vi "mainAuto.vi"() -> ()   [LabVIEW 2018]
uses:
  <vilib>/Analysis/baseanly.llb/Mean (DBL).vi
  #include/Global_usbComm.vi
  <userlib>/_OpenG.lib/array/array.llb/Filter 1D Array with Scalar (String)__ogtk.vi
  <userlib>/_OpenG.lib/array/array.llb/Filter 1D Array with Scalar (Boolean)__ogtk.vi
  <vilib>/Analysis/NI_AALBase.lvlib
panel:
  out "index 2":i32
  out "random 2":i32
  out "random":i32
  out "index":i32
  out "appended array":i16[](array[numeric])
  out "min(x,y)":i16
  out "max(x,y)":i16
  out "valueResistance":dbl
  out "resLower":dbl
  out "resUpper":dbl
  out "resistanceArray":dbl[](array[numeric])
  out "speedArray":dbl[](array[numeric])
  out "inclineArray":dbl[](array[numeric])
  out "negative incline":dbl
  out "FAN":string
  out "fanType":string
  out "refnum out":refnum<file>
  in  "Tab Control":T1(tab)
  out "Welcome to Console Test":picture
  out "Version":string[][](array[string])
  in  "Inspection Point":string(combo)
  in  "PO Line Number":string
  in  "PO Number":string
  in  "Inspector Name":string
  in  "Work Station":string
  in  "Vendor Name":string
  in  "Vendor Number":string
  out "Initialize Test":string
  out "Config and Fixture Setup":string
  out "Firmware Reference":string
  in  "EQF1259 com port":refnum<visa-resource-name>
  out "Console Number":string
  out "Console Name":string
  in  "scanSerial":string
  out "resultSerial":bool
  out "PartNumber":string
  in  "Cos0":bool
  in  "Cos1":bool
  out "COSMETIC-3, 4":string
  in  "Con1":bool
  out "FIXTURE_SETUP-1":string
  out "Connection":picture
  out "Voltage":string
  out "Power On":cluster{dbl, dbl}(graph)
  out "Current":string
  out "POWER_UP-5, 6":string
  in  "Pow0":bool
  in  "Pow1":bool
  out "PowerOn":bool
  out "CurrentOn":bool
  out "CurrentPeak":string
  out "limitON":bool
  out "CurrentMax":string
  out "PowerMode":string="Battery"
  out "BLE_SETUP-2":string
  out "BLE_CONNECT-7":string
  out "BLE PASS":bool
  out "Cal1":bool
  in  "Dis1":bool
  in  "Dis0":bool
  out "MAINTENANCE MODE-8, 9, 10, 11":string
  in  "Enter Firmware":string
  out "Firmware":bool
  in  "Key0":bool
  in  "Key1":bool
  out "SPM AEROBIC":dbl(knob) scale=0.0..200.0
  in  "stopP":bool
  out "SPEED":dbl(knob) scale=0.0..10.1
  out "MAX":string
  out "PWM_RPM":string
  out "SPEED AEROBIC":dbl(knob) scale=0.0..25.0
  out "RPM AEROBIC":dbl(knob) scale=0.0..200.0
  in  "Tac0":bool
  in  "Tac1":bool
  out "Quickspeed":bool
  out "Minus\nButton":bool
  out "Plus\nButton":bool
  out "ONE\nButton":bool
  out "PWM PASS":bool
  out "PWM hz":string
  out "PWM %":string
  out "Elapsed Time (s)":dbl
  out "Press Next":dbl format="%#_13g"
  out "Decrease":bool
  out "Increase":bool
  out "Least":bool
  out "RESISTANCE-15":string
  out "QuickResistance":bool
  out "RESISTANCE/CURRENT":cluster{dbl, dbl}(graph)
  out "IRun":string
  out "IPeak":string
  out "Press Next":dbl
  out "RESISTANCE PASS":bool
  out "overCurrent":bool
  in  "stopR":bool
  out "currentMaxResistance":string
  out "BLE PULSE":u32(graph)
  out "BLE_BPM":u32
  out "PULSE-17":string
  out "Hand/Thumb Pass":bool
  out "BLE_HRM Pass":bool
  in  "E-stopHRM":bool
  in  "PUL0":bool
  in  "PUL1":bool
  out "BLE Status":u32
  out "FanCurrent":dbl(graph)
  in  "FAN0":bool
  in  "FAN1":bool
  out "Ifan":string
  out "limitFan":bool
  out "currentMaxFan":string
  out "FAN-18":string
  out "fanIPeak":string
  in  "AUD0 2":bool
  in  "AUD1 2":bool
  out "Iaudio":string
  out "AudioCurrent":dbl(graph)
  in  "AUD0":bool
  out "currentMaxAudio":string
  out "AUDIO-19":string
  out "audioIPeak":string
  in  "AUD1":bool
  out "limitAudio":bool
  in  "TV1":bool
  in  "TV0":bool
  out "TVCurrent":dbl(graph)
  out "Itv":string
  out "limitTV":bool
  out "currentMaxTV":string
  out "TV-20":string
  out "tvIPeak":string
  out "limitUSB":bool
  out "Iusb":string
  in  "USB1":bool
  in  "USB0":bool
  out "currentMaxUSB":string
  out "USBCurrent":dbl(graph)
  out "USB-16":string
  out "usbIPeak":string
  in  "stopI":bool
  out "incline":dbl(graph)
  out "INCLINE PASS":bool
  out "INCLINE-14":string
  out "Quickincline":bool
  out "Down":bool
  out "Up":bool
  out "ZERO":bool
  out "MAX":dbl
  out "MIN":dbl
  out "Press Next":dbl
  out "limitCSafe":bool
  out "Icsafe":string
  in  "CSA1":bool
  in  "CSA0":bool
  out "currentMaxCSafe":string
  out "CSafeCurrent":dbl(graph)
  out "CSAFE-21":string
  out "csafeIPeak":string
  out "limitWahoo":bool
  out "Iwahoo":string
  in  "WAH1":bool
  in  "WAH0":bool
  out "currentMaxWahoo":string
  out "WahooCurrent":dbl(graph)
  out "WAHOO-22":string
  out "wahooIPeak":string
  in  "ANO0":bool
  in  "ANO1":bool
  out "Another":picture
  out "# of Samples":i32
  out "# of Failed Samples":i32
  out "# of Passed Samples":i32
  out "Failed":picture
  out "Test Log":string
  out "Goodbye!":picture
  out "standard notepad":string
  out "standard labviewdbupload":string
  in  "FIN0":bool
  out "FINISH-25":string
  # "Does Cosmetic Pass Inspection?"
  # "Scan Console Serial Number"
  # "Is The Harness Connected Correctly?"
  # "Did Console Power ON?"
  # "Calibrate?"
  # "Display?"
  # "Key Code?"
  # "Did The Hand/Thumb Pulse Pass?"
  # "Did The Fan Function Well?"
  # "BLE Audio"
  # "Aux Audio"
  # "NOT USED. SEE BLE CONNECT AND PULSE FOR DATA."
  # "Would You Like To Test Another Console?"
  # "Console Failed Test!"
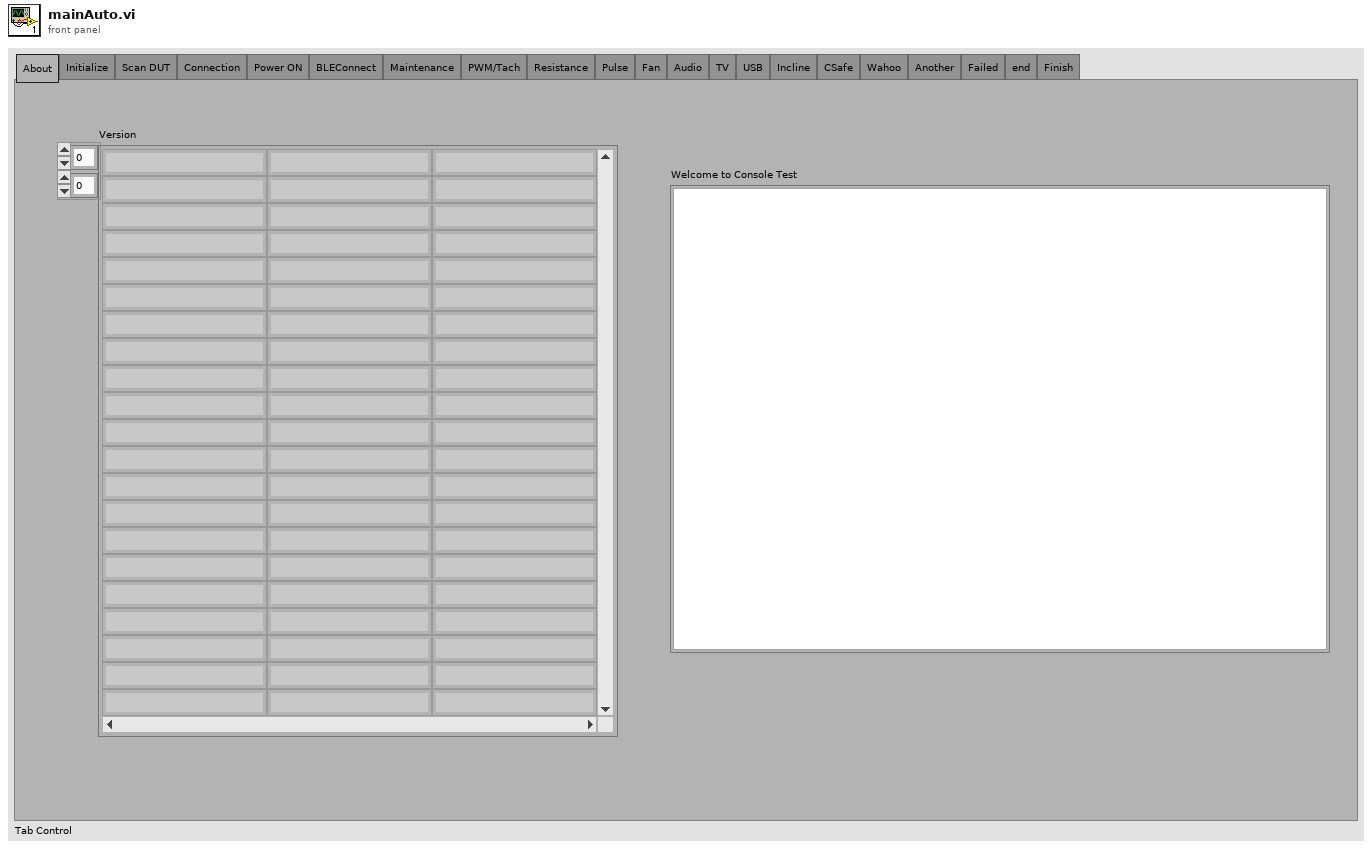
[diagram p1: front panel]
types:
  T1 = enum32{"About", "Initialize", "Scan DUT", "Connection", "Power ON", "BLEConnect", "Maintenance", "PWM/Tach", "Resistance", "Pulse", "Fan", "Audio", "TV", "USB", "Incline", "CSafe", "Wahoo", "Another", "Failed", "end", "Finish"}
  T2 = enum32{"Interactive applications", "Built-in command line utilities", "Executable command line utilities"}
  T3 = enum32{"About", "Initialize", "Scan DUT", "Connection", "Power ON", "BLEConnect", "Maintenance", "PWM/Tach", "Resistance", "Pulse", "Fan", "Audio", "TV", "USB", "Incline", "CSafe", "Wahoo", "Another", "Failed", "end"}
  T4 = enum16{"Flow", "User", "Station", "Vendor", "Number", "PO #", "PO Line#", "Record"}
  T5 = enum16{"name", "number", "device", "firmware", "mcu", "display", "grade", "resistance", "distance", "pulse"}
  T6 = enum16{"verifyHand_Thumb", "startBLE_HRM", "readBLE_HRM", "statusBLE_HRM"}
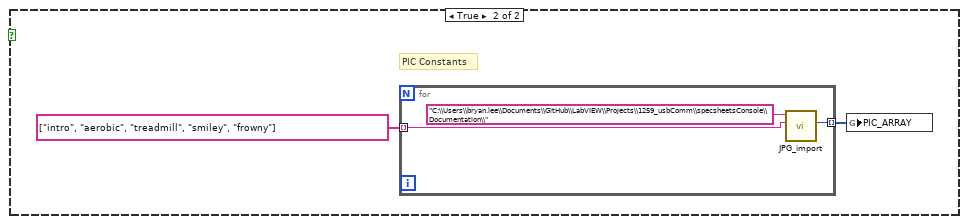
[diagram p3: hidden frame]
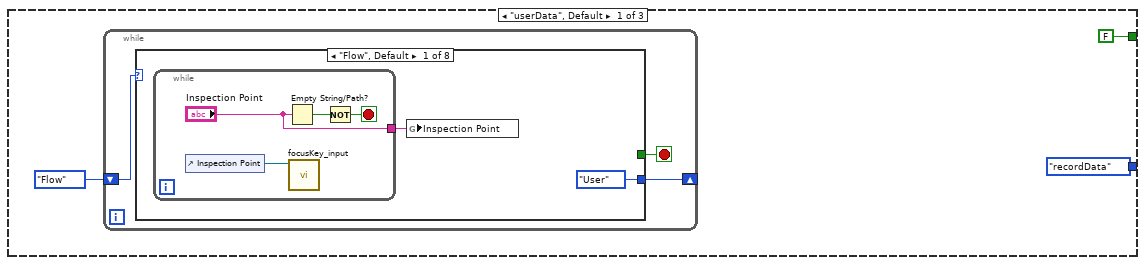
[diagram p5: hidden frame]
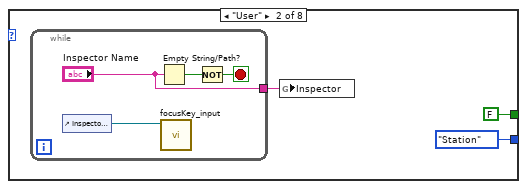
[diagram p6: hidden frame]
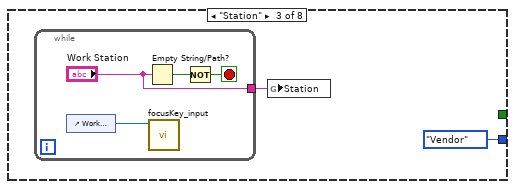
[diagram p7: hidden frame]
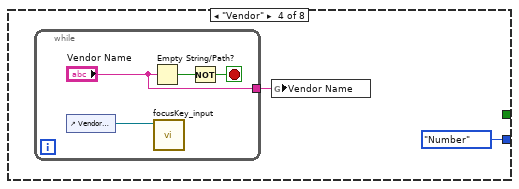
[diagram p8: hidden frame]
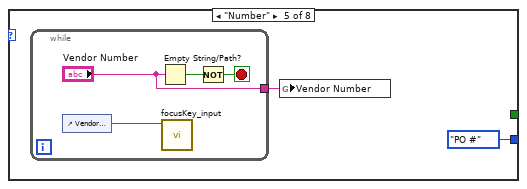
[diagram p9: hidden frame]
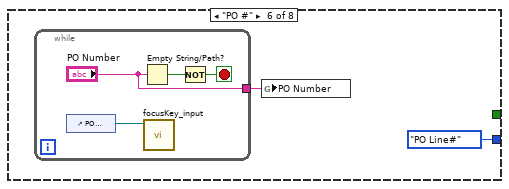
[diagram p10: hidden frame]
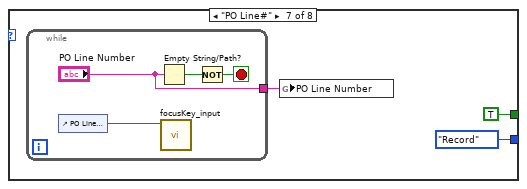
[diagram p11: hidden frame]
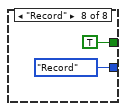
[diagram p12: hidden frame]
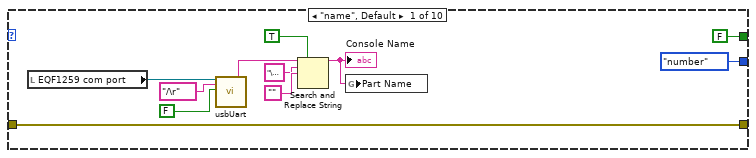
[diagram p13: hidden frame]
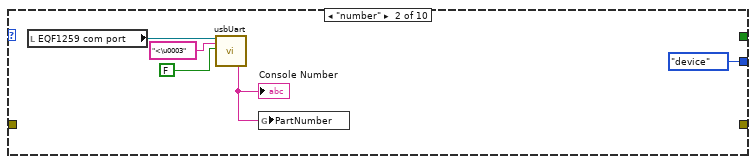
[diagram p14: hidden frame]
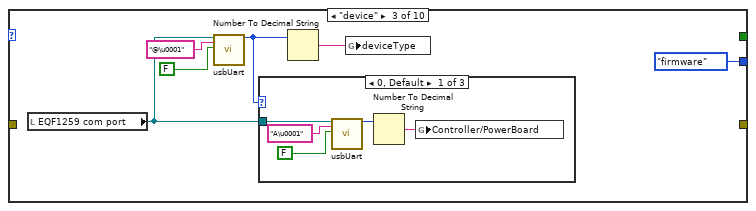
[diagram p15: hidden frame]
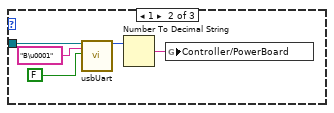
[diagram p16: hidden frame]
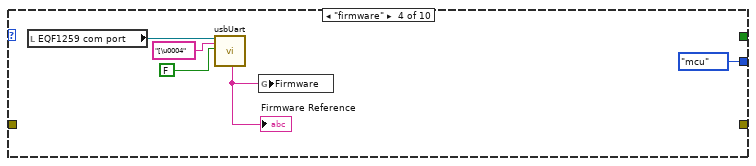
[diagram p18: hidden frame]
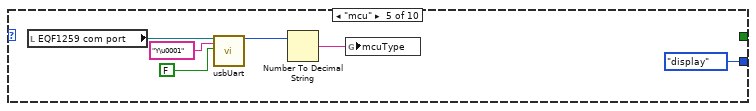
[diagram p19: hidden frame]
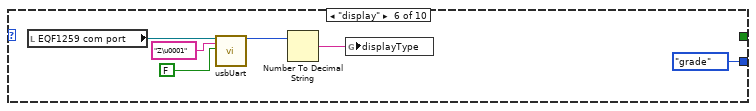
[diagram p20: hidden frame]
diagram:
  w1 = 0
  # "About\nInitialize\nScan DUT\nConnection\nPower On\nMaintenance\nSpeed/Distance\nIncline\nResistance\nFeatures\nExtra Features\nAnother\nFailed\nend"
  n1 = while {
    shift-right: [w3] -> _
    shift-left: "Tab Control" -> [w9]
    shift-right: [w5] -> _
    shift-left: w1 -> [w7]
    shift-right: [w4] -> _
    shift-left: w1 -> [w6]
    stop <- w10 stop-if-true
    n2 = property on="Tab Control" class="TabCtl (strict)"("Value"=w9) -> ("Value"=w8:T1)  [unwired: 2 in, 2 out]
    n3 = case shown="\"Audio\"" w8 {
      tunnel: [FALSE _ _ _ _ _ _ w524 w903 _ _ _ _ _ _ _ _ _ _ TRUE _] -> w10
      tunnel: [w13 T3."Connection" ("Tab Control") w217 w262 w298 w347 w413 w525 w905 w1347 w2236 w2355 w2467 w2608 w2670 w2715 w2756 w2793 T1."Finish" ("Tab Control") T3."end" ("Tab Control") w2854] -> w3
      tunnel: w7 -> [w12 w42 w210 w265 w292 w344 w410 w521 w900 w1343 w2230 w2342 w2462 w2601 w2664 w2704 w2749 w2784 w2805 w2814 w2856]
      tunnel: w6 -> [w11 w41 w215 w264 w291 w343 w409 w520 w894 w1342 w2229 w2341 w2461 w2600 w2663 w2711 w2748 w2783 w2807 w2813 w2855]
      tunnel: [w12 w42 w216 w265 w292 w344 w410 w521 w900 w1343 w2230 w2342 w2462 w2601 w2664 w2704 w2749 w2784 w2805 w2814 w2856] -> w5
      tunnel: [w11 w41 w215 w264 w291 w343 w409 w520 w894 w1342 w2229 w2341 w2461 w2600 w2663 w2711 w2748 w2783 w2806 w2813 w2855] -> w4
      frame "About", Default {
        n4 = for {
          N: 1 -> [_]
          w17 = FALSE ("Visible")
          w18 = 0
          n5 = global write "Global_usbComm.vi" "tempNumeric"(0.0 ("tempNumeric")) -> ()
          n6 = global write "Global_usbComm.vi" "tempBoolean"(FALSE) -> ()
          n7 = global write "Global_usbComm.vi" "tempString"("" ("tempString")) -> ()
          n8 = local write "# of Samples"(w18) -> ()
          n9 = local write "# of Failed Samples"(w18) -> ()
          n10 = case shown="False" FALSE {
            frame False {
              w28 = "\""
              # "Opens procedure"
              n11 = global read "Global_usbComm.vi" "PIC_ARRAY"() -> (w25:picture[])
              n12 = global read "Global_usbComm.vi" "Version"() -> (→"Version":string[][])
              n13 = Index Array(array=w25, index=0) -> (element=→"Welcome to Console Test":picture)
              n14 = call <vilib>:"Space Constant.vi"() -> ("String"=w30:string)
              n15 = Concatenate Strings("C:\\Windows\\System32\\notepad.exe" ("Command"), w30, w28, "C:\\specsheetsConsole\\Documentation\\Console(Chinese).txt" ("string"), w28) -> (w31:string)
              n16 = call "exeCLI.vi"("Tab Control"=T2."Interactive applications", "command line (interactive)"=w31) -> ()  [unwired: 11 in, 3 out]
            }
            frame True {
              # "PIC Constants"
              n17 = for {
                tunnel: [w35] -> w33 mode=indexing
                tunnel: string[] ["intro", "aerobic", "treadmill", "smiley", "frowny"] -> [w34] mode=indexing
                n18 = call "JPG_import.vi"("File name"=w34, "File path"="C:\\Users\\bryan.lee\\Documents\\GitHub\\LabVIEW\\Projects\\1259_usbComm\\specsheetsConsole\\Documentation\\") -> ("new picture"=w35:picture)  [unwired: 7 in, 2 out]
              }
              n19 = global write "Global_usbComm.vi" "PIC_ARRAY"(w33) -> ()
            }
          }
          n20 = property on="speedArray" class="Arr (strict)"("Visible"=w17) -> ()  [unwired: 2 in, 2 out]
          n21 = property on="resistanceArray" class="Arr (strict)"("Visible"=w17) -> ()  [unwired: 2 in, 2 out]
          n22 = property on="inclineArray" class="Arr (strict)"("Visible"=w17) -> ()  [unwired: 2 in, 2 out]
        }
        n23 = while {
          tunnel: [T3."Initialize" ("Tab Control")] -> w13
          stop <- TRUE stop-if-true
          n24 = Wait (ms)(milliseconds to wait=u32 1500) -> ()  [unwired: 1 out]
        }
      }
      frame "Initialize" {
        # "used for debugging"
        n25 = for {
          N: 2 -> [_]
          tunnel: [w48] -> w44
          w46 = ""
          n26 = local write "Work Station"(w46) -> ()
          n27 = global write "Global_usbComm.vi" "mcuType"(w46) -> ()
          n28 = global write "Global_usbComm.vi" "Controller/PowerBoard"(w46) -> ()
          n29 = global write "Global_usbComm.vi" "Firmware"(w46) -> ()
          n30 = global write "Global_usbComm.vi" "PartNumber"(w46) -> ()
          n31 = local write "Vendor Name"(w46) -> ()
          n32 = local write "Vendor Number"(w46) -> ()
          n33 = local write "PO Number"(w46) -> ()
          n34 = local write "PO Line Number"(w46) -> ()
          n35 = local write "Console Name"(w46) -> ()
          n36 = local write "Console Number"(w46) -> ()
          n37 = local write "Firmware Reference"(w46) -> ()
          n38 = global write "Global_usbComm.vi" "Part Name"(w46) -> ()
          n39 = global write "Global_usbComm.vi" "deviceType"(w46) -> ()
          n40 = local write "Inspector Name"(w46) -> ()
          n41 = local write "Inspection Point"(w46) -> ()
          n42 = local write "EQF1259 com port"(refnum<visa-resource-name> refnum ("VISA resource name")) -> ()
          n43 = call <vilib>:"Simple Error Handler.vi"() -> ("error out"=w48:errorcluster)  [unwired: 5 in, 4 out]
          "Initialize Test" <- "\u0006\\&^\tgMneöNvm\u0000i\u0000c\u0000r\u0000o\u0000S\u0000D\u0000ÒceQE\u0000Q\u0000F\u00001\u00002\u00005\u00009\u0000\u00020\n\u0000\u0000_/TE\u0000Q\u0000F\u00001\u00002\u00005\u00009\u0000\u00020\n\u0000(WE\u0000Q\u0000F\u00001\u00002\u00005\u00009\u0000\nN\fÿ\tébv^ R}cknxvMneöN\u00020\n\u0000(W\u000bNbvh<h\nNkXQáOo`\u00020\n\u0000\tébE\u0000Q\u0000F\u00001\u00002\u00005\u00009\u0000\u001a¯ïzãS\u00020\n\u0000I\u0000n\u0000s\u0000e\u0000r\u0000t\u0000 \u0000m\u0000i\u0000c\u0000r\u0000o\u0000S\u0000D\u0000 \u0000w\u0000i\u0000t\u0000h\u0000 \u0000p\u0000r\u0000o\u0000f\u0000i\u0000l\u0000e\u0000 \u0000i\u0000n\u0000t\u0000o\u0000 \u0000E\u0000Q\u0000F\u00001\u00002\u00005\u00009\u0000.\u0000\n\u0000T\u0000u\u0000r\u0000n\u0000 \u0000o\u0000n\u0000 \u0000E\u0000Q\u0000F\u00001\u00002\u00005\u00009\u0000.\u0000\n\u0000O\u0000n\u0000 \u0000t\u0000h\u0000e\u0000 \u0000E\u0000Q\u0000F\u00001\u00002\u00005\u00009\u0000,\u0000 \u0000s\u0000e\u0000l\u0000e\u0000c\u0000t\u0000 \u0000a\u0000n\u0000d\u0000 \u0000l\u0000o\u0000a\u0000d\u0000 \u0000t\u0000h\u0000e\u0000 \u0000c\u0000o\u0000r\u0000r\u0000e\u0000c\u0000t\u0000 \u0000c\u0000o\u0000n\u0000f\u0000i\u0000g\u0000u\u0000r\u0000a\u0000t\u0000i\u0000o\u0000n\u0000 \u0000f\u0000i\u0000l\u0000e\u0000.\u0000\n\u0000F\u0000i\u0000l\u0000l\u0000 \u0000o\u0000u\u0000t\u0000 \u0000t\u0000h\u0000e\u0000 \u0000i\u0000n\u0000f\u0000o\u0000r\u0000m\u0000a\u0000t\u0000i\u0000o\u0000n\u0000 \u0000o\u0000n\u0000 \u0000t\u0000h\u0000e\u0000 \u0000f\u0000o\u0000r\u0000m\u0000 \u0000b\u0000e\u0000l\u0000o\u0000w\u0000.\u0000\n\u0000S\u0000e\u0000l\u0000e\u0000c\u0000t\u0000 \u0000t\u0000h\u0000e\u0000 \u0000E\u0000Q\u0000F\u00001\u00002\u00005\u00009\u0000 \u0000c\u0000o\u0000m\u0000m\u0000u\u0000n\u0000i\u0000c\u0000a\u0000t\u0000i\u0000o\u0000n\u0000 \u0000p\u0000o\u0000r\u0000t\u0000.\u0000"
          "Config and Fixture Setup" <- "\u0006\\5un¿~Þ¥c0RE\u0000Q\u0000F\u00001\u00002\u00005\u00009\u0000\u00020\n\u0000¾nopwQMn\u001aÿ\n\u0000O(uP\u0000C\u0000\u0006\\.\u0000x\u0000m\u0000l\u0000MneöN R}0Rm\u0000i\u0000c\u0000r\u0000o\u0000S\u0000D\u0000aS-N\fÿåeöN(WR\u0000N\u0000D\u0000f\u0000t\u0000p\u0000-Nv§c6RðS\rTðy\u000bN~b0R\bÿOY\u001aÿ& R\u0000N\u0000D\u0000F\u0000t\u0000p\u0000 \u0000\\\u0000 \u0000E\u0000B\u0000N\u0000T\u00000\u00002\u00001\u00001\u00007\u0000 \u0000\\\u0000 \u0000P\u0000r\u0000o\u0000c\u0000e\u0000d\u0000u\u0000r\u0000e\u0000\tÿ\u00020\n\u0000\u0006\\m\u0000i\u0000c\u0000r\u0000o\u0000S\u0000D\u0000aSb\u001dg\nNÒceQm\u0000i\u0000c\u0000r\u0000o\u0000S\u0000D\u0000aSÒcýi-N\u00020\n\u0000Sb\u0000_opwQÌbvR\u0000E\u0000S\u0000E\u0000T\u0000\tc®\u00020\n\u0000O(u\u0011T\nNT\u0011T\u000bN\tc®~b0RcknxvMneöN\u00020\n\u0000\tcE\u0000N\u0000T\u0000E\u0000R\u0000\tébMneöN\bÿO\\U^1\u0000\tÿ\u00020\n\u0000S_O\\U^3z[öe\fÿ÷I{_5\u0000Òy\fÿY\u000bN@b:y\u00020\n\u0000¾n9YwQ\t²Q\u001aÿ\n\u0000\tcE\u0000Q\u0000F\u00001\u00002\u00005\u00009\u0000 \u00002\u0000x\u0000\nNvD\u0000i\u0000s\u0000p\u0000l\u0000a\u0000y\u0000\u00020\n\u0000(WdkopwQ\nN\tc\u0000_ËY\n\u0000O(u\u0011T\nNT\u0011T\u000bN\tc®¾n:g\t²Q\u00020\n\u0000(WopwQ\nN\tc\u0000_ËY\u00020\n\u0000\tc\u0000N!k>f:y\u00020\n\u0000C\u0000o\u0000n\u0000n\u0000e\u0000c\u0000t\u0000 \u0000t\u0000h\u0000e\u0000 \u0000p\u0000o\u0000w\u0000e\u0000r\u0000 \u0000..."
        }
        n44 = while {
          shift-right: [w52] -> _
          shift-left: enum16{"getData", "userData", "recordData"}."getData" -> [w54]
          tunnel: w44 -> [w51]
          stop <- w53 stop-if-true
          n45 = case shown="\"getData\"" w54 {
            tunnel: [FALSE FALSE TRUE] -> w53
            tunnel: [enum16{"getData", "userData", "recordData"}."recordData" enum16{"getData", "userData", "recordData"}."userData" enum16{"getData", "userData", "recordData"}."recordData"] -> w52
            tunnel: w51 -> [_ w109 _]
            frame "userData", Default {
              n46 = while {
                shift-right: [w58] -> _
                shift-left: T4."Flow" -> [w59]
                stop <- w60 stop-if-true
                n47 = case shown="\"Flow\", Default" w59 {
                  tunnel: [_ FALSE _ _ _ _ TRUE TRUE] -> w60
                  tunnel: [T4."User" T4."Station" T4."Vendor" T4."Number" T4."PO #" T4."PO Line#" T4."Record" T4."Record"] -> w58
                  frame "Flow", Default {
                    n48 = while {
                      tunnel: ["Inspection Point"] -> w62
                      stop <- w64 stop-if-true
                      n49 = control-ref of="Inspection Point"() -> (w66:refnum<vi>)
                      n50 = Empty String/Path?(string/path="Inspection Point") -> (empty?=w65:bool)
                      n51 = call "focusKey_input.vi"("reference"=w66) -> ()  [unwired: 10 in, 1 out]
                      n52 = Not(x=w65) -> (.not. x?=w64:bool)
                    }
                    n53 = global write "Global_usbComm.vi" "Inspection Point"(w62) -> ()
                  }
                  frame "User" {
                    n54 = while {
                      tunnel: ["Inspector Name"] -> w68
                      stop <- w72 stop-if-true
                      n55 = control-ref of="Inspector Name"() -> (w71:refnum<vi>)
                      n56 = Empty String/Path?(string/path="Inspector Name") -> (empty?=w73:bool)
                      n57 = call "focusKey_input.vi"("reference"=w71) -> ()  [unwired: 10 in, 1 out]
                      n58 = Not(x=w73) -> (.not. x?=w72:bool)
                    }
                    n59 = global write "Global_usbComm.vi" "Inspector"(w68) -> ()
                  }
                  frame "Station" {
                    n60 = while {
                      tunnel: ["Work Station"] -> w75
                      stop <- w78 stop-if-true
                      n61 = control-ref of="Work Station"() -> (w77:refnum<vi>)
                      n62 = Empty String/Path?(string/path="Work Station") -> (empty?=w79:bool)
                      n63 = call "focusKey_input.vi"("reference"=w77) -> ()  [unwired: 10 in, 1 out]
                      n64 = Not(x=w79) -> (.not. x?=w78:bool)
                    }
                    n65 = global write "Global_usbComm.vi" "Station"(w75) -> ()
                  }
                  frame "Vendor" {
                    n66 = while {
                      tunnel: ["Vendor Name"] -> w81
                      stop <- w84 stop-if-true
                      n67 = control-ref of="Vendor Name"() -> (w83:refnum<vi>)
                      n68 = Empty String/Path?(string/path="Vendor Name") -> (empty?=w85:bool)
                      n69 = call "focusKey_input.vi"("reference"=w83) -> ()  [unwired: 10 in, 1 out]
                      n70 = Not(x=w85) -> (.not. x?=w84:bool)
                    }
                    n71 = global write "Global_usbComm.vi" "Vendor Name"(w81) -> ()
                  }
                  frame "Number" {
                    n72 = while {
                      tunnel: ["Vendor Number"] -> w87
                      stop <- w90 stop-if-true
                      n73 = control-ref of="Vendor Number"() -> (w89:refnum<vi>)
                      n74 = Empty String/Path?(string/path="Vendor Number") -> (empty?=w91:bool)
                      n75 = call "focusKey_input.vi"("reference"=w89) -> ()  [unwired: 10 in, 1 out]
                      n76 = Not(x=w91) -> (.not. x?=w90:bool)
                    }
                    n77 = global write "Global_usbComm.vi" "Vendor Number"(w87) -> ()
                  }
                  frame "PO #" {
                    n78 = while {
                      tunnel: ["PO Number"] -> w93
                      stop <- w96 stop-if-true
                      n79 = control-ref of="PO Number"() -> (w95:refnum<vi>)
                      n80 = Empty String/Path?(string/path="PO Number") -> (empty?=w97:bool)
                      n81 = call "focusKey_input.vi"("reference"=w95) -> ()  [unwired: 10 in, 1 out]
                      n82 = Not(x=w97) -> (.not. x?=w96:bool)
                    }
                    n83 = global write "Global_usbComm.vi" "PO Number"(w93) -> ()
                  }
                  frame "PO Line#" {
                    n84 = while {
                      tunnel: ["PO Line Number"] -> w99
                      stop <- w102 stop-if-true
                      n85 = control-ref of="PO Line Number"() -> (w104:refnum<vi>)
                      n86 = Empty String/Path?(string/path="PO Line Number") -> (empty?=w103:bool)
                      n87 = call "focusKey_input.vi"("reference"=w104) -> ()  [unwired: 10 in, 1 out]
                      n88 = Not(x=w103) -> (.not. x?=w102:bool)
                    }
                    n89 = global write "Global_usbComm.vi" "PO Line Number"(w99) -> ()
                  }
                  frame "Record" {
                  }
                }
              }
            }
            frame "getData" {
              n90 = while {
                tunnel: [w113] -> w110
                tunnel: w109 -> [w112]
                stop <- w114 stop-if-true
                n91 = control-ref of="EQF1259 com port"() -> (w117:refnum<vi>)
                n92 = Empty String/Path?(string/path="EQF1259 com port") -> (empty?=w115:bool)
                n93 = call "focusKey_input.vi"("error in (no error)"=w112, "reference"=w117) -> ("error out"=w113:errorcluster)  [unwired: 9 in]
                n94 = Not(x=w115) -> (.not. x?=w114:bool)
              }
              n95 = while {
                shift-right: [w118] -> _
                shift-left: T5."name" -> [w119]
                shift-right: [w120] -> _
                shift-left: w110 -> [w121]
                stop <- w122 stop-if-true
                n96 = case shown="\"pulse\"" w119 {
                  tunnel: [FALSE _ _ _ _ _ _ _ _ TRUE] -> w122
                  tunnel: w121 -> [w130 _ _ _ _ _ _ _ _ _]
                  tunnel: [T5."number" T5."device" T5."firmware" T5."mcu" T5."display" T5."grade" T5."resistance" T5."distance" T5."pulse" T5."name"] -> w118
                  tunnel: [w130 _ _ _ _ _ _ _ _ _] -> w120
                  frame "name", Default {
                    n97 = local read "EQF1259 com port"() -> (w131:refnum<visa-resource-name>)
                    n98 = call "usbUart.vi"("VISA resource name"=w131, "write buffer"="/\r" ("write buffer buffer"), "sdFeature"=FALSE) -> ("valid byte"=w129:string)  [unwired: 1 in, 15 out]
                    n99 = Search and Replace String(replace all?=TRUE ("replace all? (F)"), input string=w129, search string="\u0000", replace string="") -> (result string=w126:string)  [unwired: 4 in, 3 out]
                    "Console Name" <- w126
                    n100 = global write "Global_usbComm.vi" "Part Name"(w126) -> ()
                  }
                  frame "number" {
                    n101 = local read "EQF1259 com port"() -> (w137:refnum<visa-resource-name>)
                    n102 = call "usbUart.vi"("VISA resource name"=w137, "write buffer"="<\u0003" ("write buffer buffer"), "sdFeature"=FALSE) -> ("PartNumber"=w136:string)  [unwired: 1 in, 15 out]
                    "Console Number" <- w136
                    n103 = global write "Global_usbComm.vi" "PartNumber"(w136) -> ()
                  }
                  frame "device" {
                    n104 = local read "EQF1259 com port"() -> (w140:refnum<visa-resource-name>)
                    n105 = call "usbUart.vi"("VISA resource name"=w140, "write buffer"="@\u0001" ("write buffer buffer"), "sdFeature"=FALSE) -> ("number[0]"=w141:u32)  [unwired: 1 in, 15 out]
                    n106 = case shown="0, Default" w141 {
                      tunnel: w140 -> [w146 w153 _]
                      frame 0, Default {
                        n107 = call "usbUart.vi"("VISA resource name"=w146, "write buffer"="A\u0001" ("write buffer buffer"), "sdFeature"=FALSE) -> ("number[0]"=w149:u32)  [unwired: 1 in, 15 out]
                        n108 = Number To Decimal String(number=w149) -> (decimal integer string=w148:string)  [unwired: 1 in]
                        n109 = global write "Global_usbComm.vi" "Controller/PowerBoard"(w148) -> ()
                      }
                      frame 1 {
                        n110 = call "usbUart.vi"("VISA resource name"=w153, "write buffer"="B\u0001", "sdFeature"=FALSE) -> ("number[0]"=w151:u32)  [unwired: 1 in, 15 out]
                        n111 = Number To Decimal String(number=w151) -> (decimal integer string=w152:string)  [unwired: 1 in]
                        n112 = global write "Global_usbComm.vi" "Controller/PowerBoard"(w152) -> ()
                      }
                      frame 3 {
                        # "Rower_Basic"
                      }
                    }
                    n113 = Number To Decimal String(number=w141) -> (decimal integer string=w144:string)  [unwired: 1 in]
                    n114 = global write "Global_usbComm.vi" "deviceType"(w144) -> ()
                  }
                  frame "firmware" {
                    n115 = local read "EQF1259 com port"() -> (w159:refnum<visa-resource-name>)
                    n116 = call "usbUart.vi"("VISA resource name"=w159, "write buffer"="[\u0004", "sdFeature"=FALSE) -> ("BB FW"=w155:string)  [unwired: 1 in, 15 out]
                    "Firmware Reference" <- w155
                    n117 = global write "Global_usbComm.vi" "Firmware"(w155) -> ()
                  }
                  frame "mcu" {
                    n118 = local read "EQF1259 com port"() -> (w163:refnum<visa-resource-name>)
                    n119 = call "usbUart.vi"("VISA resource name"=w163, "write buffer"="Y\u0001", "sdFeature"=FALSE) -> ("number[0]"=w165:u32)  [unwired: 1 in, 15 out]
                    n120 = Number To Decimal String(number=w165) -> (decimal integer string=w162:string)  [unwired: 1 in]
                    n121 = global write "Global_usbComm.vi" "mcuType"(w162) -> ()
                  }
                  frame "display" {
                    n122 = local read "EQF1259 com port"() -> (w168:refnum<visa-resource-name>)
                    n123 = call "usbUart.vi"("VISA resource name"=w168, "write buffer"="Z\u0001", "sdFeature"=FALSE) -> ("number[0]"=w171:u32)  [unwired: 1 in, 15 out]
                    n124 = Number To Decimal String(number=w171) -> (decimal integer string=w169:string)  [unwired: 1 in]
                    n125 = global write "Global_usbComm.vi" "displayType"(w169) -> ()
                  }
                  frame "grade" {
                    n126 = local read "EQF1259 com port"() -> (w173:refnum<visa-resource-name>)
                    n127 = call "usbUart.vi"("VISA resource name"=w173, "write buffer"=" \u0001", "sdFeature"=FALSE) -> ("number[0]"=w177:u32)  [unwired: 1 in, 15 out]
                    n128 = Number To Decimal String(number=w177) -> (decimal integer string=w175:string)  [unwired: 1 in]
                    n129 = global write "Global_usbComm.vi" "gradeType"(w175) -> ()
                  }
                  frame "resistance" {
                    n130 = local read "EQF1259 com port"() -> (w179:refnum<visa-resource-name>)
                    n131 = call "usbUart.vi"("VISA resource name"=w179, "write buffer"="¡\u0001", "sdFeature"=FALSE) -> ("number[0]"=w182:u32)  [unwired: 1 in, 15 out]
                    n132 = Number To Decimal String(number=w182) -> (decimal integer string=w183:string)  [unwired: 1 in]
                    n133 = global write "Global_usbComm.vi" "resistanceType"(w183) -> ()
                  }
                  frame "distance" {
                    n134 = local read "EQF1259 com port"() -> (w185:refnum<visa-resource-name>)
                    n135 = call "usbUart.vi"("VISA resource name"=w185, "write buffer"="›\u0001", "sdFeature"=FALSE) -> ("number[0]"=w189:u32)  [unwired: 1 in, 15 out]
                    n136 = Number To Decimal String(number=w189) -> (decimal integer string=w187:string)  [unwired: 1 in]
                    n137 = global write "Global_usbComm.vi" "distanceType"(w187) -> ()
                  }
                  frame "pulse" {
                    n138 = local read "EQF1259 com port"() -> (w192:refnum<visa-resource-name>)
                    n139 = call "usbUart.vi"("VISA resource name"=w192, "write buffer"="h\u0001", "sdFeature"=FALSE) -> ("number[0]"=w196:u32)  [unwired: 1 in, 15 out]
                    n140 = Number To Decimal String(number=w196) -> (decimal integer string=w194:string)  [unwired: 1 in]
                    n141 = global write "Global_usbComm.vi" "pulseType"(w194) -> ()
                  }
                }
              }
            }
            frame "recordData" {
              # "loads the feature array"
              n142 = local read "EQF1259 com port"() -> (w204:refnum<visa-resource-name>)
              n143 = call "usbUart.vi"("VISA resource name"=w204, "write buffer"="P\u0002", "sdFeature"=TRUE) -> ("error out"=w198:errorcluster)  [unwired: 1 in, 15 out]
              n144 = global read "Global_usbComm.vi" "Part Name"() -> (w200:string)
              n145 = call "Header data_Cnsl.vi"("base path"=path "C:/", "prompt (Create Folder)"="logsConsole", "file name"=w200, "Error In"=w198) -> ("refnum out"=→"refnum out":refnum<file>)  [unwired: 10 in, 1 out]
            }
          }
        }
      }
      frame "Scan DUT" {
        w213 = FALSE
        w220 = ""
        n146 = Increment(x=w210) -> (x+1=w216:i32)
        "# of Samples" <- w216
        n147 = local write "scanSerial"(w220) -> ()
        n148 = local write "PartNumber"(w220) -> ()
        n149 = local write "Cos0"(w213) -> ()
        n150 = local write "Cos1"(w213) -> ()
        n151 = local write "resultSerial"(w213) -> ()
        n152 = local read "refnum out"() -> (w211:refnum<file>)
        n153 = call "User data_Cnsl.vi"("refnum in"=w211) -> ("error out"=w212:errorcluster)  [unwired: 7 in, 1 out]
        n154 = call "cosmeticPIP.vi"("error in (no error)"=w212) -> ("error out"=w208:errorcluster)  [unwired: 10 in]
        n155 = flat-sequence {
          tunnel: w208 -> [w225]
          tunnel: [w225] -> w207
          frame #0 {
            n156 = global read "Global_usbComm.vi" "COSMETIC-3, 4"() -> (w222:string)
            n157 = Concatenate Strings(w222, "kbÏcïSeRagb_\u0001x\u0007h~{\u00020\n\u0000S\u0000c\u0000a\u0000n\u0000 \u0000t\u0000h\u0000e\u0000 \u0000p\u0000e\u0000e\u0000l\u0000a\u0000b\u0000l\u0000e\u0000 \u0000b\u0000a\u0000r\u0000c\u0000o\u0000d\u0000e\u0000 \u0000l\u0000a\u0000b\u0000e\u0000l\u0000.\u0000\n\u0000") -> (→"COSMETIC-3, 4":string)
          }
        }
        n158 = while {
          tunnel: [w259] -> w221
          tunnel: [w253] -> w214
          tunnel: w207 -> [w252]
          stop <- w260 stop-if-true
          n159 = control-ref of="scanSerial"() -> (w258:refnum<vi>)
          n160 = Empty String/Path?(string/path="scanSerial") -> (empty?=w261:bool)
          n161 = Search/Split String(string="scanSerial", offset (0)=6) -> (substring before match=w257:string)  [unwired: 1 in, 2 out]
          n162 = call "focusKey_input.vi"("error in (no error)"=w252, "reference"=w258) -> ("error out"=w259:errorcluster)  [unwired: 9 in]
          n163 = global read "Global_usbComm.vi" "PartNumber"() -> (w256:string)
          "PartNumber" <- w256
          n164 = Not(x=w261) -> (.not. x?=w260:bool)
          n165 = Equal?(x=w257, y=w256) -> (x = y?=w253:bool)
          "resultSerial" <- w253
        }
        n166 = case shown="True" w214 {
          tunnel: w221 -> [_ w232]
          tunnel: [FALSE w229] -> w209
          frame False {
          }
          frame True {
            n167 = flat-sequence {
              tunnel: w232 -> [w235]
              tunnel: [w234] -> w231
              tunnel: [w233] -> w230
              tunnel: w231 -> [_]
              tunnel: w230 -> [w243]
              tunnel: [w241] -> w227
              frame #0 {
                n168 = local read "scanSerial"() -> (w237:string)
                n169 = Reverse String(1:w237) -> (0:w239:string)
                n170 = Search/Split String(string=w239, offset (0)=11) -> (substring before match=w240:string)  [unwired: 1 in, 2 out]
                n171 = local read "refnum out"() -> (w233:refnum<file>)
                n172 = Reverse String(1:w240) -> (0:w236:string)
                n173 = call "Serial data.vi"("error in"=w235, "Serial Number"=w236, "refnum in"=w233) -> ("error out"=w234:errorcluster)  [unwired: 7 in, 1 out]
              }
              frame #1 {
                n174 = while {
                  tunnel: [w247] -> w242
                  stop <- w250 stop-if-true
                  n175 = Not(x="Cos0") -> (.not. x?=w251:bool)
                  n176 = Or(x="Cos1", y="Cos0") -> (x .or. y?=w250:bool)
                  n177 = And(x="Cos1", y=w251) -> (x .and. y?=w247:bool)
                }
                n178 = case shown="True" w242 {
                  selector: w242 -> [w244 w245]
                  tunnel: w243 -> [_ w246]
                  tunnel: [w244 w245] -> w241
                  frame False {
                  }
                  frame True {
                    n179 = call "Pass_Fail.vi"("OK"=w245, "Byte Stream File in"=w246) -> ()  [unwired: 8 in, 2 out]
                  }
                }
              }
            }
            n180 = And(x=TRUE, y=w227) -> (x .and. y?=w229:bool)
          }
        }
        n181 = Select(t=T3."Power ON" ("Tab Control"), s=w209, f=T3."Failed" ("Tab Control")) -> (s? t:f=w217:T3)
      }
      frame "Connection" {
        n182 = call "controllerVoltage.vi"() -> ("error out"=w263:errorcluster)  [unwired: 11 in]
        n183 = local write "Con1"(FALSE) -> ()
        n184 = call "controllerPIP.vi"("error in (no error)"=w263) -> ("error out"=w266:errorcluster)  [unwired: 10 in]
        n185 = global read "Global_usbComm.vi" "deviceType"() -> (w267:string)
        n186 = case shown="\"1\"" w267 {
          tunnel: w266 -> [_ _ _]
          frame "0", Default {
            n187 = global read "Global_usbComm.vi" "PIC_ARRAY"() -> (w269:picture[])
            n188 = global read "Global_usbComm.vi" "FIXTURE_SETUP-1"() -> (→"FIXTURE_SETUP-1":string)
            n189 = Index Array(array=w269, index=2) -> (element=→"Connection":picture)
          }
          frame "1" {
            n190 = global read "Global_usbComm.vi" "PIC_ARRAY"() -> (w275:picture[])
            n191 = global read "Global_usbComm.vi" "FIXTURE_SETUP-1"() -> (w276:string)
            n192 = Index Array(array=w275, index=1) -> (element=w273:picture)
            n193 = local write "FIXTURE_SETUP-1"(w276) -> ()
            n194 = local write "Connection"(w273) -> ()
          }
          frame "2" {
            n195 = global read "Global_usbComm.vi" "PIC_ARRAY"() -> (w279:picture[])
            n196 = global read "Global_usbComm.vi" "FIXTURE_SETUP-1"() -> (w280:string)
            n197 = Index Array(array=w279, index=1) -> (element=w277:picture)
            n198 = local write "FIXTURE_SETUP-1"(w280) -> ()
            n199 = local write "Connection"(w277) -> ()
          }
        }
        n200 = while {
          tunnel: [T3."Scan DUT" ("Tab Control")] -> w262
          stop <- "Con1" stop-if-true
        }
      }
      frame "Power ON" {
        w287 = "0.00" ("Voltage")
        w288 = FALSE
        # "current cannot be used as a stop due to battery option"
        n201 = local write "Voltage"(w287) -> ()
        n202 = local write "Current"(w287) -> ()
        n203 = local write "CurrentPeak"(w287) -> ()
        n204 = global write "Global_usbComm.vi" "runCurrent"(w287) -> ()
        n205 = local write "CurrentMax"(w287) -> ()
        n206 = local write "Pow1"(w288) -> ()
        n207 = local write "Pow0"(w288) -> ()
        n208 = property on="Power On" class="WFChart (strict)"("History Data"=cluster{dbl, dbl}[] []) -> ()  [unwired: 2 in, 2 out]
        n209 = local write "PowerMode"("Off" ("runCurrent")) -> ()
        n210 = global read "Global_usbComm.vi" "POWER_UP-5, 6"() -> (→"POWER_UP-5, 6":string)
        n211 = local write "CurrentOn"(w288) -> ()
        n212 = local write "limitON"(w288) -> ()
        n213 = local write "PowerOn"(w288) -> ()
        n214 = local read "EQF1259 com port"() -> (w283:refnum<visa-resource-name>)
        n215 = call "currentMax.vi"("VISA Refnum in"=w283) -> ("error out"=w289:errorcluster, "stringCurrentMax"=w284:string)  [unwired: 8 in, 1 out]
        n216 = global write "Global_usbComm.vi" "maxCurrent"(w284) -> ()
        n217 = while {
          tunnel: [w327] -> w297
          tunnel: w289 -> [w309]
          tunnel: [w323] -> w290
          tunnel: [w316] -> w286
          tunnel: w284 -> [w304]
          stop <- w328 stop-if-true
          n218 = local read "EQF1259 com port"() -> (w305:refnum<visa-resource-name>)
          n219 = call "usbUart.vi"("VISA resource name"=w305, "write buffer"="j\u0001", "sdFeature"=FALSE) -> ("number[0]"=w308:u32)  [unwired: 1 in, 15 out]
          n220 = case shown="0, Default" w308 {
            frame 0, Default {
              w329 = "Off" ("USB")
              n221 = local write "PowerMode"(w329) -> ()
              n222 = global write "Global_usbComm.vi" "PowerMode"(w329) -> ()
            }
            frame 1 {
              w330 = "On" ("USB")
              # "On"
              n223 = local read "limitON"() -> (w335:bool)
              n224 = local read "CurrentOn"() -> (w334:bool)
              n225 = local read "PowerOn"() -> (w333:bool)
              n226 = Not(x=w335) -> (.not. x?=w336:bool)
              n227 = Compound Arithmetic op=OR(TRUE, w333, w334, w336) -> (w331:bool)
              n228 = local write "PowerMode"(w330) -> ()
              n229 = global write "Global_usbComm.vi" "PowerMode"(w330) -> ()
              n230 = local write "Pow1"(w331) -> ()
            }
            frame 2 {
              w337 = "Battery" ("USB")
              # "Battery"
              n231 = global write "Global_usbComm.vi" "PowerMode"(w337) -> ()
              "PowerMode" <- w337
            }
          }
          n232 = global read "Global_usbComm.vi" "ConsoleVoltage"() -> (w302:string)
          n233 = call "voltageScan.vi"("error in (no error)"=w309, "VISA Refnum in"=w305) -> ("error out"=w321:errorcluster, "stringVoltage"=w316:string, "numberVoltage"=w315:dbl)  [unwired: 7 in]
          "Voltage" <- w316
          n234 = Fract/Exp String To Number(string=w302) -> (number=w301:dbl)  [unwired: 3 in, 1 out]
          n235 = call "currentScan.vi"("error in (no error)"=w321, "Imax"=w304, "VISA resource name"=w305) -> ("error out"=w320:errorcluster, "max"=w317:bool, "Istring"=w310:string, "Ichart"=w313:dbl)  [unwired: 5 in]
          "limitON" <- w317
          n236 = Greater?(x=w315, y=w301) -> (0:→"PowerOn":bool)
          n237 = Compound Arithmetic op=OR("Pow1", "Pow0", w317) -> (w328:bool)
          n238 = Not(x=w317) -> (.not. x?=w318:bool)
          n239 = Not(x="Pow0") -> (.not. x?=w325:bool)
          n240 = call "currentPeak.vi"("error in (no error)"=w320, "Istring# change"=w310, "Istring# scan"=w310) -> ("Ipeak"=w323:string, "Irun"=→"Current":string)  [unwired: 6 in, 1 out]
          "CurrentPeak" <- w323
          n241 = Bundle("numberVoltage"=w315, "Ichart"=w313) -> (→"Power On":cluster{"\nnumberVoltage":dbl, "Ichart":dbl})  [unwired: 1 in]
          n242 = Greater?(x=w313, y=0.0) -> (0:→"CurrentOn":bool)
          n243 = Compound Arithmetic op=AND(TRUE ("value"), w318, "Pow1", w325) -> (w327:bool)
          "CurrentMax" <- w304
        }
        n244 = local read "refnum out"() -> (w300:refnum<file>)
        n245 = call "dataSampled.vi"("Data"=w286, "refnum in"=w300) -> ("refnum out"=w299:refnum<file>)  [unwired: 8 in, 1 out]
        n246 = call "dataSampled.vi"("Data"=w290, "refnum in"=w299) -> ()  [unwired: 8 in, 2 out]
        n247 = Select(t=T3."Maintenance" ("Tab Control"), s=w297, f=T3."Failed" ("Tab Control")) -> (s? t:f=w298:T3)
      }
      frame "BLEConnect" {
        n248 = local write "BLE PASS"(FALSE ("BLE PASS")) -> ()
        n249 = global read "Global_usbComm.vi" "Inspection Point"() -> (w340:string)
        n250 = Equal?(x=w340, y="SubAssembly") -> (x = y?=w338:bool)
        n251 = case shown="False" w338 {
          tunnel: [TRUE w353] -> w342
          frame True {
            n252 = local read "refnum out"() -> (w348:refnum<file>)
            n253 = call "dataSampled.vi"("refnum in"=w348) -> ()  [unwired: 9 in, 2 out]
          }
          frame False {
            n254 = global read "Global_usbComm.vi" "WAHOO"() -> (w352:string)
            n255 = Not Equal?(x=w352, y="1") -> (x != y?=w350:bool)
            n256 = case shown="True" w350 {
              tunnel: [w354 w379] -> w353
              frame False {
                w358 = 2 ("index (row)")
                # "ANT+ SamplerApp"
                n257 = global read "Global_usbComm.vi" "PIP_Instruction"() -> (w361:string[][])
                n258 = global write "Global_usbComm.vi" "pulseType"("16" ("pulseType")) -> ()
                n259 = Index Array(array=w361, index (row) #1=w358, index (col) #1=w358, index (row) #2=w358, index (col) #2=7 ("disabled index (col)")) -> (element #1=w356:string, element #2=w357:string)
                n260 = global write "Global_usbComm.vi" "BLE_SETUP-2"(w356) -> ()
                n261 = local write "BLE_SETUP-2"(w356) -> ()
                n262 = global write "Global_usbComm.vi" "BLE_CONNECT-7"(w357) -> ()
                n263 = local write "BLE_CONNECT-7"(w357) -> ()
                n264 = while {
                  tunnel: [w373] -> w355
                  stop <- w371 stop-if-true
                  n265 = local read "EQF1259 com port"() -> (w366:refnum<visa-resource-name>)
                  n266 = call "usbUart.vi"("VISA resource name"=w366, "write buffer"="†\u0001") -> ("number[0]"=w368:u32)  [unwired: 2 in, 15 out]
                  n267 = Number To Decimal String(number=w368, width (-)=i16 0) -> (decimal integer string=w365:string)
                  n268 = Not Equal?(x=w365, y="0") -> (x != y?=w373:bool)
                  n269 = feedback #1() -> (w370:bool)  [unwired: 1 in]
                  n270 = call "Elapsed Time3"("Reset"=w370) -> ("Time has Elapsed"=w372:bool)  [unwired: 11 in, 7 out]
                  n271 = Or(x=w373, y=w372) -> (x .or. y?=w371:bool)
                  n272 = feedback-in #1(w371) -> ()
                }
                n273 = local write "BLE PASS"(w355) -> ()
                n274 = case shown="True" w355 {
                  selector: w355 -> [w362 w363]
                  tunnel: [w362 w363] -> w354
                  frame False {
                  }
                  frame True {
                    n275 = local read "refnum out"() -> (w364:refnum<file>)
                    n276 = call "Pass_Fail.vi"("OK"=w363, "Byte Stream File in"=w364) -> ()  [unwired: 8 in, 2 out]
                  }
                }
              }
              frame True {
                n277 = global read "Global_usbComm.vi" "TABLET"() -> (w377:string)
                n278 = Equal?(x=w377, y="0") -> (x = y?=w375:bool)
                n279 = case shown="True" w375 {
                  tunnel: [FALSE w381] -> w378
                  frame False {
                  }
                  frame True {
                    n280 = global read "Global_usbComm.vi" "BLE"() -> (w383:string)
                    n281 = Equal?(x=w383, y="1") -> (x = y?=w381:bool)
                  }
                }
                n282 = case shown="True" w378 {
                  tunnel: [TRUE w386] -> w379
                  frame False {
                    n283 = local read "refnum out"() -> (w385:refnum<file>)
                    n284 = call "dataSampled.vi"("refnum in"=w385) -> ()  [unwired: 9 in, 2 out]
                  }
                  frame True {
                    w388 = 1 ("index (row)")
                    # "BLE_CardioApp"
                    n285 = global read "Global_usbComm.vi" "PIP_Instruction"() -> (w393:string[][])
                    n286 = while {
                      tunnel: [w402] -> w387
                      stop <- w403 stop-if-true
                      n287 = local read "EQF1259 com port"() -> (w399:refnum<visa-resource-name>)
                      n288 = call "usbUart.vi"("VISA resource name"=w399, "write buffer"="†\u0001") -> ("binary[0] String"=w397:string)  [unwired: 2 in, 15 out]
                      n289 = Not Equal?(x="0" ("y"), y=w397) -> (x != y?=w402:bool)
                      n290 = feedback #2() -> (w401:bool)  [unwired: 1 in]
                      n291 = call "Elapsed Time2"("Reset"=w401) -> ("Time has Elapsed"=w404:bool)  [unwired: 11 in, 7 out]
                      n292 = Or(x=w402, y=w404) -> (x .or. y?=w403:bool)
                      n293 = feedback-in #2(w403) -> ()
                    }
                    "BLE PASS" <- w387
                    n294 = Index Array(array=w393, index (row) #1=w388, index (col) #1=2 ("disabled index (col)"), index (row) #2=w388, index (col) #2=7 ("disabled index (col)")) -> (element #1=w392:string, element #2=w391:string)
                    "BLE_SETUP-2" <- w392
                    "BLE_CONNECT-7" <- w391
                    n295 = global write "Global_usbComm.vi" "BLE_SETUP-2"(w392) -> ()
                    n296 = global write "Global_usbComm.vi" "BLE_CONNECT-7"(w391) -> ()
                    n297 = case shown="True" w387 {
                      selector: w387 -> [w394 w395]
                      tunnel: [w394 w395] -> w386
                      frame False {
                      }
                      frame True {
                        n298 = local read "refnum out"() -> (w396:refnum<file>)
                        n299 = call "Pass_Fail.vi"("OK"=w395, "Byte Stream File in"=w396) -> ()  [unwired: 8 in, 2 out]
                      }
                    }
                  }
                }
              }
            }
          }
        }
        n300 = Select(t=T3."PWM/Tach" ("Tab Control"), s=w342, f=T3."Failed" ("Tab Control")) -> (s? t:f=w347:T3)
      }
      frame "Maintenance" {
        w405 = ""
        w408 = FALSE
        (unwired) FALSE
        n301 = local write "Enter Firmware"(w405) -> ()
        n302 = global write "Global_usbComm.vi" "BaseCurrent"(w405) -> ()
        n303 = local write "Cal1"(w408) -> ()
        n304 = local write "Dis1"(w408) -> ()
        n305 = local write "Key0"(w408) -> ()
        n306 = local write "Key1"(w408) -> ()
        n307 = local write "Dis0"(w408) -> ()
        n308 = local write "Firmware"(w408) -> ()
        n309 = while {
          shift-right: [w416] -> _
          shift-left: 0 -> [w417]
          tunnel: [w414] -> w411
          stop <- w415 stop-if-true
          n310 = case shown="3" w417 {
            tunnel: [1 2 3 4 5 6 _] -> w416
            tunnel: [FALSE FALSE FALSE w446 w475 w489 w503] -> w415
            tunnel: [FALSE FALSE FALSE w447 w476 w490 w504] -> w414
            frame 0, Default {
              n311 = local read "EQF1259 com port"() -> (w419:refnum<visa-resource-name>)
              n312 = call "usbUart.vi"("VISA resource name"=w419, "write buffer"="\u0001", "sdFeature"=FALSE) -> ("PartNumber"=w428:string, "error out"=w418:errorcluster)  [unwired: 1 in, 14 out]
              n313 = global write "Global_usbComm.vi" "buttonType"(w428) -> ()
              n314 = call "usbUart.vi"("VISA resource name"=w419, "write buffer"="š\u0001", "sdFeature"=FALSE, "error in (no error)"=w418) -> ("PartNumber"=w422:string)  [unwired: 15 out]
              n315 = global write "Global_usbComm.vi" "tabletType"(w422) -> ()
            }
            frame 1 {
              n316 = global read "Global_usbComm.vi" "GRADE"() -> (w432:string)
              n317 = case shown="\"0\"" w432 {
                frame "1", Default {
                  n318 = property on="Cal1" class="Bool (strict)"("Visible"=TRUE) -> ()  [unwired: 2 in, 2 out]
                }
                frame "0" {
                  n319 = local write "Cal1"(TRUE) -> ()
                  n320 = property on="Cal1" class="Bool (strict)"("Visible"=FALSE) -> ()  [unwired: 2 in, 2 out]
                }
              }
              n321 = call "maintenancePIP.vi"() -> ("MAINTENANCE MODE-8, 9, 10, 11"=→"MAINTENANCE MODE-8, 9, 10, 11":string)  [unwired: 10 in, 1 out]
            }
            frame 2 {
              n322 = while {
                tunnel: ["Enter Firmware"] -> w439
                stop <- w444 stop-if-true
                n323 = control-ref of="Enter Firmware"() -> (w443:refnum<vi>)
                n324 = Empty String/Path?(string/path="Enter Firmware") -> (empty?=w445:bool)
                n325 = call "focusKey_input.vi"("reference"=w443) -> ()  [unwired: 10 in, 1 out]
                n326 = Not(x=w445) -> (.not. x?=w444:bool)
                "Firmware" <- w444
              }
              n327 = local read "refnum out"() -> (w440:refnum<file>)
              n328 = call "dataSampled.vi"("Data"=w439, "refnum in"=w440) -> ()  [unwired: 8 in, 2 out]
            }
            frame 3 {
              n329 = local read "Cal1"() -> (w448:bool)
              n330 = case shown="False" w448 {
                tunnel: [FALSE w463] -> w447
                tunnel: [FALSE w462] -> w446
                frame True {
                  # "This is 1 second / per 10 samples"
                  n331 = while {
                    tunnel: [w461] -> w453 mode=indexing
                    i -> [w459]
                    stop <- w460 stop-if-true
                    n332 = local read "EQF1259 com port"() -> (w457:refnum<visa-resource-name>)
                    n333 = Equal?(x=25, y=w459) -> (x = y?=w460:bool)
                    n334 = call "currentScan.vi"("VISA resource name"=w457) -> ("Ichart"=w461:dbl)  [unwired: 7 in, 3 out]
                  }
                  n335 = local read "refnum out"() -> (w456:refnum<file>)
                  n336 = call-poly <vilib>:"Mean.vi"("X"=w453) -> ("mean"=w452:dbl)  [unwired: 1 out]
                  n337 = call "dataSampled.vi"("refnum in"=w456) -> ()  [unwired: 9 in, 2 out]
                  n338 = Number To Fractional String(number=w452, precision (6)=i16 2) -> (F-format string=w451:string)  [unwired: 2 in]
                  n339 = global write "Global_usbComm.vi" "BaseCurrent"(w451) -> ()
                }
                frame False {
                  n340 = flat-sequence {
                    tunnel: [w465] -> w464
                    tunnel: w464 -> [w469]
                    tunnel: [w468] -> w463
                    tunnel: [w467] -> w462
                    frame #0 {
                      # "engineer mode on fixture"
                      n341 = local read "EQF1259 com port"() -> (w466:refnum<visa-resource-name>)
                      n342 = call "inclineCalibrate.vi"("VISA Refnum in"=w466) -> ("Complete"=w465:bool)  [unwired: 8 in, 2 out]
                    }
                    frame #1 {
                      n343 = case shown="False" w469 {
                        selector: w469 -> [w471 w473]
                        tunnel: [w471 w473] -> w468
                        tunnel: [w470 w472] -> w467
                        frame False {
                          n344 = Not(x=w471) -> (.not. x?=w470:bool)
                        }
                        frame True {
                          n345 = Not(x=w473) -> (.not. x?=w472:bool)
                          n346 = local read "refnum out"() -> (w474:refnum<file>)
                          n347 = call "Pass_Fail.vi"("OK"=w473, "Byte Stream File in"=w474) -> ()  [unwired: 8 in, 2 out]
                        }
                      }
                      "Cal1" <- w469
                    }
                  }
                }
              }
            }
            frame 4 {
              n348 = while {
                tunnel: [w487] -> w477
                stop <- w486 stop-if-true
                n349 = Not(x="Dis0") -> (.not. x?=w488:bool)
                n350 = Or(x="Dis1", y="Dis0") -> (x .or. y?=w486:bool)
                n351 = And(x="Dis1", y=w488) -> (x .and. y?=w487:bool)
              }
              n352 = case shown="True" w477 {
                selector: w477 -> [w479 w482]
                tunnel: [w479 w482] -> w476
                tunnel: [w480 w481] -> w475
                frame False {
                  n353 = Not(x=w479) -> (.not. x?=w480:bool)
                }
                frame True {
                  n354 = Not(x=w482) -> (.not. x?=w481:bool)
                  n355 = local read "refnum out"() -> (w483:refnum<file>)
                  n356 = call "Pass_Fail.vi"("OK"=w482, "Byte Stream File in"=w483) -> ()  [unwired: 8 in, 2 out]
                }
              }
            }
            frame 5 {
              n357 = while {
                tunnel: [w501] -> w491
                stop <- w500 stop-if-true
                n358 = Not(x="Key0") -> (.not. x?=w502:bool)
                n359 = Or(x="Key1", y="Key0") -> (x .or. y?=w500:bool)
                n360 = And(x="Key1", y=w502) -> (x .and. y?=w501:bool)
              }
              n361 = case shown="True" w491 {
                selector: w491 -> [w494 w496]
                tunnel: [w494 w496] -> w490
                tunnel: [w493 w495] -> w489
                frame False {
                  n362 = Not(x=w494) -> (.not. x?=w493:bool)
                }
                frame True {
                  n363 = Not(x=w496) -> (.not. x?=w495:bool)
                  n364 = local read "refnum out"() -> (w497:refnum<file>)
                  n365 = call "Pass_Fail.vi"("OK"=w496, "Byte Stream File in"=w497) -> ()  [unwired: 8 in, 2 out]
                }
              }
            }
            frame 6 {
              n366 = while {
                tunnel: [w509] -> w504
                tunnel: [w508] -> w503
                stop <- w508 stop-if-true
                n367 = local read "Key1"() -> (w507:bool)
                n368 = local read "Cal1"() -> (w506:bool)
                n369 = local read "Dis1"() -> (w511:bool)
                n370 = Compound Arithmetic op=AND(TRUE ("value"), w506, w511, w507) -> (w509:bool)
                n371 = Not(x=w509) -> (.not. x?=w510:bool)
                n372 = Or(x=w509, y=w510) -> (x .or. y?=w508:bool)
              }
            }
          }
        }
        n373 = Select(t=T3."BLEConnect" ("Tab Control"), s=w411, f=T3."Failed" ("Tab Control")) -> (s? t:f=w413:T3)
      }
      frame "PWM/Tach" {
        w516 = 0.0 ("Press Next")
        w518 = FALSE ("stop")
        n374 = local write "SPEED"(w516) -> ()
        n375 = local write "Plus\nButton"(w518) -> ()
        n376 = local write "Minus\nButton"(w518) -> ()
        n377 = local write "Quickspeed"(w518) -> ()
        n378 = local write "ONE\nButton"(w518) -> ()
        n379 = local write "PWM PASS"(w518) -> ()
        n380 = local write "speedArray"(dbl[] [0.0] ("Array")) -> ()
        n381 = local write "Press Next"(w516) -> ()
        n382 = global read "Global_usbComm.vi" "deviceType"() -> (w514:string)
        n383 = Decimal String To Number(string=w514) -> (number=w515:i32)  [unwired: 2 in, 1 out]
        n384 = Not Equal To 0?(x=w515) -> (x != 0?=w513:bool)
        n385 = case shown="True" w513 {
          tunnel: ["0" "1"] -> w512
          frame False {
            # "Treadmill"
          }
          frame True {
            # "Aerobic"
          }
        }
        n386 = case shown="\"0\", Default" w512 {
          tunnel: [w543 w601] -> w519
          tunnel: [w542 FALSE ("E-Stop")] -> w524
          frame "1" {
            w537 = 0.0 ("SPEED AEROBIC")
            w538 = FALSE ("Visible")
            w536 = TRUE
            w544 = FALSE ("Visible")
            # "Aerobic"
            # "Quick_Keys"
            n387 = property on="MAX" class="Str"("Visible"=w538) -> ()  [unwired: 2 in, 2 out]
            n388 = property on="speedArray" class="Arr (strict)"("Visible"=w538) -> ()  [unwired: 2 in, 2 out]
            n389 = property on="Quickspeed" class="Bool (strict)"("Visible"=w538) -> ()  [unwired: 2 in, 2 out]
            n390 = property on="ONE\nButton" class="Bool (strict)"("Visible"=w538) -> ()  [unwired: 2 in, 2 out]
            n391 = property on="PWM PASS" class="Bool (strict)"("Visible"=w538) -> ()  [unwired: 2 in, 2 out]
            n392 = property on="Plus\nButton" class="Bool (strict)"("Visible"=w538) -> ()  [unwired: 2 in, 2 out]
            n393 = property on="Press Next" class="DigNum (strict)"("Visible"=w538) -> ()  [unwired: 2 in, 2 out]
            n394 = property on="Minus\nButton" class="Bool (strict)"("Visible"=w538) -> ()  [unwired: 2 in, 2 out]
            n395 = property on="PWM hz" class="Str"("Visible"=w538) -> ()  [unwired: 2 in, 2 out]
            n396 = property on="PWM %" class="Str"("Visible"=w538) -> ()  [unwired: 2 in, 2 out]
            n397 = property on="SPEED" class="Knob (strict)"("Visible"=FALSE) -> ()  [unwired: 2 in, 2 out]
            n398 = property on="RPM AEROBIC" class="Knob (strict)"("Visible"=w536) -> ()  [unwired: 2 in, 2 out]
            n399 = property on="SPEED AEROBIC" class="Knob (strict)"("Visible"=w536) -> ()  [unwired: 2 in, 2 out]
            n400 = property on="Tac1" class="Bool (strict)"("Visible"=w536) -> ()  [unwired: 2 in, 2 out]
            n401 = property on="Tac0" class="Bool (strict)"("Visible"=w536) -> ()  [unwired: 2 in, 2 out]
            n402 = local write "Tac1"(w544) -> ()
            n403 = local write "Tac0"(w544) -> ()
            n404 = for {
              N: 1 -> [_]
              tunnel: [w553] -> w530
              tunnel: [w550] -> w529
              n405 = call "pwm_rpmPIP.vi"() -> ("error out"=w551:errorcluster, "PWM_RPM"=w554:string)  [unwired: 10 in]
              n406 = local read "EQF1259 com port"() -> (w552:refnum<visa-resource-name>)
              n407 = local write "PWM_RPM"(w554) -> ()
              n408 = Wait (ms)(milliseconds to wait=u32 250) -> ()  [unwired: 1 out]
              n409 = call "speedSet.vi"("error in (no error)"=w551, "VISA resource name"=w552) -> ("error out (no error)"=w550:errorcluster, "Running"=w553:bool)  [unwired: 2 in, 6 out]
            }
            n410 = property on="SPM AEROBIC" class="Knob (strict)"("Visible"=w536) -> ()  [unwired: 2 in, 2 out]
            n411 = local write "RPM AEROBIC"(w537) -> ()
            n412 = local write "SPEED AEROBIC"(w537) -> ()
            n413 = local write "SPM AEROBIC"(w537) -> ()
            n414 = while {
              tunnel: [w563] -> w540
              tunnel: [w562] -> w541
              tunnel: [w559] -> w543
              tunnel: [w558] -> w542
              shift-right: [w556] -> _
              shift-left: w530 -> [w557]
              tunnel: w529 -> [_]
              tunnel: [w555] -> w531
              stop <- w561 stop-if-true
              n415 = feedback #3() -> (w560:bool)  [unwired: 1 in]
              n416 = case shown="True" w557 {
                tunnel: [w566 w581] -> w561
                tunnel: [w564 w584] -> w563
                tunnel: [w564 w583] -> w562
                tunnel: w560 -> [_ w582]
                tunnel: [w566 w576] -> w559
                tunnel: [w566 FALSE ("E-Stop")] -> w558
                tunnel: [TRUE TRUE] -> w556
                tunnel: [w564 w570] -> w555
                frame False {
                  w564 = ""
                  w566 = FALSE
                  n417 = local read "EQF1259 com port"() -> (w569:refnum<visa-resource-name>)
                  n418 = call "usbCommand.vi"("write buffer"="\u0005\u0004", "VISA resource name in"=w569) -> ()  [unwired: 8 in, 2 out]
                  n419 = Wait (ms)(milliseconds to wait=u32 250) -> ()  [unwired: 1 out]
                }
                frame True {
                  n420 = call "Elapsed Time"("Reset"=w582) -> ("Elapsed Time (s)"=→"Elapsed Time (s)":dbl, "Time has Elapsed"=w575:bool)  [unwired: 11 in, 6 out]
                  n421 = local read "EQF1259 com port"() -> (w587:refnum<visa-resource-name>)
                  n422 = call "speedSet.vi"("VISA resource name"=w587) -> ("spm"=w570:string, "rpm"=w583:string, "speed"=w584:string, "RPM"=→"RPM AEROBIC":dbl, "SPEED"=→"SPEED AEROBIC":dbl, "SPM"=→"SPM AEROBIC":dbl)  [unwired: 3 in, 2 out]
                  n423 = Or(x="Tac1", y="Tac0") -> (x .or. y?=w577:bool)
                  n424 = Not(x="Tac0") -> (.not. x?=w580:bool)
                  n425 = And(x="Tac1", y=w580) -> (x .and. y?=w576:bool)
                  n426 = Compound Arithmetic op=OR(w577, w575) -> (w581:bool)
                }
              }
              n427 = feedback-in #3(w561) -> ()
            }
            n428 = local read "refnum out"() -> (w547:refnum<file>)
            n429 = call "dataSampled.vi"("Data"=w540, "refnum in"=w547) -> ("error out"=w546:errorcluster, "refnum out"=w548:refnum<file>)  [unwired: 8 in]
            n430 = call "dataSampled.vi"("Error In"=w546, "Data"=w541, "refnum in"=w548) -> ("error out"=w533:errorcluster, "refnum out"=w532:refnum<file>)  [unwired: 7 in]
            n431 = call "dataSampled.vi"("Error In"=w533, "Data"=w531, "refnum in"=w532) -> ("error out"=w534:errorcluster, "refnum out"=w535:refnum<file>)  [unwired: 7 in]
            n432 = for {
              N: 7 -> [_]
              tunnel: w535 -> [w589]
              tunnel: w534 -> [w588]
              n433 = call "dataSampled.vi"("Error In"=w588, "refnum in"=w589) -> ()  [unwired: 8 in, 2 out]
            }
          }
          frame "0", Default {
            w591 = FALSE
            w597 = TRUE ("Visible")
            # "Treadmill"
            # "No E-STOP"
            n434 = property on="RPM AEROBIC" class="Knob (strict)"("Visible"=w591) -> ()  [unwired: 2 in, 2 out]
            n435 = property on="Tac1" class="Bool (strict)"("Visible"=w591) -> ()  [unwired: 2 in, 2 out]
            n436 = property on="Tac0" class="Bool (strict)"("Visible"=w591) -> ()  [unwired: 2 in, 2 out]
            n437 = property on="Elapsed Time (s)" class="DigNum (strict)"("Visible"=w591) -> ()  [unwired: 2 in, 2 out]
            n438 = property on="SPEED AEROBIC" class="Knob (strict)"("Visible"=w591) -> ()  [unwired: 2 in, 2 out]
            n439 = property on="MAX" class="Str"("Visible"=w597) -> ()  [unwired: 2 in, 2 out]
            n440 = property on="PWM PASS" class="Bool (strict)"("Visible"=w597) -> ()  [unwired: 2 in, 2 out]
            n441 = property on="Press Next" class="DigNum (strict)"("Visible"=w597) -> ()  [unwired: 2 in, 2 out]
            n442 = property on="Plus\nButton" class="Bool (strict)"("Visible"=w597) -> ()  [unwired: 2 in, 2 out]
            n443 = property on="Quickspeed" class="Bool (strict)"("Visible"=w597) -> ()  [unwired: 2 in, 2 out]
            n444 = property on="ONE\nButton" class="Bool (strict)"("Visible"=w597) -> ()  [unwired: 2 in, 2 out]
            n445 = property on="SPEED" class="Knob (strict)"("Visible"=w597) -> ()  [unwired: 2 in, 2 out]
            n446 = property on="Minus\nButton" class="Bool (strict)"("Visible"=w597) -> ()  [unwired: 2 in, 2 out]
            n447 = property on="PWM hz" class="Str"("Visible"=w597) -> ()  [unwired: 2 in, 2 out]
            n448 = property on="PWM %" class="Str"("Visible"=w597) -> ()  [unwired: 2 in, 2 out]
            n449 = property on="SPM AEROBIC" class="Knob (strict)"("Visible"=w591) -> ()  [unwired: 2 in, 2 out]
            n450 = for {
              N: 2 -> [_]
              tunnel: [w845] -> w599
              tunnel: [w844] -> w600
              tunnel: [w841] -> w592
              n451 = flat-sequence {
                tunnel: [w848] -> w839
                tunnel: [w847] -> w838
                tunnel: [w855] -> w840
                tunnel: w839 -> [w856]
                tunnel: w838 -> [w855]
                tunnel: [w852] -> w837
                tunnel: [w851] -> w836
                tunnel: [w863] -> w843
                tunnel: [w862] -> w842
                tunnel: w840 -> [w861]
                tunnel: w837 -> [w860]
                tunnel: w836 -> [w859]
                tunnel: [w887] -> w845
                tunnel: [w883] -> w844
                tunnel: w843 -> [w883]
                tunnel: w842 -> [w882]
                tunnel: [w882] -> w841
                frame #0 {
                  n452 = local read "EQF1259 com port"() -> (w848:refnum<visa-resource-name>)
                  n453 = call "usbUart.vi"("VISA resource name"=w848, "write buffer"="E\u0001", "sdFeature"=FALSE) -> ("PartNumber"=w847:string)  [unwired: 1 in, 15 out]
                  n454 = global write "Global_usbComm.vi" "unitType"(w847) -> ()
                  n455 = Wait (ms)(milliseconds to wait=u32 250) -> ()  [unwired: 1 out]
                }
                frame #1 {
                  n456 = call "usbUart.vi"("VISA resource name"=w856, "write buffer"="v\u0002", "sdFeature"=FALSE) -> ("maxSpeed"=w851:string)  [unwired: 1 in, 15 out]
                  n457 = Fract/Exp String To Number(string=w851) -> (number=w852:dbl)  [unwired: 3 in, 1 out]
                  n458 = Wait (ms)(milliseconds to wait=u32 250) -> ()  [unwired: 1 out]
                }
                frame #2 {
                  n459 = case shown="\"1\", Default" w861 {
                    tunnel: w860 -> [w873 _]
                    tunnel: w859 -> [_ w881]
                    tunnel: [w867 w878] -> w863
                    tunnel: [w866 w877] -> w862
                    frame "1", Default {
                      # "euro"
                      n460 = local read "EQF1259 com port"() -> (w869:refnum<visa-resource-name>)
                      n461 = Multiply(x=w873, y=1.60934) -> (x*y=w871:dbl)
                      n462 = Number To Fractional String(number=w871, precision (6)=i16 1) -> (F-format string=w870:string)  [unwired: 2 in]
                      "MAX" <- w870
                      n463 = global write "Global_usbComm.vi" "MaxSpeed"(w870) -> ()
                      n464 = call "parseQuickKey.vi"("VISA resource name"=w869, "write buffer"="«\u0003", "y"=1, "x"=0) -> ("lengthString"=w867:i32, "KeyCodeName"=w866:string[])  [unwired: 11 in, 3 out]
                    }
                    frame "2" {
                      # "dom"
                      n465 = global write "Global_usbComm.vi" "MaxSpeed"(w881) -> ()
                      n466 = local write "MAX"(w881) -> ()
                      n467 = local read "EQF1259 com port"() -> (w880:refnum<visa-resource-name>)
                      n468 = call "parseQuickKey.vi"("VISA resource name"=w880, "write buffer"="©\u0002", "y"=0, "x"=0) -> ("lengthString"=w878:i32, "KeyCodeName"=w877:string[])  [unwired: 11 in, 3 out]
                    }
                  }
                  n469 = Wait (ms)(milliseconds to wait=u32 250) -> ()  [unwired: 1 out]
                }
                frame #3 {
                  n470 = global read "Global_usbComm.vi" "MaxSpeed"() -> (w885:string)
                  n471 = Fract/Exp String To Number(string=w885) -> (number=w884:dbl)  [unwired: 3 in, 1 out]
                  n472 = property on="SPEED" class="Knob (strict)"("Scale.Maximum"=w884) -> ()  [unwired: 2 in, 2 out]
                  n473 = call "pwm_rpmPIP.vi"() -> ("error out"=w887:errorcluster, "PWM_RPM"=→"PWM_RPM":string)  [unwired: 10 in]
                }
              }
            }
            n474 = for {
              N: 3 -> [_]
              tunnel: w599 -> [w835]
              tunnel: [w834] -> w590
              # "Speed, RPM, and SPM"
              n475 = local read "refnum out"() -> (w833:refnum<file>)
              n476 = call "dataSampled.vi"("Error In"=w835, "refnum in"=w833) -> ("error out"=w834:errorcluster)  [unwired: 8 in, 1 out]
            }
            n477 = global read "Global_usbComm.vi" "Inspection Point"() -> (w596:string)
            n478 = Equal?(x=w596, y="SubAssembly") -> (x = y?=w593:bool)
            n479 = case shown="True" w593 {
              tunnel: w590 -> [_ w730]
              tunnel: [w607 w729] -> w601
              tunnel: w600 -> [_ w728]
              tunnel: w592 -> [w605 w727]
              frame True {
                # "sub assembly"
                n480 = local write "PWM_RPM"("(W§c6RðS\nN\fÿYg*gÐL\fÿ÷\tcS\u0000T\u0000A\u0000R\u0000T\u0000\n\u0000(W§c6RðS\nN\fÿ\tc\tN\u000bN\u0000N*NvQ\u0000u\u0000i\u0000c\u0000k\u0000 \u0000s\u0000p\u0000e\u0000e\u0000d\u0000\bÿë_\u001f\u001f¦^\tÿ\tc®\fÿ6q\u000eTI{_Ó~gôv0R\u0007c:yopÝO\u0001c¹p®N\u00020\n\u0000(W§c6RðS\nN\fÿ\tc\u0000gNOv\u001c ë_\u001f\u001f¦^\u001d \tc®\u00020\n\u0000\n\u0000O\u0000n\u0000 \u0000t\u0000h\u0000e\u0000 \u0000c\u0000o\u0000n\u0000s\u0000o\u0000l\u0000e\u0000,\u0000 \u0000p\u0000r\u0000e\u0000s\u0000s\u0000 \u0000S\u0000T\u0000A\u0000R\u0000T\u0000 \u0000i\u0000f\u0000 \u0000n\u0000o\u0000t\u0000 \u0000r\u0000u\u0000n\u0000n\u0000i\u0000n\u0000g\u0000\n\u0000O\u0000n\u0000 \u0000t\u0000h\u0000e\u0000 \u0000c\u0000o\u0000n\u0000s\u0000o\u0000l\u0000e\u0000,\u0000 \u0000p\u0000r\u0000e\u0000s\u0000s\u0000 \u0000n\u0000e\u0000x\u0000t\u0000 \u0000Q\u0000u\u0000i\u0000c\u0000k\u0000 \u0000s\u0000p\u0000e\u0000e\u0000d\u0000 \u0000b\u0000u\u0000t\u0000t\u0000o\u0000n\u0000 \u0000o\u0000f\u0000 \u0000t\u0000h\u0000r\u0000e\u0000e\u0000 \u0000a\u0000n\u0000d\u0000 \u0000w\u0000a\u0000i\u0000t\u0000 \u0000f\u0000o\u0000r\u0000 \u0000r\u0000e\u0000s\u0000u\u0000l\u0000t\u0000s\u0000 \u0000t\u0000i\u0000l\u0000l\u0000 \u0000i\u0000n\u0000d\u0000i\u0000c\u0000a\u0000t\u0000o\u0000r\u0000 \u0000r\u0000e\u0000m\u0000a\u0000i\u0000n\u0000s\u0000 \u0000l\u0000i\u0000t\u0000.\u0000\n\u0000O\u0000n\u0000 \u0000t\u0000h\u0000e\u0000 \u0000c\u0000o\u0000n\u0000s\u0000o\u0000l\u0000e\u0000,\u0000 \u0000p\u0000r\u0000e\u0000s\u0000s\u0000 \u0000t\u0000h\u0000e\u0000 \u0000l\u0000o\u0000w\u0000e\u0000s\u0000t\u0000 \u0000Q\u0000u\u0000i\u0000c\u0000k\u0000 \u0000s\u0000p\u0000e\u0000e\u0000d\u0000 \u0000b\u0000u\u0000t\u0000t\u0000o\u0000n\u0000.\u0000") -> ()
                n481 = call-poly <userlib>:"Filter 1D Array__ogtk.vi"("items to filter"="", "array"=w605) -> ("filtered array"=w603:string[])  [unwired: 4 in, 1 out]
                n482 = flat-sequence {
                  tunnel: w603 -> [w608]
                  tunnel: [w723] -> w607
                  frame #0 {
                    n483 = while {
                      shift-right: [w612] -> _
                      shift-left: 0 -> [w613]
                      tunnel: w608 -> [w610]
                      stop <- w611 stop-if-true
                      n484 = case shown="1" w613 {
                        tunnel: [1 _] -> w612
                        tunnel: [FALSE TRUE] -> w611
                        tunnel: w610 -> [w614 _]
                        frame 0, Default {
                          n485 = while {
                            shift-right: [w619] -> _
                            shift-left: 0 -> [w620]
                            tunnel: w614 -> [w618]
                            stop <- w621 stop-if-true
                            n486 = case shown="0, Default" w620 {
                              tunnel: [FALSE FALSE TRUE] -> w621
                              tunnel: [w622 w646 2 ("f")] -> w619
                              tunnel: w618 -> [_ w645 _]
                              frame 0, Default {
                                n487 = for {
                                N: 2 -> [_]
                                tunnel: [w641] -> w640 mode=indexing
                                n488 = Random Number (0-1)() -> (number: 0 to 1=w644:dbl)
                                n489 = Multiply(x=w644, y=10.0) -> (x*y=w642:dbl)
                                n490 = To Word Integer(number=w642) -> (16bit integer=w641:i16)
                                }
                                n491 = Index Array(array=w640, index #1=0 ("index"), index #2=1 ("index")) -> (element #1=w638:i16, element #2=w639:i16)
                                n492 = Max & Min(x=w638, y=w639) -> (max(x,y)=w628:i16, min(x,y)=w634:i16)
                                "max(x,y)" <- w628
                                "min(x,y)" <- w634
                                n493 = Not Equal?(x=w628, y=w634) -> (x != y?=w632:bool)
                                n494 = Greater Or Equal?(x=i16 8 ("y"), y=w628) -> (x >= y?=w630:bool)
                                n495 = Greater Or Equal?(x=w634, y=i16 3) -> (x >= y?=w631:bool)
                                n496 = Compound Arithmetic op=AND(TRUE ("value"), w630, w632, w631) -> (w623:bool)
                                n497 = Select(t=1, s=w623, f=0) -> (s? t:f=w622:i32)
                              }
                              frame 1 {
                                n498 = for {
                                tunnel: w645 -> [w671] mode=indexing
                                tunnel: [w668] -> w658 mode=indexing
                                n499 = local read "max(x,y)"() -> (w667:i16)
                                n500 = Number To Decimal String(number=w667, width (-)=i16 0) -> (decimal integer string=w669:string)
                                n501 = Equal?(x=w671, y=w669) -> (x = y?=w668:bool)
                                }
                                n502 = for {
                                tunnel: w645 -> [w666] mode=indexing
                                tunnel: [w663] -> w655 mode=indexing
                                n503 = local read "min(x,y)"() -> (w662:i16)
                                n504 = Number To Decimal String(number=w662, width (-)=i16 0) -> (decimal integer string=w664:string)
                                n505 = Equal?(x=w666, y=w664) -> (x = y?=w663:bool)
                                }
                                n506 = call-poly <userlib>:"Filter 1D Array__ogtk.vi"("items to filter"=FALSE, "array"=w658) -> ("filtered array"=w657:bool[])  [unwired: 4 in, 1 out]
                                n507 = call-poly <userlib>:"Filter 1D Array__ogtk.vi"("items to filter"=FALSE, "array"=w655) -> ("filtered array"=w656:bool[])  [unwired: 4 in, 1 out]
                                n508 = Index Array(array=w657, index=0) -> (element=w659:bool)
                                n509 = Index Array(array=w656, index=0) -> (element=w660:bool)
                                n510 = Compound Arithmetic op=AND(TRUE ("value"), w659, w660) -> (w661:bool)
                                n511 = Select(t=2, s=w661, f=0) -> (s? t:f=w646:i32)
                              }
                              frame 2 {
                                n512 = local read "max(x,y)"() -> (w676:i16)
                                n513 = local read "min(x,y)"() -> (w675:i16)
                                n514 = Build Array(w676, w675, i16 1) -> (→"appended array":i16[])
                              }
                            }
                          }
                        }
                        frame 1 {
                          n515 = local read "appended array"() -> (w678:i16[])
                          n516 = for {
                            N: 3 -> [_]
                            tunnel: w678 -> [w683]
                            i -> [w682]
                            n517 = while {
                              tunnel: w683 -> [w699]
                              tunnel: w682 -> [w698]
                              tunnel: [w693] -> w681
                              i -> [w694]
                              stop <- w693 stop-if-true
                              n518 = Index Array(array=w699, index=w698) -> (element=w697:i16)
                              n519 = To Double Precision Float(number=w697) -> (double precision float=w696:dbl)
                              n520 = local write "Press Next"(w696) -> ()
                              n521 = Equal?(x=w694, y=1) -> (x = y?=w693:bool)
                            }
                            n522 = case shown="True" w681 {
                              frame False {
                              }
                              frame True {
                                n523 = while {
                                stop <- w689 stop-if-true
                                w692 = 0.5
                                n524 = local read "EQF1259 com port"() -> (w684:refnum<visa-resource-name>)
                                n525 = local read "Press Next"() -> (w686:dbl)
                                n526 = Add(x=w686, y=w692) -> (x+y=w691:dbl)
                                n527 = Subtract(x=w686, y=w692) -> (x-y=w690:dbl)
                                n528 = call "speedAquire.vi"("VISA resource name"=w684) -> ("SPEED"=w685:dbl)  [unwired: 6 in, 4 out]
                                n529 = local write "SPEED"(w685) -> ()
                                n530 = local read "stopP"() -> (w688:bool)
                                n531 = In Range and Coerce(upper limit=w691, x=w685, lower limit=w690) -> (In Range?=w687:bool)  [unwired: 1 out]
                                n532 = Or(x=w687, y=w688) -> (x .or. y?=w689:bool)
                                n533 = local write "Quickspeed"(w687) -> ()
                                }
                              }
                            }
                          }
                        }
                      }
                      n534 = local write "ONE\nButton"(w611) -> ()
                    }
                  }
                  frame #1 {
                    n535 = local read "refnum out"() -> (w717:refnum<file>)
                    n536 = global read "Global_usbComm.vi" "MaxSpeed"() -> (w716:string)
                    n537 = local read "EQF1259 com port"() -> (w712:refnum<visa-resource-name>)
                    n538 = call "dataSampled.vi"("Data"=w716, "refnum in"=w717) -> ("error out"=w713:errorcluster, "refnum out"=w718:refnum<file>)  [unwired: 8 in]
                    n539 = call "usbUart.vi"("VISA resource name"=w712, "write buffer"="t\u0002", "sdFeature"=FALSE, "error in (no error)"=w713) -> ("BB FW"=w708:string, "error out"=w710:errorcluster)  [unwired: 14 out]
                    n540 = local read "Quickspeed"() -> (w715:bool)
                    n541 = call "decimalAdd.vi"("Error In"=w710, "Frequency/PWM%"=w708, "refnum in"=w718) -> ("error out"=w709:errorcluster, "concatenated string"=w714:string, "refnum out"=w711:refnum<file>)  [unwired: 6 in]
                    n542 = local write "PWM hz"(w714) -> ()
                    n543 = call "Pass_Fail.vi"("error in (no error)"=w709, "OK"=w715, "Byte Stream File in"=w711) -> ("error out"=w707:errorcluster, "Byte Stream File out"=w702:refnum<file>)  [unwired: 7 in]
                    n544 = local read "ONE\nButton"() -> (w700:bool)
                    n545 = for {
                      N: 3 -> [_]
                      tunnel: w707 -> [w722]
                      tunnel: [w721] -> w703
                      tunnel: w702 -> [w720]
                      tunnel: [w719] -> w701
                      n546 = call "dataSampled.vi"("Error In"=w722, "refnum in"=w720) -> ("error out"=w719:errorcluster, "refnum out"=w721:refnum<file>)  [unwired: 8 in]
                    }
                    n547 = call "Pass_Fail.vi"("error in (no error)"=w701, "OK"=w700, "Byte Stream File in"=w703) -> ()  [unwired: 7 in, 2 out]
                  }
                  frame #2 {
                    n548 = local read "Quickspeed"() -> (w724:bool)
                    n549 = local read "ONE\nButton"() -> (w725:bool)
                    n550 = Compound Arithmetic op=AND(w724, w725, TRUE) -> (w723:bool)
                    n551 = local write "PWM PASS"(w723) -> ()
                  }
                }
              }
              frame False {
                # "vendor assembly"
                n552 = flat-sequence {
                  tunnel: w728 -> [w732]
                  tunnel: w730 -> [_]
                  tunnel: w727 -> [w733]
                  tunnel: [w830] -> w729
                  frame #0 {
                    n553 = for {
                      N: w732 -> [_]
                      tunnel: w733 -> [w740]
                      tunnel: [w736] -> w731 mode=indexing
                      i -> [w739]
                      n554 = Index Array(array=w740, index=w739) -> (element=w734:string)
                      n555 = Empty String/Path?(string/path=w734) -> (empty?=w738:bool)
                      n556 = Not(x=w738) -> (.not. x?=w737:bool)
                      n557 = case shown="True" w737 {
                        tunnel: [FALSE TRUE] -> w735
                        tunnel: w734 -> [_ w744]
                        frame False {
                        }
                        frame True {
                          n558 = Fract/Exp String To Number(string=w744) -> (number=→"Press Next":dbl)  [unwired: 3 in, 1 out]
                          n559 = Wait (ms)(milliseconds to wait=u32 1250) -> ()  [unwired: 1 out]
                        }
                      }
                      n560 = case shown="True" w735 {
                        tunnel: [_ w746] -> w736
                        frame False {
                        }
                        frame True {
                          n561 = while {
                            tunnel: [w751] -> w746
                            stop <- w749 stop-if-true
                            w752 = 0.5 ("x")
                            n562 = local read "EQF1259 com port"() -> (w753:refnum<visa-resource-name>)
                            n563 = local read "Press Next"() -> (w750:dbl)
                            n564 = Add(x=w752, y=w750) -> (x+y=w755:dbl)
                            n565 = Subtract(x=w750, y=w752) -> (x-y=w754:dbl)
                            n566 = call "speedAquire.vi"("VISA resource name"=w753) -> ("SPEED"=w751:dbl)  [unwired: 6 in, 4 out]
                            "SPEED" <- w751
                            n567 = In Range and Coerce(upper limit=w755, x=w751, lower limit=w754) -> (In Range?=w747:bool)  [unwired: 1 out]
                            "Quickspeed" <- w747
                            n568 = Or(x=w747, y="stopP") -> (x .or. y?=w749:bool)
                          }
                        }
                      }
                    }
                    "speedArray" <- w731
                  }
                  frame #1 {
                    n569 = flat-sequence {
                      tunnel: [w765] -> w760
                      tunnel: [w766] -> w759
                      tunnel: [w764] -> w756
                      tunnel: [w778] -> w761
                      tunnel: w760 -> [w778]
                      tunnel: w759 -> [w777]
                      tunnel: [w777] -> w758
                      tunnel: [w776] -> w757
                      tunnel: w756 -> [w776]
                      tunnel: w761 -> [w783]
                      tunnel: w758 -> [w782]
                      tunnel: w757 -> [w781]
                      frame #0 {
                        n570 = local read "EQF1259 com port"() -> (w764:refnum<visa-resource-name>)
                        n571 = local read "refnum out"() -> (w771:refnum<file>)
                        n572 = global read "Global_usbComm.vi" "MaxSpeed"() -> (w770:string)
                        n573 = call "dataSampled.vi"("Data"=w770, "refnum in"=w771) -> ("error out"=w769:errorcluster)  [unwired: 8 in, 1 out]
                        n574 = call "usbUart.vi"("VISA resource name"=w764, "write buffer"="t\u0002", "sdFeature"=FALSE, "error in (no error)"=w769) -> ("BB FW"=w774:string, "error out"=w768:errorcluster)  [unwired: 14 out]
                        n575 = call "decimalAdd.vi"("Error In"=w768, "Frequency/PWM%"=w774, "refnum in"=w771) -> ("error out"=w773:errorcluster, "concatenated string"=→"PWM hz":string, "refnum out"=w767:refnum<file>)  [unwired: 6 in]
                        n576 = local read "Quickspeed"() -> (w763:bool)
                        n577 = call "Pass_Fail.vi"("error in (no error)"=w773, "OK"=w763, "Byte Stream File in"=w767) -> ("error out"=w766:errorcluster, "Byte Stream File out"=w765:refnum<file>)  [unwired: 7 in]
                      }
                      frame #1 {
                        n578 = Wait (ms)(milliseconds to wait=u32 1000) -> ()  [unwired: 1 out]
                      }
                      frame #2 {
                        n579 = call "usbUart.vi"("VISA resource name"=w781, "write buffer"="r\u0002", "sdFeature"=FALSE, "error in (no error)"=w782) -> ("BB FW"=w785:string, "error out"=w787:errorcluster)  [unwired: 14 out]
                        n580 = call "decimalAdd.vi"("Error In"=w787, "Frequency/PWM%"=w785, "refnum in"=w783) -> ("concatenated string"=→"PWM %":string)  [unwired: 6 in, 2 out]
                      }
                    }
                  }
                  frame #2 {
                    n581 = while {
                      tunnel: [w793] -> w788
                      stop <- w794 stop-if-true
                      n582 = local read "EQF1259 com port"() -> (w795:refnum<visa-resource-name>)
                      n583 = global read "Global_usbComm.vi" "MaxSpeed"() -> (w799:string)
                      n584 = call "speedAquire.vi"("VISA resource name"=w795) -> ("KPH/MPH"=w801:string)  [unwired: 6 in, 4 out]
                      n585 = Fract/Exp String To Number(string=w799) -> (number=w798:dbl)  [unwired: 3 in, 1 out]
                      n586 = Fract/Exp String To Number(string=w801) -> (number=w800:dbl)  [unwired: 3 in, 1 out]
                      n587 = Subtract(x=w798, y=1.0) -> (x-y=w796:dbl)
                      n588 = local write "SPEED"(w800) -> ()
                      n589 = local read "stopP"() -> (w790:bool)
                      n590 = Equal?(x=w800, y=w796) -> (x = y?=w792:bool)
                      n591 = Or(x=w790, y=w792) -> (x .or. y?=w794:bool)
                      n592 = Not(x=w790) -> (.not. x?=w791:bool)
                      n593 = And(x=w792, y=w791) -> (x .and. y?=w793:bool)
                    }
                    "Minus\nButton" <- w788
                    n594 = local read "refnum out"() -> (w789:refnum<file>)
                    n595 = call "Pass_Fail.vi"("OK"=w788, "Byte Stream File in"=w789) -> ()  [unwired: 8 in, 2 out]
                  }
                  frame #3 {
                    n596 = while {
                      tunnel: [w806] -> w802
                      stop <- w807 stop-if-true
                      n597 = local read "EQF1259 com port"() -> (w809:refnum<visa-resource-name>)
                      n598 = global read "Global_usbComm.vi" "MaxSpeed"() -> (w813:string)
                      n599 = call "speedAquire.vi"("VISA resource name"=w809) -> ("KPH/MPH"=w815:string)  [unwired: 6 in, 4 out]
                      n600 = Fract/Exp String To Number(string=w813) -> (number=w811:dbl)  [unwired: 3 in, 1 out]
                      n601 = Fract/Exp String To Number(string=w815) -> (number=w814:dbl)  [unwired: 3 in, 1 out]
                      n602 = Subtract(x=w811, y=0.5) -> (x-y=w812:dbl)
                      n603 = local write "SPEED"(w814) -> ()
                      n604 = local read "stopP"() -> (w805:bool)
                      n605 = Equal?(x=w814, y=w812) -> (x = y?=w804:bool)
                      n606 = Or(x=w804, y=w805) -> (x .or. y?=w807:bool)
                      n607 = Not(x=w805) -> (.not. x?=w808:bool)
                      n608 = And(x=w804, y=w808) -> (x .and. y?=w806:bool)
                    }
                    "Plus\nButton" <- w802
                    n609 = local read "refnum out"() -> (w803:refnum<file>)
                    n610 = call "Pass_Fail.vi"("OK"=w802, "Byte Stream File in"=w803) -> ()  [unwired: 8 in, 2 out]
                  }
                  frame #4 {
                    n611 = local read "EQF1259 com port"() -> (w816:refnum<visa-resource-name>)
                    n612 = while {
                      tunnel: [w820] -> w817
                      tunnel: w816 -> [w826]
                      stop <- w821 stop-if-true
                      n613 = call "speedAquire.vi"("VISA resource name"=w826) -> ("KPH/MPH"=w827:string)  [unwired: 6 in, 4 out]
                      n614 = Fract/Exp String To Number(string=w827) -> (number=w824:dbl)  [unwired: 3 in, 1 out]
                      n615 = local write "SPEED"(w824) -> ()
                      n616 = local read "stopP"() -> (w823:bool)
                      n617 = Less?(x=w824, y=2.0) -> (x < y?=w819:bool)
                      n618 = Not(x=w823) -> (.not. x?=w822:bool)
                      n619 = Or(x=w823, y=w819) -> (x .or. y?=w821:bool)
                      n620 = And(x=w819, y=w822) -> (x .and. y?=w820:bool)
                    }
                    "ONE\nButton" <- w817
                    n621 = local read "refnum out"() -> (w818:refnum<file>)
                    n622 = call "Pass_Fail.vi"("OK"=w817, "Byte Stream File in"=w818) -> ()  [unwired: 8 in, 2 out]
                  }
                  frame #5 {
                    n623 = local read "Minus\nButton"() -> (w831:bool)
                    n624 = local read "ONE\nButton"() -> (w828:bool)
                    n625 = local read "Plus\nButton"() -> (w832:bool)
                    n626 = Compound Arithmetic op=AND(w831, w832, w828, TRUE ("value")) -> (w830:bool)
                    "PWM PASS" <- w830
                  }
                }
              }
            }
          }
        }
        n627 = Select(t=T3."Pulse" ("Tab Control"), s=w519, f=T3."Failed" ("Tab Control")) -> (s? t:f=w525:T3)
      }
      frame "Incline" {
        w893 = FALSE ("Visible")
        n628 = local write "negative incline"(0.0 ("negative incline")) -> ()
        n629 = local write "Up"(w893) -> ()
        n630 = local write "Down"(w893) -> ()
        n631 = local write "ZERO"(w893) -> ()
        n632 = local write "stopI"(w893) -> ()
        n633 = local write "inclineArray"(dbl[] []) -> ()
        n634 = property on="incline" class="WFChart (strict)"("History Data"=dbl[] []) -> ()  [unwired: 2 in, 2 out]
        n635 = local write "INCLINE PASS"(w893) -> ()
        n636 = local write "Quickincline"(w893) -> ()
        n637 = global read "Global_usbComm.vi" "gradeType"() -> (w899:string)
        n638 = Equal?(x=w899, y="0") -> (x = y?=w891:bool)
        n639 = case shown="False" w891 {
          tunnel: [FALSE w1328] -> w892
          frame True {
          }
          frame False {
            n640 = global read "Global_usbComm.vi" "gradeType"() -> (w1331:string)
            n641 = Decimal String To Number(string=w1331) -> (number=w1330:i32)  [unwired: 2 in, 1 out]
            n642 = Greater Or Equal?(x=w1330, y=2) -> (x >= y?=w1328:bool)
          }
        }
        n643 = global read "Global_usbComm.vi" "Inspection Point"() -> (w889:string)
        n644 = Equal?(x=w889, y="SubAssembly") -> (x = y?=w888:bool)
        n645 = case shown="False" w888 {
          tunnel: [w907 w1055] -> w904
          tunnel: [FALSE w1054] -> w903
          tunnel: w892 -> [w906 w1053]
          frame True {
            # "Quick"
            n646 = case shown="True" w906 {
              tunnel: [TRUE w928] -> w907
              frame False {
                n647 = local read "refnum out"() -> (w920:refnum<file>)
                n648 = call "dataSampled.vi"("refnum in"=w920) -> ("error out"=w914:errorcluster, "refnum out"=w919:refnum<file>)  [unwired: 9 in]
                n649 = call "dataSampled.vi"("Error In"=w914, "refnum in"=w919) -> ("error out"=w913:errorcluster, "refnum out"=w918:refnum<file>)  [unwired: 8 in]
                n650 = call "dataSampled.vi"("Error In"=w913, "refnum in"=w918) -> ("error out"=w912:errorcluster, "refnum out"=w917:refnum<file>)  [unwired: 8 in]
                n651 = call "dataSampled.vi"("Error In"=w912, "refnum in"=w917) -> ("error out"=w911:errorcluster, "refnum out"=w916:refnum<file>)  [unwired: 8 in]
                n652 = call "dataSampled.vi"("Error In"=w911, "refnum in"=w916) -> ("error out"=w910:errorcluster, "refnum out"=w915:refnum<file>)  [unwired: 8 in]
                n653 = call "dataSampled.vi"("Error In"=w910, "refnum in"=w915) -> ()  [unwired: 8 in, 2 out]
              }
              frame True {
                n654 = local write "INCLINE-14"("(W§c6RðS\nN\fÿ\tc\u000bN\u0000N*N\u001c ë_\u001f>Pe\u001d \tc®\fÿ6q\u000eTI{_Ó~gôv0R\u0007c:yopÝO\u0001c¹p®N\u00020\n\u0000(W§c6RðS\nN\fÿ\tc\u0000gNOv\u001c ë_\u001f>Pe\u001d \tc®\u00020\n\u0000\n\u0000O\u0000n\u0000 \u0000t\u0000h\u0000e\u0000 \u0000c\u0000o\u0000n\u0000s\u0000o\u0000l\u0000e\u0000,\u0000 \u0000p\u0000r\u0000e\u0000s\u0000s\u0000 \u0000n\u0000e\u0000x\u0000t\u0000 \u0000Q\u0000u\u0000i\u0000c\u0000k\u0000 \u0000i\u0000n\u0000c\u0000l\u0000i\u0000n\u0000e\u0000 \u0000b\u0000u\u0000t\u0000t\u0000o\u0000n\u0000 \u0000a\u0000n\u0000d\u0000 \u0000w\u0000a\u0000i\u0000t\u0000 \u0000f\u0000o\u0000r\u0000 \u0000r\u0000e\u0000s\u0000u\u0000l\u0000t\u0000s\u0000 \u0000t\u0000i\u0000l\u0000l\u0000 \u0000i\u0000n\u0000d\u0000i\u0000c\u0000a\u0000t\u0000o\u0000r\u0000 \u0000r\u0000e\u0000m\u0000a\u0000i\u0000n\u0000s\u0000 \u0000l\u0000i\u0000t\u0000.\u0000\n\u0000O\u0000n\u0000 \u0000t\u0000h\u0000e\u0000 \u0000c\u0000o\u0000n\u0000s\u0000o\u0000l\u0000e\u0000,\u0000 \u0000p\u0000r\u0000e\u0000s\u0000s\u0000 \u0000t\u0000h\u0000e\u0000 \u0000l\u0000o\u0000w\u0000e\u0000s\u0000t\u0000 \u0000Q\u0000u\u0000i\u0000c\u0000k\u0000 \u0000i\u0000n\u0000c\u0000l\u0000i\u0000n\u0000e\u0000 \u0000b\u0000u\u0000t\u0000t\u0000o\u0000n\u0000.\u0000\u0000\u0000o\u0000n\u0000.\u0000") -> ()
                n655 = local read "EQF1259 com port"() -> (w927:refnum<visa-resource-name>)
                n656 = call "parseQuickKey.vi"("VISA resource name"=w927, "write buffer"="®\b", "y"=2, "x"=0) -> ("KeyCodeName"=w923:string[])  [unwired: 11 in, 4 out]
                n657 = call-poly <userlib>:"Filter 1D Array__ogtk.vi"("items to filter"="", "array"=w923) -> ("filtered array"=w921:string[])  [unwired: 4 in, 1 out]
                n658 = flat-sequence {
                  tunnel: w921 -> [w930]
                  tunnel: [w1049] -> w928
                  frame #0 {
                    n659 = while {
                      shift-right: [w934] -> _
                      shift-left: 0 -> [w935]
                      tunnel: w930 -> [w933]
                      stop <- w932 stop-if-true
                      n660 = case shown="1" w935 {
                        tunnel: [1 _] -> w934
                        tunnel: [FALSE TRUE] -> w932
                        tunnel: w933 -> [w936 _]
                        frame 0, Default {
                          n661 = while {
                            shift-right: [w942] -> _
                            shift-left: 0 -> [w943]
                            tunnel: w936 -> [w940]
                            stop <- w941 stop-if-true
                            n662 = case shown="0, Default" w943 {
                              tunnel: [w948 w969 2] -> w942
                              tunnel: [FALSE FALSE TRUE] -> w941
                              tunnel: w940 -> [_ w967 _]
                              frame 0, Default {
                                n663 = for {
                                N: 2 -> [_]
                                tunnel: [w963] -> w962 mode=indexing
                                n664 = Random Number (0-1)() -> (number: 0 to 1=w966:dbl)
                                n665 = Multiply(x=w966, y=10.0) -> (x*y=w964:dbl)
                                n666 = To Word Integer(number=w964) -> (16bit integer=w963:i16)
                                }
                                n667 = Index Array(array=w962, index #1=0 ("index"), index #2=1 ("index")) -> (element #1=w960:i16, element #2=w961:i16)
                                n668 = Max & Min(x=w960, y=w961) -> (max(x,y)=w949:i16, min(x,y)=w950:i16)
                                n669 = local write "max(x,y)"(w949) -> ()
                                n670 = local write "min(x,y)"(w950) -> ()
                                n671 = Not Equal?(x=w949, y=w950) -> (x != y?=w955:bool)
                                n672 = Greater Or Equal?(x=i16 8 ("y"), y=w949) -> (x >= y?=w953:bool)
                                n673 = Greater Or Equal?(x=w950, y=i16 3) -> (x >= y?=w954:bool)
                                n674 = Compound Arithmetic op=AND(TRUE ("value"), w953, w955, w954) -> (w945:bool)
                                n675 = Select(t=1, s=w945, f=0) -> (s? t:f=w948:i32)
                              }
                              frame 1 {
                                n676 = for {
                                tunnel: w967 -> [w993] mode=indexing
                                tunnel: [w990] -> w980 mode=indexing
                                n677 = local read "max(x,y)"() -> (w989:i16)
                                n678 = Number To Decimal String(number=w989, width (-)=i16 0) -> (decimal integer string=w991:string)
                                n679 = Equal?(x=w993, y=w991) -> (x = y?=w990:bool)
                                }
                                n680 = for {
                                tunnel: w967 -> [w988] mode=indexing
                                tunnel: [w985] -> w977 mode=indexing
                                n681 = local read "min(x,y)"() -> (w984:i16)
                                n682 = Number To Decimal String(number=w984, width (-)=i16 0) -> (decimal integer string=w986:string)
                                n683 = Equal?(x=w988, y=w986) -> (x = y?=w985:bool)
                                }
                                n684 = call-poly <userlib>:"Filter 1D Array__ogtk.vi"("items to filter"=FALSE, "array"=w980) -> ("filtered array"=w979:bool[])  [unwired: 4 in, 1 out]
                                n685 = call-poly <userlib>:"Filter 1D Array__ogtk.vi"("items to filter"=FALSE, "array"=w977) -> ("filtered array"=w978:bool[])  [unwired: 4 in, 1 out]
                                n686 = Index Array(array=w979, index=0) -> (element=w981:bool)
                                n687 = Index Array(array=w978, index=0) -> (element=w982:bool)
                                n688 = Compound Arithmetic op=AND(TRUE ("value"), w981, w982) -> (w983:bool)
                                n689 = Select(t=2, s=w983, f=0) -> (s? t:f=w969:i32)
                              }
                              frame 2 {
                                n690 = local read "max(x,y)"() -> (w999:i16)
                                n691 = local read "min(x,y)"() -> (w998:i16)
                                n692 = Build Array(w999, w998, i16 0) -> (w997:i16[])
                                n693 = local write "appended array"(w997) -> ()
                              }
                            }
                          }
                        }
                        frame 1 {
                          n694 = local read "appended array"() -> (w1002:i16[])
                          n695 = for {
                            N: 3 -> [_]
                            tunnel: w1002 -> [w1005]
                            i -> [w1004]
                            n696 = while {
                              tunnel: w1005 -> [w1022]
                              tunnel: w1004 -> [w1020]
                              tunnel: [w1017] -> w1003
                              i -> [w1019]
                              stop <- w1017 stop-if-true
                              n697 = Index Array(array=w1022, index=w1020) -> (element=w1021:i16)
                              n698 = To Double Precision Float(number=w1021) -> (double precision float=w1016:dbl)
                              n699 = local write "Press Next"(w1016) -> ()
                              n700 = Equal?(x=w1019, y=1) -> (x = y?=w1017:bool)
                            }
                            n701 = case shown="True" w1003 {
                              frame False {
                              }
                              frame True {
                                n702 = while {
                                stop <- w1011 stop-if-true
                                w1015 = 0.3
                                n703 = local read "EQF1259 com port"() -> (w1008:refnum<visa-resource-name>)
                                n704 = local read "Press Next"() -> (w1010:dbl)
                                n705 = Add(x=w1010, y=w1015) -> (x+y=w1014:dbl)
                                n706 = Subtract(x=w1010, y=w1015) -> (x-y=w1013:dbl)
                                n707 = call "inclineAquire.vi"("Negative Incline"=0.0, "VISA Refnum in"=w1008) -> ("Incline Out"=w1009:dbl)  [unwired: 8 in, 1 out]
                                n708 = local write "incline"(w1009) -> ()
                                n709 = local read "stopI"() -> (w1012:bool)
                                n710 = In Range and Coerce(upper limit=w1014, x=w1009, lower limit=w1013) -> (In Range?=w1006:bool)  [unwired: 1 out]
                                n711 = Or(x=w1006, y=w1012) -> (x .or. y?=w1011:bool)
                                n712 = local write "Quickincline"(w1006) -> ()
                                }
                              }
                            }
                          }
                        }
                      }
                      n713 = local write "ZERO"(w932) -> ()
                    }
                  }
                  frame #1 {
                    n714 = for {
                      N: 2 -> [_]
                      tunnel: [w1047] -> w1030
                      tunnel: [w1046] -> w1027
                      n715 = local read "refnum out"() -> (w1048:refnum<file>)
                      n716 = call "dataSampled.vi"("refnum in"=w1048) -> ("error out"=w1047:errorcluster, "refnum out"=w1046:refnum<file>)  [unwired: 9 in]
                    }
                    n717 = case shown="True" TRUE {
                      tunnel: w1030 -> [w1040 w1044]
                      tunnel: [w1039 w1043] -> w1029
                      tunnel: [w1038 w1042] -> w1026
                      tunnel: w1027 -> [w1037 w1041]
                      frame False {
                        n718 = call "dataSampled.vi"("Error In"=w1040, "refnum in"=w1037) -> ("error out"=w1039:errorcluster, "refnum out"=w1038:refnum<file>)  [unwired: 8 in]
                      }
                      frame True {
                        n719 = local read "Quickincline"() -> (w1045:bool)
                        n720 = call "Pass_Fail.vi"("error in (no error)"=w1044, "OK"=w1045, "Byte Stream File in"=w1041) -> ("error out"=w1043:errorcluster, "Byte Stream File out"=w1042:refnum<file>)  [unwired: 7 in]
                      }
                    }
                    n721 = for {
                      N: 2 -> [_]
                      tunnel: [w1036] -> w1023
                      tunnel: w1029 -> [w1035]
                      tunnel: w1026 -> [w1034]
                      tunnel: [w1033] -> w1025
                      n722 = call "dataSampled.vi"("Error In"=w1035, "refnum in"=w1034) -> ("error out"=w1036:errorcluster, "refnum out"=w1033:refnum<file>)  [unwired: 8 in]
                    }
                    n723 = local read "ZERO"() -> (w1024:bool)
                    n724 = call "Pass_Fail.vi"("error in (no error)"=w1023, "OK"=w1024, "Byte Stream File in"=w1025) -> ()  [unwired: 7 in, 2 out]
                  }
                  frame #2 {
                    n725 = local read "Quickincline"() -> (w1051:bool)
                    n726 = local read "ZERO"() -> (w1050:bool)
                    n727 = Compound Arithmetic op=AND(TRUE, w1051, w1050) -> (w1049:bool)
                    n728 = local write "INCLINE PASS"(w1049) -> ()
                  }
                }
              }
            }
          }
          frame False {
            # "Standard"
            n729 = case shown="True" w1053 {
              tunnel: [TRUE w1083] -> w1055
              tunnel: [FALSE ("E-Stop/Incline") FALSE ("E-Stop/Incline")] -> w1054
              frame False {
                n730 = local read "refnum out"() -> (w1067:refnum<file>)
                n731 = call "dataSampled.vi"("refnum in"=w1067) -> ("error out"=w1063:errorcluster, "refnum out"=w1066:refnum<file>)  [unwired: 9 in]
                n732 = call "dataSampled.vi"("Error In"=w1063, "refnum in"=w1066) -> ("error out"=w1062:errorcluster, "refnum out"=w1065:refnum<file>)  [unwired: 8 in]
                n733 = call "dataSampled.vi"("Error In"=w1062, "refnum in"=w1065) -> ("error out"=w1061:errorcluster, "refnum out"=w1056:refnum<file>)  [unwired: 8 in]
                n734 = call "dataSampled.vi"("Error In"=w1061, "refnum in"=w1056) -> ("error out"=w1060:errorcluster, "refnum out"=w1057:refnum<file>)  [unwired: 8 in]
                n735 = call "dataSampled.vi"("Error In"=w1060, "refnum in"=w1057) -> ("error out"=w1059:errorcluster, "refnum out"=w1058:refnum<file>)  [unwired: 8 in]
                n736 = call "dataSampled.vi"("Error In"=w1059, "refnum in"=w1058) -> ()  [unwired: 8 in, 2 out]
              }
              frame True {
                n737 = flat-sequence {
                  tunnel: [w1091] -> w1072
                  tunnel: [w1087] -> w1071
                  tunnel: [w1090] -> w1070
                  tunnel: [w1089] -> w1069
                  tunnel: [w1093] -> w1081
                  tunnel: [w1103] -> w1076
                  tunnel: w1072 -> [w1096]
                  tunnel: w1071 -> [w1093]
                  tunnel: w1070 -> [w1095]
                  tunnel: w1069 -> [w1094]
                  tunnel: [w1118] -> w1086
                  tunnel: [w1119] -> w1085
                  tunnel: [w1117] -> w1082
                  tunnel: w1081 -> [w1116]
                  tunnel: w1076 -> [w1114]
                  tunnel: [w1111] -> w1075
                  tunnel: [w1110] -> w1074
                  tunnel: w1086 -> [w1136]
                  tunnel: w1085 -> [w1138]
                  tunnel: w1082 -> [w1137]
                  tunnel: [w1122] -> w1080
                  tunnel: w1075 -> [w1135]
                  tunnel: w1074 -> [w1132]
                  tunnel: w1080 -> [w1234]
                  tunnel: [w1234] -> w1079
                  tunnel: w1079 -> [w1249]
                  tunnel: [w1249] -> w1078
                  tunnel: w1078 -> [w1274]
                  tunnel: [w1274] -> w1077
                  tunnel: w1077 -> [w1299]
                  tunnel: [w1299] -> w1073
                  tunnel: [w1316] -> w1083
                  tunnel: w1073 -> [w1315]
                  frame #0 {
                    w1091 = FALSE ("sdFeature")
                    n738 = Wait (ms)(milliseconds to wait=u32 250) -> ()  [unwired: 1 out]
                    n739 = local read "EQF1259 com port"() -> (w1089:refnum<visa-resource-name>)
                    n740 = call "usbUart.vi"("VISA resource name"=w1089, "write buffer"="€\u0002", "sdFeature"=w1091) -> ("double precision float"=w1087:dbl, "error out"=w1090:errorcluster)  [unwired: 1 in, 14 out]
                  }
                  frame #1 {
                    n741 = Wait (ms)(milliseconds to wait=u32 250) -> ()  [unwired: 1 out]
                    n742 = call "usbUart.vi"("VISA resource name"=w1094, "write buffer"="‚\u0002", "sdFeature"=w1096, "error in (no error)"=w1095) -> ("number[0]"=w1098:u32, "negative incline"=w1097:dbl, "error out"=w1103:errorcluster)  [unwired: 13 out]
                    n743 = Equal?(x=w1098, y=u32 0) -> (x = y?=w1099:bool)
                    n744 = case shown="False" w1099 {
                      tunnel: w1098 -> [_ w1106]
                      tunnel: w1097 -> [w1104 _]
                      frame False {
                        "negative incline" <- w1104
                      }
                      frame True {
                        n745 = To Double Precision Float(number=w1106) -> (double precision float=w1105:dbl)
                        n746 = local write "negative incline"(w1105) -> ()
                      }
                    }
                  }
                  frame #2 {
                    n747 = Wait (ms)(milliseconds to wait=u32 250) -> ()  [unwired: 1 out]
                    n748 = local read "EQF1259 com port"() -> (w1113:refnum<visa-resource-name>)
                    n749 = local read "negative incline"() -> (w1108:dbl)
                    n750 = local write "Press Next"(w1108) -> ()
                    n751 = call "usbUart.vi"("VISA resource name"=w1113, "write buffer"="Å\u0002", "sdFeature"=FALSE, "error in (no error)"=w1114) -> ("double precision float"=w1111:dbl, "error out"=w1115:errorcluster)  [unwired: 14 out]
                    n752 = call "inclineCount.vi"("error in (no error)"=w1115, "negative incline"=w1108, "max incline"=w1116) -> ("error out"=w1110:errorcluster, "press start"=w1118:dbl, "max incline"=w1117:dbl)  [unwired: 5 in, 1 out]
                    n753 = Not Equal?(x=w1108, y=0.0) -> (x != y?=w1119:bool)
                  }
                  frame #3 {
                    # "Note: changed incline compare from .6 to .1 on negative and from .5 to .1 on positive to eliminate false presses at the low end. need more data. 06-04-20"
                    n754 = local read "EQF1259 com port"() -> (w1139:refnum<visa-resource-name>)
                    n755 = Increment(x=w1137) -> (x+1=w1126:dbl)
                    n756 = Decrement(x=w1136) -> (x-1=w1125:dbl)
                    n757 = call "parseQuickKey.vi"("VISA resource name"=w1139, "write buffer"="®\b", "y"=2, "x"=0, "error in (no error)"=w1132) -> ("lengthString"=w1127:i32, "KeyCodeName"=w1140:string[], "No Keys"=w1122:bool, "error out"=w1133:errorcluster)  [unwired: 10 in, 1 out]
                    n758 = property on="incline" class="WFChart (strict)"("YScale.Maximum"=w1126) -> ()  [unwired: 2 in, 2 out]
                    n759 = property on="incline" class="WFChart (strict)"("YScale.Minimum"=w1125) -> ()  [unwired: 2 in, 2 out]
                    n760 = Decrement(x=w1127) -> (x-1=w1131:i32)
                    n761 = call "delayTransmax.vi"("error in (no error)"=w1133, "Tmax"=w1135, "Bcount"=w1131) -> ("error out"=w1123:errorcluster, "Tdelay"=w1134:dbl)  [unwired: 7 in]
                    n762 = case shown="True" w1138 {
                      tunnel: w1131 -> [w1144 w1187]
                      tunnel: w1139 -> [w1146 w1189]
                      tunnel: w1140 -> [w1145 w1188]
                      tunnel: w1134 -> [w1143 w1186]
                      tunnel: w1122 -> [w1141 w1184]
                      frame False {
                        n763 = for {
                          N: w1144 -> [_]
                          tunnel: w1146 -> [w1159]
                          tunnel: w1145 -> [w1157]
                          tunnel: w1143 -> [w1148]
                          tunnel: [w1149] -> w1142 mode=indexing
                          tunnel: w1141 -> [w1147]
                          i -> [w1158]
                          n764 = Index Array(array=w1157, index=w1158) -> (element=w1151:string)
                          n765 = Empty String/Path?(string/path=w1151) -> (empty?=w1153:bool)
                          n766 = Equal?(x=w1151, y="0") -> (x = y?=w1152:bool)
                          n767 = Or(x=w1152, y=w1153) -> (x .or. y?=w1154:bool)
                          n768 = Not(x=w1154) -> (.not. x?=w1156:bool)
                          n769 = case shown="True" w1156 {
                            tunnel: [w1162 TRUE] -> w1150
                            tunnel: w1151 -> [_ w1170]
                            tunnel: w1148 -> [_ w1166]
                            frame False {
                              n770 = local read "Press Next"() -> (w1161:dbl)
                              n771 = local read "MAX"() -> (w1160:dbl)
                              n772 = Equal?(x=w1161, y=w1160) -> (x = y?=w1165:bool)
                              n773 = Select(t=TRUE, s=w1165, f=FALSE) -> (s? t:f=w1162:bool)
                            }
                            frame True {
                              n774 = To Unsigned Long Integer(number=w1166) -> (unsigned 32bit integer=w1167:u32)
                              n775 = Fract/Exp String To Number(string=w1170) -> (number=w1169:dbl)  [unwired: 3 in, 1 out]
                              n776 = Wait (ms)(milliseconds to wait=w1167) -> ()  [unwired: 1 out]
                              n777 = local write "Press Next"(w1169) -> ()
                            }
                          }
                          n778 = case shown="True" w1150 {
                            tunnel: w1159 -> [_ w1173]
                            tunnel: [_ w1172] -> w1149
                            tunnel: w1147 -> [w1171 _]
                            frame False {
                              n779 = local write "Quickincline"(w1171) -> ()
                            }
                            frame True {
                              n780 = while {
                                tunnel: w1173 -> [w1182]
                                tunnel: [w1177] -> w1172
                                stop <- w1176 stop-if-true
                                w1179 = 0.5 ("y")
                                n781 = local read "negative incline"() -> (w1183:dbl)
                                n782 = local read "Press Next"() -> (w1178:dbl)
                                n783 = Add(x=w1178, y=w1179) -> (x+y=w1180:dbl)
                                n784 = Subtract(x=w1178, y=w1179) -> (x-y=w1181:dbl)
                                n785 = call "inclineAquire.vi"("Negative Incline"=w1183, "VISA Refnum in"=w1182) -> ("Incline Out"=w1177:dbl)  [unwired: 8 in, 1 out]
                                n786 = local write "incline"(w1177) -> ()
                                n787 = In Range and Coerce(upper limit=w1180, x=w1177, lower limit=w1181) -> (In Range?=w1174:bool)  [unwired: 1 out]
                                n788 = Or(x=w1174, y="stopI") -> (x .or. y?=w1176:bool)
                                n789 = local write "Quickincline"(w1174) -> ()
                              }
                            }
                          }
                        }
                        n790 = local write "inclineArray"(w1142) -> ()
                      }
                      frame True {
                        n791 = for {
                          N: w1187 -> [_]
                          tunnel: w1189 -> [_]
                          tunnel: w1188 -> [w1200]
                          tunnel: w1186 -> [w1191]
                          tunnel: [w1199] -> w1185 mode=indexing
                          tunnel: w1184 -> [w1190]
                          i -> [w1201]
                          n792 = Index Array(array=w1200, index=w1201) -> (element=w1195:string)
                          n793 = Empty String/Path?(string/path=w1195) -> (empty?=w1197:bool)
                          n794 = Equal?(x=w1195, y="0") -> (x = y?=w1196:bool)
                          n795 = Or(x=w1196, y=w1197) -> (x .or. y?=w1198:bool)
                          n796 = Not(x=w1198) -> (.not. x?=w1192:bool)
                          n797 = case shown="True" w1192 {
                            tunnel: w1195 -> [_ w1212]
                            tunnel: [w1202 TRUE] -> w1193
                            tunnel: w1191 -> [_ w1208]
                            frame False {
                              n798 = local read "Press Next"() -> (w1207:dbl)
                              n799 = local read "MAX"() -> (w1206:dbl)
                              n800 = Equal?(x=w1207, y=w1206) -> (x = y?=w1205:bool)
                              n801 = Select(t=TRUE, s=w1205, f=FALSE) -> (s? t:f=w1202:bool)
                            }
                            frame True {
                              n802 = To Unsigned Long Integer(number=w1208) -> (unsigned 32bit integer=w1209:u32)
                              n803 = Fract/Exp String To Number(string=w1212) -> (number=→"Press Next":dbl)  [unwired: 3 in, 1 out]
                              n804 = Wait (ms)(milliseconds to wait=w1209) -> ()  [unwired: 1 out]
                            }
                          }
                          n805 = case shown="True" w1193 {
                            tunnel: [_ w1214] -> w1199
                            tunnel: w1190 -> [w1213 _]
                            frame False {
                              n806 = local write "Quickincline"(w1213) -> ()
                            }
                            frame True {
                              n807 = while {
                                tunnel: [w1215] -> w1214
                                stop <- w1220 stop-if-true
                                n808 = local read "EQF1259 com port"() -> (w1221:refnum<visa-resource-name>)
                                n809 = local read "negative incline"() -> (w1223:dbl)
                                n810 = call "inclineAquire.vi"("Negative Incline"=w1223, "VISA Refnum in"=w1221) -> ("Incline Out"=w1215:dbl)  [unwired: 8 in, 1 out]
                                "incline" <- w1215
                                n811 = local read "Press Next"() -> (w1222:dbl)
                                n812 = Greater Or Equal?(x=w1215, y=0.0) -> (x >= y?=w1225:bool)
                                n813 = case shown="False" w1225 {
                                tunnel: w1222 -> [w1228 w1233]
                                tunnel: [w1227 w1231] -> w1217
                                tunnel: [w1226 w1230] -> w1216
                                frame False {
                                w1229 = 0.5 ("x")
                                # "Positive"
                                n814 = Subtract(x=w1228, y=w1229) -> (x-y=w1227:dbl)
                                n815 = Add(x=w1229, y=w1228) -> (x+y=w1226:dbl)
                                }
                                frame True {
                                w1232 = 0.6
                                # "negative"
                                n816 = Subtract(x=w1233, y=w1232) -> (x-y=w1231:dbl)
                                n817 = Add(x=w1232, y=w1233) -> (x+y=w1230:dbl)
                                }
                                }
                                n818 = local read "stopI"() -> (w1219:bool)
                                n819 = In Range and Coerce(upper limit=w1216, x=w1215, lower limit=w1217) -> (In Range?=w1218:bool)  [unwired: 1 out]
                                "Quickincline" <- w1218
                                n820 = Or(x=w1218, y=w1219) -> (x .or. y?=w1220:bool)
                              }
                            }
                          }
                        }
                        "inclineArray" <- w1185
                      }
                    }
                    n821 = call "inclinePIP.vi"("error in (no error)"=w1123, "QUICK_KEYS"=w1122, "INCLINE"=TRUE) -> ("INCLINE-14"=→"INCLINE-14":string)  [unwired: 7 in, 1 out]
                    "MAX" <- w1137
                    "MIN" <- w1136
                  }
                  frame #4 {
                    n822 = local read "MIN"() -> (w1242:dbl)
                    n823 = Number To Fractional String(number=w1242) -> (F-format string=w1241:string)  [unwired: 3 in]
                    n824 = local read "refnum out"() -> (w1239:refnum<file>)
                    n825 = local read "MAX"() -> (w1243:dbl)
                    n826 = call "dataSampled.vi"("Data"=w1241, "refnum in"=w1239) -> ("error out"=w1237:errorcluster, "refnum out"=w1238:refnum<file>)  [unwired: 8 in]
                    n827 = Number To Fractional String(number=w1243) -> (F-format string=w1240:string)  [unwired: 3 in]
                    n828 = call "dataSampled.vi"("Error In"=w1237, "Data"=w1240, "refnum in"=w1238) -> ("error out"=w1235:errorcluster, "refnum out"=w1236:refnum<file>)  [unwired: 7 in]
                    n829 = case shown="False" w1234 {
                      tunnel: w1236 -> [w1245 w1248]
                      tunnel: w1235 -> [w1244 w1247]
                      frame False {
                        n830 = local read "Quickincline"() -> (w1246:bool)
                        n831 = call "Pass_Fail.vi"("error in (no error)"=w1244, "OK"=w1246, "Byte Stream File in"=w1245) -> ()  [unwired: 7 in, 2 out]
                      }
                      frame True {
                        n832 = call "dataSampled.vi"("Error In"=w1247, "refnum in"=w1248) -> ()  [unwired: 8 in, 2 out]
                      }
                    }
                  }
                  frame #5 {
                    n833 = case shown="True" w1249 {
                      tunnel: [w1252 w1264] -> w1250
                      frame False {
                        n834 = while {
                          tunnel: [w1255] -> w1252
                          stop <- w1254 stop-if-true
                          n835 = local read "EQF1259 com port"() -> (w1263:refnum<visa-resource-name>)
                          n836 = local read "negative incline"() -> (w1262:dbl)
                          n837 = local read "MAX"() -> (w1261:dbl)
                          n838 = call "inclineAquire.vi"("Negative Incline"=w1262, "VISA Refnum in"=w1263) -> ("Incline Out"=w1258:dbl)  [unwired: 8 in, 1 out]
                          n839 = Subtract(x=w1261, y=2.0) -> (x-y=w1259:dbl)
                          n840 = local write "incline"(w1258) -> ()
                          n841 = local read "stopI"() -> (w1256:bool)
                          n842 = Equal?(x=w1258, y=w1259) -> (x = y?=w1253:bool)
                          n843 = Or(x=w1256, y=w1253) -> (x .or. y?=w1254:bool)
                          n844 = Not(x=w1256) -> (.not. x?=w1257:bool)
                          n845 = And(x=w1253, y=w1257) -> (x .and. y?=w1255:bool)
                        }
                        "Down" <- w1252
                      }
                      frame True {
                        n846 = while {
                          tunnel: [w1270] -> w1264
                          stop <- w1268 stop-if-true
                          n847 = local read "EQF1259 com port"() -> (w1273:refnum<visa-resource-name>)
                          n848 = local read "negative incline"() -> (w1272:dbl)
                          n849 = call "inclineAquire.vi"("Negative Incline"=w1272, "VISA Refnum in"=w1273) -> ("Incline Out"=w1265:dbl)  [unwired: 8 in, 1 out]
                          n850 = local write "incline"(w1265) -> ()
                          n851 = local read "stopI"() -> (w1267:bool)
                          n852 = Equal?(x=w1265, y=2.0) -> (x = y?=w1266:bool)
                          n853 = Or(x=w1266, y=w1267) -> (x .or. y?=w1268:bool)
                          n854 = Not(x=w1267) -> (.not. x?=w1269:bool)
                          n855 = And(x=w1266, y=w1269) -> (x .and. y?=w1270:bool)
                        }
                        n856 = local write "Up"(w1264) -> ()
                      }
                    }
                    n857 = local read "refnum out"() -> (w1251:refnum<file>)
                    n858 = call "Pass_Fail.vi"("OK"=w1250, "Byte Stream File in"=w1251) -> ()  [unwired: 8 in, 2 out]
                  }
                  frame #6 {
                    n859 = case shown="True" w1274 {
                      tunnel: [w1277 w1289] -> w1275
                      frame False {
                        n860 = while {
                          tunnel: [w1281] -> w1277
                          stop <- w1282 stop-if-true
                          n861 = local read "EQF1259 com port"() -> (w1288:refnum<visa-resource-name>)
                          n862 = local read "negative incline"() -> (w1287:dbl)
                          n863 = local read "MAX"() -> (w1286:dbl)
                          n864 = call "inclineAquire.vi"("Negative Incline"=w1287, "VISA Refnum in"=w1288) -> ("Incline Out"=w1283:dbl)  [unwired: 8 in, 1 out]
                          n865 = Subtract(x=w1286, y=1.0) -> (x-y=w1284:dbl)
                          n866 = local write "incline"(w1283) -> ()
                          n867 = local read "stopI"() -> (w1279:bool)
                          n868 = Equal?(x=w1283, y=w1284) -> (x = y?=w1278:bool)
                          n869 = Or(x=w1279, y=w1278) -> (x .or. y?=w1282:bool)
                          n870 = Not(x=w1279) -> (.not. x?=w1280:bool)
                          n871 = And(x=w1278, y=w1280) -> (x .and. y?=w1281:bool)
                        }
                        "Up" <- w1277
                      }
                      frame True {
                        n872 = while {
                          tunnel: [w1295] -> w1289
                          stop <- w1292 stop-if-true
                          n873 = local read "EQF1259 com port"() -> (w1298:refnum<visa-resource-name>)
                          n874 = local read "negative incline"() -> (w1297:dbl)
                          n875 = call "inclineAquire.vi"("Negative Incline"=w1297, "VISA Refnum in"=w1298) -> ("Incline Out"=w1290:dbl)  [unwired: 8 in, 1 out]
                          n876 = local write "incline"(w1290) -> ()
                          n877 = local read "stopI"() -> (w1293:bool)
                          n878 = Equal?(x=w1290, y=1.0) -> (x = y?=w1291:bool)
                          n879 = Or(x=w1293, y=w1291) -> (x .or. y?=w1292:bool)
                          n880 = Not(x=w1293) -> (.not. x?=w1294:bool)
                          n881 = And(x=w1291, y=w1294) -> (x .and. y?=w1295:bool)
                        }
                        n882 = local write "Down"(w1289) -> ()
                      }
                    }
                    n883 = local read "refnum out"() -> (w1276:refnum<file>)
                    n884 = call "Pass_Fail.vi"("OK"=w1275, "Byte Stream File in"=w1276) -> ()  [unwired: 8 in, 2 out]
                  }
                  frame #7 {
                    n885 = case shown="False" w1299 {
                      tunnel: [w1301 TRUE] -> w1300
                      frame False {
                        n886 = while {
                          tunnel: [w1309] -> w1301
                          stop <- w1308 stop-if-true
                          n887 = local read "EQF1259 com port"() -> (w1312:refnum<visa-resource-name>)
                          n888 = local read "negative incline"() -> (w1311:dbl)
                          n889 = call "inclineAquire.vi"("Negative Incline"=w1311, "VISA Refnum in"=w1312) -> ("Incline Out"=w1304:dbl)  [unwired: 8 in, 1 out]
                          n890 = local write "incline"(w1304) -> ()
                          n891 = In Range and Coerce(upper limit=1.0, x=w1304, lower limit=-0.1 ("y")) -> (In Range?=w1305:bool)  [unwired: 1 out]
                          n892 = local read "stopI"() -> (w1306:bool)
                          n893 = Or(x=w1306, y=w1305) -> (x .or. y?=w1308:bool)
                          n894 = Not(x=w1306) -> (.not. x?=w1307:bool)
                          n895 = And(x=w1305, y=w1307) -> (x .and. y?=w1309:bool)
                        }
                        n896 = local read "refnum out"() -> (w1302:refnum<file>)
                        n897 = call "Pass_Fail.vi"("OK"=w1301, "Byte Stream File in"=w1302) -> ()  [unwired: 8 in, 2 out]
                      }
                      frame True {
                        n898 = local read "refnum out"() -> (w1313:refnum<file>)
                        n899 = call "dataSampled.vi"("refnum in"=w1313) -> ()  [unwired: 9 in, 2 out]
                      }
                    }
                    "ZERO" <- w1300
                  }
                  frame #8 {
                    n900 = case shown="True" w1315 {
                      tunnel: [w1317 w1323] -> w1316
                      frame False {
                        n901 = local read "Quickincline"() -> (w1322:bool)
                        n902 = local read "Down"() -> (w1321:bool)
                        n903 = local read "ZERO"() -> (w1319:bool)
                        n904 = local read "Up"() -> (w1320:bool)
                        n905 = Compound Arithmetic op=AND(TRUE ("value"), w1319, w1320, w1321, w1322) -> (w1317:bool)
                      }
                      frame True {
                        n906 = local read "Down"() -> (w1324:bool)
                        n907 = local read "Up"() -> (w1325:bool)
                        n908 = Compound Arithmetic op=AND(TRUE, w1325, w1324) -> (w1323:bool)
                      }
                    }
                    "INCLINE PASS" <- w1316
                  }
                }
              }
            }
          }
        }
        n909 = Select(t=T3."CSafe" ("Tab Control"), s=w904, f=T3."Failed" ("Tab Control")) -> (s? t:f=w905:T3)
      }
      frame "Resistance" {
        w1340 = ""
        w1338 = FALSE
        # "#define RESISTNACE_PROTOCOL         0xA1\n//    #define TAG_RESISTANCE_DRIVER_NONE  1\n//    #define TAG_RESISTANCE_DRIVER_ADC   2\n//    #define TAG_RESISTANCE_DRIVER_RS485 3"
        # "protocolResistance"
        n910 = local write "resistanceArray"(dbl[] [0.0] ("resistanceArray")) -> ()
        n911 = local write "Least"(w1338) -> ()
        n912 = property on="resLower" class="DigNum (strict)"("Visible"=w1338) -> ()  [unwired: 2 in, 2 out]
        n913 = local write "stopR"(w1338) -> ()
        n914 = property on="resUpper" class="DigNum (strict)"("Visible"=w1338) -> ()  [unwired: 2 in, 2 out]
        n915 = property on="RESISTANCE/CURRENT" class="WFChart (strict)"("History Data"=cluster{dbl, dbl}[] []) -> ()  [unwired: 2 in, 2 out]
        n916 = local write "IRun"(w1340) -> ()
        n917 = local write "IPeak"(w1340) -> ()
        n918 = local write "Decrease"(w1338) -> ()
        n919 = local write "QuickResistance"(w1338) -> ()
        n920 = local write "RESISTANCE PASS"(w1338) -> ()
        n921 = local write "overCurrent"(w1338) -> ()
        n922 = local write "Increase"(w1338) -> ()
        n923 = global write "Global_usbComm.vi" "runCurrent"(w1340) -> ()
        n924 = global read "Global_usbComm.vi" "maxCurrent"() -> (→"currentMaxResistance":string)
        n925 = global read "Global_usbComm.vi" "resistanceType"() -> (w1333:string)
        n926 = global read "Global_usbComm.vi" "RESISTANCE"() -> (w1334:string)
        n927 = Decimal String To Number(string=w1333) -> (number=w1336:i32)  [unwired: 2 in, 1 out]
        n928 = Equal?(x=w1334, y="1") -> (x = y?=w1337:bool)
        n929 = case shown="True" w1337 {
          selector: w1337 -> [_ w1360]
          tunnel: [TRUE w1369] -> w1344
          tunnel: w1336 -> [_ w1368]
          frame False {
            n930 = local read "refnum out"() -> (w1359:refnum<file>)
            n931 = call "dataSampled.vi"("refnum in"=w1359) -> ("error out"=w1352:errorcluster, "refnum out"=w1358:refnum<file>)  [unwired: 9 in]
            n932 = call "dataSampled.vi"("Error In"=w1352, "refnum in"=w1358) -> ("error out"=w1351:errorcluster, "refnum out"=w1357:refnum<file>)  [unwired: 8 in]
            n933 = call "dataSampled.vi"("Error In"=w1351, "refnum in"=w1357) -> ("error out"=w1350:errorcluster, "refnum out"=w1355:refnum<file>)  [unwired: 8 in]
            n934 = call "dataSampled.vi"("Error In"=w1350, "refnum in"=w1355) -> ("error out"=w1349:errorcluster, "refnum out"=w1354:refnum<file>)  [unwired: 8 in]
            n935 = call "dataSampled.vi"("Error In"=w1349, "refnum in"=w1354) -> ("error out"=w1348:errorcluster, "refnum out"=w1353:refnum<file>)  [unwired: 8 in]
            n936 = call "dataSampled.vi"("Error In"=w1348, "refnum in"=w1353) -> ()  [unwired: 8 in, 2 out]
          }
          frame True {
            # "have resistance?"
            n937 = local read "EQF1259 com port"() -> (w1366:refnum<visa-resource-name>)
            n938 = local read "refnum out"() -> (w1364:refnum<file>)
            n939 = call "resistanceScan.vi"("VISA Refnum in"=w1366) -> ("error out"=w1367:errorcluster, "Istring#"=w1365:string)  [unwired: 6 in, 3 out]
            n940 = global write "Global_usbComm.vi" "runCurrent"(w1365) -> ()
            n941 = global read "Global_usbComm.vi" "Inspection Point"() -> (w1362:string)
            n942 = call "dataSampled.vi"("Data"=w1365, "refnum in"=w1364) -> ()  [unwired: 8 in, 2 out]
            n943 = Equal?(x=w1362, y="SubAssembly") -> (x = y?=w1361:bool)
            n944 = case shown="False" w1361 {
              tunnel: [w1370 w1743] -> w1369
              tunnel: w1368 -> [w1371 w1742]
              tunnel: w1367 -> [_ w1737]
              tunnel: w1366 -> [_ w1740]
              tunnel: w1360 -> [_ w1741]
              frame True {
                # "quick"
                n945 = case shown="3" w1371 {
                  tunnel: [TRUE w1375 w1557] -> w1370
                  frame 1, Default {
                  }
                  frame 2 {
                    n946 = local read "EQF1259 com port"() -> (w1379:refnum<visa-resource-name>)
                    n947 = call "resistanceCalculator.vi"("VISA Refnum in"=w1379) -> ("steps/button Array"=w1377:dbl[][], "cycle"=w1376:dbl, "No Keys"=w1374:bool)  [unwired: 6 in, 6 out]
                    n948 = for {
                      N: w1376 -> [_]
                      tunnel: w1377 -> [w1554]
                      tunnel: [w1553] -> w1378 mode=indexing
                      i -> [w1551]
                      n949 = Index Array(array=w1554, index (row)=w1551, index (col)=0) -> (element=w1553:dbl)
                    }
                    n950 = Not(x=w1374) -> (.not. x?=w1373:bool)
                    n951 = case shown="False" w1373 {
                      tunnel: w1378 -> [_ w1425]
                      tunnel: w1377 -> [_ w1424]
                      tunnel: w1376 -> [_ w1423]
                      tunnel: [TRUE w1422] -> w1375
                      frame False {
                        n952 = flat-sequence {
                          frame #0 {
                            n953 = for {
                              N: 2 -> [_]
                              n954 = local read "refnum out"() -> (w1382:refnum<file>)
                              n955 = call "dataSampled.vi"("refnum in"=w1382) -> ()  [unwired: 9 in, 2 out]
                            }
                          }
                          frame #1 {
                            n956 = while {
                              shift-right: [w1396] -> _
                              shift-left: _ -> [w1395]
                              tunnel: [w1387] -> w1384
                              stop <- w1392 stop-if-true
                              n957 = local read "currentMaxResistance"() -> (w1399:string)
                              n958 = local read "EQF1259 com port"() -> (w1386:refnum<visa-resource-name>)
                              n959 = call "resistanceScan.vi"("Imax"=w1399, "VISA Refnum in"=w1386) -> ("error out"=w1398:errorcluster, "RESISTANCE/CURRENT"=w1385:cluster{dbl, dbl}, "ADC value"=w1389:dbl, "Istring#"=w1394:string)  [unwired: 5 in, 1 out]
                              n960 = local read "overCurrent"() -> (w1390:bool)
                              n961 = local write "IRun"(w1394) -> ()
                              n962 = local read "stopR"() -> (w1391:bool)
                              n963 = call "currentPeak.vi"("error in (no error)"=w1398, "Istring# change"=w1395, "Istring# scan"=w1394) -> ("Ipeak"=w1397:string, "Irun"=w1396:string)  [unwired: 6 in, 1 out]
                              n964 = local write "RESISTANCE/CURRENT"(w1385) -> ()
                              n965 = Equal?(x=w1389, y=1000.0) -> (x = y?=w1388:bool)
                              n966 = local write "IPeak"(w1397) -> ()
                              n967 = Compound Arithmetic op=OR(w1388, w1391, w1390) -> (w1392:bool)
                              n968 = Not(x=w1391) -> (.not. x?=w1400:bool)
                              n969 = Not(x=w1390) -> (.not. x?=w1401:bool)
                              n970 = Compound Arithmetic op=AND(w1388, w1401, w1400) -> (w1387:bool)
                            }
                            n971 = local read "refnum out"() -> (w1383:refnum<file>)
                            n972 = local write "Increase"(w1384) -> ()
                            n973 = call "Pass_Fail.vi"("OK"=w1384, "Byte Stream File in"=w1383) -> ()  [unwired: 8 in, 2 out]
                          }
                          frame #2 {
                            n974 = while {
                              shift-right: [w1415] -> _
                              shift-left: _ -> [w1414]
                              tunnel: [w1406] -> w1402
                              stop <- w1411 stop-if-true
                              n975 = local read "currentMaxResistance"() -> (w1418:string)
                              n976 = local read "EQF1259 com port"() -> (w1405:refnum<visa-resource-name>)
                              n977 = call "resistanceScan.vi"("Imax"=w1418, "VISA Refnum in"=w1405) -> ("error out"=w1417:errorcluster, "RESISTANCE/CURRENT"=w1404:cluster{dbl, dbl}, "ADC value"=w1408:dbl, "Istring#"=w1413:string)  [unwired: 5 in, 1 out]
                              n978 = local read "overCurrent"() -> (w1409:bool)
                              n979 = local write "IRun"(w1413) -> ()
                              n980 = local read "stopR"() -> (w1410:bool)
                              n981 = local write "RESISTANCE/CURRENT"(w1404) -> ()
                              n982 = call "currentPeak.vi"("error in (no error)"=w1417, "Istring# change"=w1414, "Istring# scan"=w1413) -> ("Ipeak"=w1416:string, "Irun"=w1415:string)  [unwired: 6 in, 1 out]
                              n983 = Equal?(x=w1408, y=500.0) -> (x = y?=w1407:bool)
                              n984 = local write "IPeak"(w1416) -> ()
                              n985 = Compound Arithmetic op=OR(w1407, w1410, w1409) -> (w1411:bool)
                              n986 = Not(x=w1410) -> (.not. x?=w1419:bool)
                              n987 = Not(x=w1409) -> (.not. x?=w1420:bool)
                              n988 = Compound Arithmetic op=AND(w1407, w1420, w1419) -> (w1406:bool)
                            }
                            n989 = local read "refnum out"() -> (w1403:refnum<file>)
                            n990 = local write "Decrease"(w1402) -> ()
                            n991 = call "Pass_Fail.vi"("OK"=w1402, "Byte Stream File in"=w1403) -> ()  [unwired: 8 in, 2 out]
                          }
                          frame #3 {
                            n992 = local read "refnum out"() -> (w1421:refnum<file>)
                            n993 = call "dataSampled.vi"("refnum in"=w1421) -> ()  [unwired: 9 in, 2 out]
                          }
                        }
                      }
                      frame True {
                        n994 = flat-sequence {
                          tunnel: w1425 -> [w1429]
                          tunnel: w1424 -> [w1428]
                          tunnel: w1423 -> [w1427]
                          tunnel: [w1547] -> w1422
                          frame #0 {
                            w1426 = 0
                            n995 = while {
                              tunnel: w1429 -> [w1432]
                              tunnel: w1428 -> [w1431]
                              tunnel: w1427 -> [w1433]
                              shift-right: [w1434] -> _
                              shift-left: w1426 -> [w1437]
                              shift-right: [w1435] -> _
                              shift-left: w1426 -> [w1436]
                              stop <- w1430 stop-if-true
                              n996 = case shown="0, Default" w1437 {
                                tunnel: w1436 -> [w1448 w1458 w1482 w1490 w1513]
                                tunnel: [w1448 w1458 w1482 w1489 w1513] -> w1435
                                tunnel: [w1441 w1450 3 ("f") w1484 4 ("f")] -> w1434
                                tunnel: w1433 -> [w1440 w1452 _ _ _]
                                tunnel: w1432 -> [_ w1451 _ _ _]
                                tunnel: w1431 -> [_ _ w1477 _ w1506]
                                tunnel: [FALSE FALSE FALSE FALSE w1505] -> w1430
                                frame 0, Default {
                                n997 = Random Number (0-1)() -> (number: 0 to 1=w1447:dbl)
                                n998 = Multiply(x=w1447, y=w1440) -> (x*y=w1446:dbl)
                                n999 = To Long Integer(number=w1446) -> (32bit integer=w1439:i32)
                                "random" <- w1439
                                n1000 = Greater?(x=w1439, y=3) -> (0:w1443:bool)
                                n1001 = Select(t=1, s=w1443, f=0) -> (s? t:f=w1441:i32)
                                }
                                frame 1 {
                                n1002 = Increment(x=w1452) -> (x+1=w1457:dbl)
                                n1003 = while {
                                tunnel: [w1463] -> w1456
                                tunnel: w1451 -> [w1462]
                                tunnel: w1457 -> [w1459]
                                i -> [w1463]
                                stop <- w1464 stop-if-true
                                n1004 = local read "random"() -> (w1461:i32)
                                n1005 = Equal?(x=w1459, y=w1463) -> (x = y?=w1465:bool)
                                n1006 = Index Array(array=w1462, index=w1463) -> (element=w1460:dbl)
                                n1007 = Equal?(x=w1460, y=w1461) -> (x = y?=w1466:bool)
                                n1008 = Or(x=w1466, y=w1465) -> (x .or. y?=w1464:bool)
                                }
                                "index" <- w1456
                                n1009 = Equal?(x=w1456, y=w1457) -> (x = y?=w1453:bool)
                                n1010 = Select(t=0, s=w1453, f=2) -> (s? t:f=w1450:i32)
                                }
                                frame 2 {
                                n1011 = local read "index"() -> (w1476:i32)
                                n1012 = Index Array(array=w1477, index (row)=w1476) -> (element=w1478:dbl[])  [unwired: 1 in]
                                n1013 = Index Array(array=w1478, index #1=0 ("index"), index #2=1 ("index"), index #3=2 ("index")) -> (element #1=w1473:dbl, element #2=w1471:dbl, element #3=w1472:dbl)
                                n1014 = local write "Press Next"(w1473) -> ()
                                n1015 = Subtract(x=w1471, y=40.0) -> (x-y=w1470:dbl)
                                n1016 = Add(x=w1472, y=110.0) -> (x+y=w1469:dbl)
                                n1017 = local write "max(x,y)"(w1469) -> ()
                                n1018 = local write "min(x,y)"(w1470) -> ()
                                }
                                frame 3 {
                                n1019 = while {
                                shift-right: [w1492] -> _
                                shift-left: _ -> [w1493]
                                stop <- w1502 stop-if-true
                                n1020 = local read "currentMaxResistance"() -> (w1495:string)
                                n1021 = local read "EQF1259 com port"() -> (w1501:refnum<visa-resource-name>)
                                n1022 = local read "max(x,y)"() -> (w1500:i16)
                                n1023 = local read "min(x,y)"() -> (w1499:i16)
                                n1024 = call "resistanceScan.vi"("Imax"=w1495, "VISA Refnum in"=w1501) -> ("RESISTANCE/CURRENT"=w1496:cluster{dbl, dbl}, "ADC value"=w1503:dbl, "overCurrent"=w1498:bool, "Istring#"=w1491:string)  [unwired: 5 in, 1 out]
                                n1025 = local write "IRun"(w1491) -> ()
                                n1026 = local write "RESISTANCE/CURRENT"(w1496) -> ()
                                n1027 = local write "overCurrent"(w1498) -> ()
                                n1028 = In Range and Coerce(upper limit=w1500, x=w1503, lower limit=w1499) -> (In Range?=w1497:bool)  [unwired: 1 out]
                                n1029 = call "currentPeak.vi"("Istring# change"=w1493, "Istring# scan"=w1491) -> ("Ipeak"=w1494:string, "Irun"=w1492:string)  [unwired: 7 in, 1 out]
                                n1030 = local write "IPeak"(w1494) -> ()
                                n1031 = local write "QuickResistance"(w1497) -> ()
                                n1032 = Or(x=w1497, y=w1498) -> (x .or. y?=w1502:bool)
                                }
                                n1033 = Increment(x=w1490) -> (x+1=w1489:i32)
                                n1034 = Equal?(x=w1489, y=2) -> (x = y?=w1487:bool)
                                n1035 = Select(t=4, s=w1487, f=0) -> (s? t:f=w1484:i32)
                                }
                                frame 4 {
                                n1036 = Index Array(array=w1506, index (row) #1=1 ("index (row)"), index (col) #1=2 ("disabled index (col)"), index (row) #2=0 ("disabled index (row)"), index (col) #2=1 ("disabled index (col)")) -> (element #1=w1512:dbl, element #2=w1511:dbl)
                                n1037 = while {
                                tunnel: w1512 -> [w1524]
                                tunnel: w1511 -> [w1523]
                                tunnel: [w1517] -> w1505
                                shift-right: [w1515] -> _
                                shift-left: _ -> [w1516]
                                stop <- w1517 stop-if-true
                                n1038 = local read "currentMaxResistance"() -> (w1514:string)
                                n1039 = local read "EQF1259 com port"() -> (w1522:refnum<visa-resource-name>)
                                n1040 = call "resistanceScan.vi"("Imax"=w1514, "VISA Refnum in"=w1522) -> ("RESISTANCE/CURRENT"=w1520:cluster{dbl, dbl}, "ADC value"=w1525:dbl, "overCurrent"=w1521:bool, "Istring#"=w1518:string)  [unwired: 5 in, 1 out]
                                n1041 = local write "IRun"(w1518) -> ()
                                n1042 = local write "RESISTANCE/CURRENT"(w1520) -> ()
                                n1043 = local write "overCurrent"(w1521) -> ()
                                n1044 = call "currentPeak.vi"("Istring# change"=w1516, "Istring# scan"=w1518) -> ("Ipeak"=w1519:string, "Irun"=w1515:string)  [unwired: 7 in, 1 out]
                                n1045 = In Range and Coerce(upper limit=w1524, x=w1525, lower limit=w1523) -> (In Range?=w1517:bool)  [unwired: 1 out]
                                n1046 = local write "IPeak"(w1519) -> ()
                                n1047 = local write "Least"(w1517) -> ()
                                }
                                }
                              }
                            }
                          }
                          frame #1 {
                            # "least"
                            # "current peak"
                            n1048 = local read "IPeak"() -> (w1527:string)
                            n1049 = local read "refnum out"() -> (w1537:refnum<file>)
                            n1050 = call "dataSampled.vi"("Data"=w1527, "refnum in"=w1537) -> ("error out"=w1535:errorcluster, "refnum out"=w1536:refnum<file>)  [unwired: 8 in]
                            n1051 = case shown="False" FALSE {
                              tunnel: w1535 -> [w1541 w1546]
                              tunnel: w1536 -> [w1540 w1545]
                              tunnel: [w1539 w1543] -> w1533
                              tunnel: [w1538 w1542] -> w1530
                              frame True {
                                n1052 = call "dataSampled.vi"("Error In"=w1541, "refnum in"=w1540) -> ("error out"=w1538:errorcluster, "refnum out"=w1539:refnum<file>)  [unwired: 8 in]
                              }
                              frame False {
                                n1053 = local read "QuickResistance"() -> (w1544:bool)
                                n1054 = call "Pass_Fail.vi"("error in (no error)"=w1546, "OK"=w1544, "Byte Stream File in"=w1545) -> ("error out"=w1542:errorcluster, "Byte Stream File out"=w1543:refnum<file>)  [unwired: 7 in]
                              }
                            }
                            n1055 = call "dataSampled.vi"("Error In"=w1530, "refnum in"=w1533) -> ("error out"=w1529:errorcluster, "refnum out"=w1532:refnum<file>)  [unwired: 8 in]
                            n1056 = call "dataSampled.vi"("Error In"=w1529, "refnum in"=w1532) -> ("error out"=w1528:errorcluster, "refnum out"=w1531:refnum<file>)  [unwired: 8 in]
                            n1057 = local read "Least"() -> (w1534:bool)
                            n1058 = call "Pass_Fail.vi"("error in (no error)"=w1528, "OK"=w1534, "Byte Stream File in"=w1531) -> ()  [unwired: 7 in, 2 out]
                          }
                          frame #2 {
                            n1059 = local read "QuickResistance"() -> (w1549:bool)
                            n1060 = local read "Least"() -> (w1550:bool)
                            n1061 = Compound Arithmetic op=AND(w1549, TRUE, w1550) -> (w1547:bool)
                            n1062 = local write "RESISTANCE PASS"(w1547) -> ()
                          }
                        }
                      }
                    }
                  }
                  frame 3 {
                    n1063 = local read "EQF1259 com port"() -> (w1561:refnum<visa-resource-name>)
                    n1064 = call "gearCalculator.vi"("VISA Refnum in"=w1561) -> ("steps/button Array"=w1559:dbl[][], "No Keys"=w1555:bool, "cycle"=w1558:dbl)  [unwired: 10 in, 2 out]
                    n1065 = for {
                      N: w1558 -> [_]
                      tunnel: w1559 -> [w1731]
                      tunnel: [w1730] -> w1560 mode=indexing
                      i -> [w1728]
                      n1066 = Index Array(array=w1731, index (row)=w1728, index (col)=0) -> (element=w1730:dbl)
                    }
                    n1067 = Not(x=w1555) -> (.not. x?=w1556:bool)
                    n1068 = case shown="False" w1556 {
                      tunnel: w1560 -> [_ w1607]
                      tunnel: w1559 -> [_ w1606]
                      tunnel: w1558 -> [_ w1605]
                      tunnel: [TRUE w1604] -> w1557
                      frame False {
                        n1069 = flat-sequence {
                          frame #0 {
                            n1070 = for {
                              N: 2 -> [_]
                              n1071 = local read "refnum out"() -> (w1564:refnum<file>)
                              n1072 = call "dataSampled.vi"("refnum in"=w1564) -> ()  [unwired: 9 in, 2 out]
                            }
                          }
                          frame #1 {
                            n1073 = while {
                              shift-right: [w1578] -> _
                              shift-left: _ -> [w1577]
                              tunnel: [w1569] -> w1566
                              stop <- w1574 stop-if-true
                              n1074 = local read "currentMaxResistance"() -> (w1581:string)
                              n1075 = local read "EQF1259 com port"() -> (w1568:refnum<visa-resource-name>)
                              n1076 = call "resistanceScan.vi"("Imax"=w1581, "VISA Refnum in"=w1568) -> ("error out"=w1580:errorcluster, "RESISTANCE/CURRENT"=w1567:cluster{dbl, dbl}, "ADC value"=w1571:dbl, "Istring#"=w1576:string)  [unwired: 5 in, 1 out]
                              n1077 = local read "overCurrent"() -> (w1572:bool)
                              n1078 = local write "IRun"(w1576) -> ()
                              n1079 = local read "stopR"() -> (w1573:bool)
                              n1080 = call "currentPeak.vi"("error in (no error)"=w1580, "Istring# change"=w1577, "Istring# scan"=w1576) -> ("Ipeak"=w1579:string, "Irun"=w1578:string)  [unwired: 6 in, 1 out]
                              n1081 = local write "RESISTANCE/CURRENT"(w1567) -> ()
                              n1082 = Equal?(x=w1571, y=1000.0) -> (x = y?=w1570:bool)
                              n1083 = local write "IPeak"(w1579) -> ()
                              n1084 = Compound Arithmetic op=OR(w1570, w1573, w1572) -> (w1574:bool)
                              n1085 = Not(x=w1573) -> (.not. x?=w1582:bool)
                              n1086 = Not(x=w1572) -> (.not. x?=w1583:bool)
                              n1087 = Compound Arithmetic op=AND(w1570, w1583, w1582) -> (w1569:bool)
                            }
                            n1088 = local read "refnum out"() -> (w1565:refnum<file>)
                            n1089 = local write "Increase"(w1566) -> ()
                            n1090 = call "Pass_Fail.vi"("OK"=w1566, "Byte Stream File in"=w1565) -> ()  [unwired: 8 in, 2 out]
                          }
                          frame #2 {
                            n1091 = while {
                              shift-right: [w1597] -> _
                              shift-left: _ -> [w1596]
                              tunnel: [w1588] -> w1584
                              stop <- w1593 stop-if-true
                              n1092 = local read "currentMaxResistance"() -> (w1600:string)
                              n1093 = local read "EQF1259 com port"() -> (w1587:refnum<visa-resource-name>)
                              n1094 = call "resistanceScan.vi"("Imax"=w1600, "VISA Refnum in"=w1587) -> ("error out"=w1599:errorcluster, "RESISTANCE/CURRENT"=w1586:cluster{dbl, dbl}, "ADC value"=w1590:dbl, "Istring#"=w1595:string)  [unwired: 5 in, 1 out]
                              n1095 = local read "overCurrent"() -> (w1591:bool)
                              n1096 = local write "IRun"(w1595) -> ()
                              n1097 = local read "stopR"() -> (w1592:bool)
                              n1098 = local write "RESISTANCE/CURRENT"(w1586) -> ()
                              n1099 = call "currentPeak.vi"("error in (no error)"=w1599, "Istring# change"=w1596, "Istring# scan"=w1595) -> ("Ipeak"=w1598:string, "Irun"=w1597:string)  [unwired: 6 in, 1 out]
                              n1100 = Equal?(x=w1590, y=500.0) -> (x = y?=w1589:bool)
                              n1101 = local write "IPeak"(w1598) -> ()
                              n1102 = Compound Arithmetic op=OR(w1589, w1592, w1591) -> (w1593:bool)
                              n1103 = Not(x=w1592) -> (.not. x?=w1601:bool)
                              n1104 = Not(x=w1591) -> (.not. x?=w1602:bool)
                              n1105 = Compound Arithmetic op=AND(w1589, w1602, w1601) -> (w1588:bool)
                            }
                            n1106 = local read "refnum out"() -> (w1585:refnum<file>)
                            n1107 = local write "Decrease"(w1584) -> ()
                            n1108 = call "Pass_Fail.vi"("OK"=w1584, "Byte Stream File in"=w1585) -> ()  [unwired: 8 in, 2 out]
                          }
                          frame #3 {
                            n1109 = local read "refnum out"() -> (w1603:refnum<file>)
                            n1110 = call "dataSampled.vi"("refnum in"=w1603) -> ()  [unwired: 9 in, 2 out]
                          }
                        }
                      }
                      frame True {
                        n1111 = flat-sequence {
                          tunnel: w1607 -> [w1611]
                          tunnel: w1606 -> [w1610]
                          tunnel: w1605 -> [w1609]
                          tunnel: [w1724] -> w1604
                          frame #0 {
                            w1608 = 0
                            n1112 = while {
                              tunnel: w1611 -> [w1614]
                              tunnel: w1610 -> [w1613]
                              tunnel: w1609 -> [w1615]
                              shift-right: [w1616] -> _
                              shift-left: w1608 -> [w1619]
                              shift-right: [w1617] -> _
                              shift-left: w1608 -> [w1618]
                              stop <- w1612 stop-if-true
                              n1113 = case shown="0, Default" w1619 {
                                tunnel: w1618 -> [w1630 w1640 w1664 w1672 w1695]
                                tunnel: [w1630 w1640 w1664 w1671 w1695] -> w1617
                                tunnel: [w1623 w1632 3 ("f") w1666 4 ("f")] -> w1616
                                tunnel: w1615 -> [w1622 w1634 _ _ _]
                                tunnel: w1614 -> [_ w1633 _ _ _]
                                tunnel: w1613 -> [_ _ w1659 _ w1688]
                                tunnel: [FALSE FALSE FALSE FALSE w1687] -> w1612
                                frame 0, Default {
                                n1114 = Random Number (0-1)() -> (number: 0 to 1=w1629:dbl)
                                n1115 = Multiply(x=w1629, y=w1622) -> (x*y=w1628:dbl)
                                n1116 = To Long Integer(number=w1628) -> (32bit integer=w1621:i32)
                                "random 2" <- w1621
                                n1117 = Greater?(x=w1621, y=3) -> (0:w1625:bool)
                                n1118 = Select(t=1, s=w1625, f=0) -> (s? t:f=w1623:i32)
                                }
                                frame 1 {
                                n1119 = Increment(x=w1634) -> (x+1=w1639:dbl)
                                n1120 = while {
                                tunnel: [w1645] -> w1638
                                tunnel: w1633 -> [w1644]
                                tunnel: w1639 -> [w1641]
                                i -> [w1645]
                                stop <- w1646 stop-if-true
                                n1121 = local read "random 2"() -> (w1643:i32)
                                n1122 = Equal?(x=w1641, y=w1645) -> (x = y?=w1647:bool)
                                n1123 = Index Array(array=w1644, index=w1645) -> (element=w1642:dbl)
                                n1124 = Equal?(x=w1642, y=w1643) -> (x = y?=w1648:bool)
                                n1125 = Or(x=w1648, y=w1647) -> (x .or. y?=w1646:bool)
                                }
                                "index 2" <- w1638
                                n1126 = Equal?(x=w1638, y=w1639) -> (x = y?=w1635:bool)
                                n1127 = Select(t=0, s=w1635, f=2) -> (s? t:f=w1632:i32)
                                }
                                frame 2 {
                                n1128 = local read "index 2"() -> (w1658:i32)
                                n1129 = Index Array(array=w1659, index (row)=w1658) -> (element=w1660:dbl[])  [unwired: 1 in]
                                n1130 = Index Array(array=w1660, index #1=0 ("index"), index #2=1 ("index"), index #3=2 ("index")) -> (element #1=w1655:dbl, element #2=w1651:dbl, element #3=w1650:dbl)
                                n1131 = local write "Press Next"(w1655) -> ()
                                n1132 = Subtract(x=w1651, y=40.0) -> (x-y=w1653:dbl)
                                n1133 = Add(x=w1650, y=110.0) -> (x+y=w1652:dbl)
                                n1134 = local write "max(x,y)"(w1652) -> ()
                                n1135 = local write "min(x,y)"(w1653) -> ()
                                }
                                frame 3 {
                                n1136 = while {
                                shift-right: [w1675] -> _
                                shift-left: _ -> [w1676]
                                stop <- w1684 stop-if-true
                                n1137 = local read "currentMaxResistance"() -> (w1673:string)
                                n1138 = local read "EQF1259 com port"() -> (w1683:refnum<visa-resource-name>)
                                n1139 = local read "min(x,y)"() -> (w1681:i16)
                                n1140 = local read "max(x,y)"() -> (w1682:i16)
                                n1141 = call "resistanceScan.vi"("Imax"=w1673, "VISA Refnum in"=w1683) -> ("RESISTANCE/CURRENT"=w1678:cluster{dbl, dbl}, "ADC value"=w1685:dbl, "overCurrent"=w1680:bool, "Istring#"=w1677:string)  [unwired: 5 in, 1 out]
                                n1142 = local write "RESISTANCE/CURRENT"(w1678) -> ()
                                n1143 = call "currentPeak.vi"("Istring# change"=w1676, "Istring# scan"=w1677) -> ("Ipeak"=w1674:string, "Irun"=w1675:string)  [unwired: 7 in, 1 out]
                                n1144 = local write "IRun"(w1677) -> ()
                                n1145 = local write "overCurrent"(w1680) -> ()
                                n1146 = In Range and Coerce(upper limit=w1682, x=w1685, lower limit=w1681) -> (In Range?=w1679:bool)  [unwired: 1 out]
                                n1147 = local write "IPeak"(w1674) -> ()
                                n1148 = Or(x=w1679, y=w1680) -> (x .or. y?=w1684:bool)
                                n1149 = local write "QuickResistance"(w1679) -> ()
                                }
                                n1150 = Increment(x=w1672) -> (x+1=w1671:i32)
                                n1151 = Equal?(x=w1671, y=2) -> (x = y?=w1669:bool)
                                n1152 = Select(t=4, s=w1669, f=0) -> (s? t:f=w1666:i32)
                                }
                                frame 4 {
                                n1153 = Index Array(array=w1688, index (row) #1=1 ("index (row)"), index (col) #1=2 ("disabled index (col)"), index (row) #2=0 ("disabled index (row)"), index (col) #2=1 ("disabled index (col)")) -> (element #1=w1694:dbl, element #2=w1693:dbl)
                                n1154 = while {
                                tunnel: w1694 -> [w1706]
                                tunnel: w1693 -> [w1705]
                                tunnel: [w1696] -> w1687
                                shift-right: [w1698] -> _
                                shift-left: _ -> [w1697]
                                stop <- w1696 stop-if-true
                                n1155 = local read "currentMaxResistance"() -> (w1700:string)
                                n1156 = local read "EQF1259 com port"() -> (w1704:refnum<visa-resource-name>)
                                n1157 = call "resistanceScan.vi"("Imax"=w1700, "VISA Refnum in"=w1704) -> ("RESISTANCE/CURRENT"=w1702:cluster{dbl, dbl}, "ADC value"=w1707:dbl, "overCurrent"=w1703:bool, "Istring#"=w1699:string)  [unwired: 5 in, 1 out]
                                n1158 = local write "IRun"(w1699) -> ()
                                n1159 = local write "RESISTANCE/CURRENT"(w1702) -> ()
                                n1160 = local write "overCurrent"(w1703) -> ()
                                n1161 = In Range and Coerce(upper limit=w1706, x=w1707, lower limit=w1705) -> (In Range?=w1696:bool)  [unwired: 1 out]
                                n1162 = call "currentPeak.vi"("Istring# change"=w1697, "Istring# scan"=w1699) -> ("Ipeak"=w1701:string, "Irun"=w1698:string)  [unwired: 7 in, 1 out]
                                n1163 = local write "IPeak"(w1701) -> ()
                                n1164 = local write "Least"(w1696) -> ()
                                }
                                }
                              }
                            }
                          }
                          frame #1 {
                            # "least"
                            # "current peak"
                            n1165 = local read "IPeak"() -> (w1716:string)
                            n1166 = local read "refnum out"() -> (w1715:refnum<file>)
                            n1167 = call "dataSampled.vi"("Data"=w1716, "refnum in"=w1715) -> ("error out"=w1713:errorcluster, "refnum out"=w1714:refnum<file>)  [unwired: 8 in]
                            n1168 = case shown="False" FALSE {
                              tunnel: w1713 -> [w1719 w1723]
                              tunnel: w1714 -> [w1718 w1722]
                              tunnel: [w1717 w1720] -> w1710
                              frame True {
                                n1169 = call "dataSampled.vi"("Error In"=w1719, "refnum in"=w1718) -> ("refnum out"=w1717:refnum<file>)  [unwired: 8 in, 1 out]
                              }
                              frame False {
                                n1170 = local read "QuickResistance"() -> (w1721:bool)
                                n1171 = call "Pass_Fail.vi"("error in (no error)"=w1723, "OK"=w1721, "Byte Stream File in"=w1722) -> ("Byte Stream File out"=w1720:refnum<file>)  [unwired: 7 in, 1 out]
                              }
                            }
                            n1172 = call "dataSampled.vi"("refnum in"=w1710) -> ("refnum out"=w1709:refnum<file>)  [unwired: 9 in, 1 out]
                            n1173 = call "dataSampled.vi"("refnum in"=w1709) -> ("refnum out"=w1708:refnum<file>)  [unwired: 9 in, 1 out]
                            n1174 = local read "Least"() -> (w1712:bool)
                            n1175 = call "Pass_Fail.vi"("OK"=w1712, "Byte Stream File in"=w1708) -> ()  [unwired: 8 in, 2 out]
                          }
                          frame #2 {
                            n1176 = local read "QuickResistance"() -> (w1727:bool)
                            n1177 = local read "Least"() -> (w1726:bool)
                            n1178 = Compound Arithmetic op=AND(w1727, TRUE, w1726) -> (w1724:bool)
                            n1179 = local write "RESISTANCE PASS"(w1724) -> ()
                          }
                        }
                      }
                    }
                  }
                }
              }
              frame False {
                # "standard"
                n1180 = global read "Global_usbComm.vi" "PartNumber"() -> (w1735:string)
                n1181 = global read "Global_usbComm.vi" "deviceType"() -> (w1732:string)
                n1182 = call "resistanceCalculator.vi"("VISA Refnum in"=w1740, "error in (no error)"=w1737) -> ("No Keys"=w1736:bool, "error out"=w1738:errorcluster)  [unwired: 5 in, 7 out]
                n1183 = Not Equal?(x=w1735, y="400659") -> (x != y?=w1733:bool)
                n1184 = case shown="True" w1733 {
                  tunnel: w1741 -> [_ w1750]
                  tunnel: [w1744 w1749] -> w1739
                  tunnel: w1738 -> [w1744 w1748]
                  tunnel: w1736 -> [_ w1747]
                  tunnel: w1732 -> [_ w1746]
                  frame False {
                    n1185 = local write "RESISTANCE-15"("(W§c6RðS\nN\fÿ\u0006\\\u001c >Pe¦^\u001d ¾n:N7\u0000\u0005ÿ\u00020\n\u0000(W§c6RðS\nN\fÿ\tc\u000bN\u0000Nek\tc®ôv0R1\u00008\u0000\u00020\n\u0000(W§c6RðS\nN\fÿ\u0006\\\u001c >Pe¦^\u001d ¾n:N0\u0000\u0005ÿ\u00020\n\u0000(W§c6RðS\nN\fÿ\tcÏQ;\tc®ôvó\u0007c:y\u00020\n\u0000(W§c6RðS\nN\fÿ\tcX R5u;\tc®ôv0R>f:yúQeg\u00020\n\u0000(W§c6RðS\nN\fÿ\tc\u0000gNOvQ\u0000u\u0000i\u0000c\u0000k\u0000 \u0000R\u0000e\u0000s\u0000i\u0000s\u0000t\u0000a\u0000n\u0000c\u0000e\u0000\tc®\u00020\n\u0000O\u0000n\u0000 \u0000t\u0000h\u0000e\u0000 \u0000c\u0000o\u0000n\u0000s\u0000o\u0000l\u0000e\u0000,\u0000 \u0000s\u0000e\u0000t\u0000 \u0000i\u0000n\u0000c\u0000l\u0000i\u0000n\u0000e\u0000 \u0000t\u0000o\u0000 \u00007\u0000%\u0000.\u0000\n\u0000O\u0000n\u0000 \u0000t\u0000h\u0000e\u0000 \u0000c\u0000o\u0000n\u0000s\u0000o\u0000l\u0000e\u0000,\u0000 \u0000p\u0000r\u0000e\u0000s\u0000s\u0000 \u0000t\u0000h\u0000e\u0000 \u0000n\u0000e\u0000x\u0000t\u0000 \u0000b\u0000u\u0000t\u0000t\u0000o\u0000n\u0000s\u0000 \u0000t\u0000i\u0000l\u0000l\u0000 \u00001\u00008\u0000.\u0000\n\u0000O\u0000n\u0000 \u0000t\u0000h\u0000e\u0000 \u0000c\u0000o\u0000n\u0000s\u0000o\u0000l\u0000e\u0000,\u0000 \u0000s\u0000e\u0000t\u0000 \u0000i\u0000n\u0000c\u0000l\u0000i\u0000n\u0000e\u0000 \u0000t\u0000o\u0000 \u00000\u0000%\u0000.\u0000\n\u0000O\u0000n\u0000 \u0000t\u0000h\u0000e\u0000 \u0000c\u0000o\u0000n\u0000s\u0000o\u0000l\u0000e\u0000,\u0000 \u0000p\u0000r\u0000e\u0000s\u0000s\u0000 \u0000d\u0000e\u0000c\u0000r\u0000e\u0000m\u0000e\u0000n\u0000t\u0000 \u0000r\u0000e\u0000s\u0000i\u0000s\u0000t\u0000a\u0000n\u0000c\u0000e\u0000 \u0000b\u0000u\u0000t\u0000t\u0000o\u0000n\u0000 \u0000t\u0000i\u0000l\u0000l\u0000 \u0000i\u0000n\u0000d\u0000...") -> ()
                  }
                  frame True {
                    n1186 = call "resistancePIP.vi"("error in (no error)"=w1748, "DeviceType"=w1746, "QUICK_KEYS"=w1747, "RESISTANCE"=w1750) -> ("error out"=w1749:errorcluster, "RESISTANCE-15"=→"RESISTANCE-15":string)  [unwired: 6 in]
                  }
                }
                n1187 = case shown="2" w1742 {
                  tunnel: [_ w1755 w1969] -> w1743
                  tunnel: w1739 -> [_ w1754 w1979]
                  tunnel: w1740 -> [_ w1753 w1980]
                  frame 1, Default {
                  }
                  frame 2 {
                    n1188 = flat-sequence {
                      tunnel: [w1771] -> w1763
                      tunnel: [w1764] -> w1762
                      tunnel: [w1767] -> w1761
                      tunnel: w1754 -> [w1766]
                      tunnel: w1753 -> [w1765]
                      tunnel: w1763 -> [w1824]
                      tunnel: [w1824] -> w1760
                      tunnel: w1762 -> [w1823]
                      tunnel: w1761 -> [w1821]
                      tunnel: [w1823] -> w1759
                      tunnel: w1760 -> [w1839]
                      tunnel: [w1839] -> w1758
                      tunnel: w1759 -> [w1838]
                      tunnel: [w1838] -> w1757
                      tunnel: w1758 -> [w1888]
                      tunnel: w1757 -> [w1887]
                      tunnel: [w1887] -> w1756
                      tunnel: w1756 -> [w1930]
                      tunnel: [w1930] -> w1752
                      tunnel: [w1956] -> w1755
                      tunnel: w1752 -> [w1955]
                      frame #0 {
                        n1189 = call "resistanceCalculator.vi"("VISA Refnum in"=w1765, "error in (no error)"=w1766) -> ("steps/button Array"=w1769:dbl[][], "cycle"=w1768:dbl, "No Keys"=w1764:bool)  [unwired: 5 in, 6 out]
                        n1190 = To Long Integer(number=w1768) -> (32bit integer=w1770:i32)
                        n1191 = for {
                          N: w1770 -> [_]
                          tunnel: w1769 -> [w1780]
                          tunnel: [w1775] -> w1772 mode=indexing
                          tunnel: [w1774] -> w1767
                          tunnel: w1764 -> [w1773]
                          i -> [w1779]
                          n1192 = Index Array(array=w1780, index (row)=w1779, index (col)=0 ("disabled index (col)")) -> (element=w1781:dbl)
                          n1193 = Not Equal To 0?(x=w1781) -> (x != 0?=w1777:bool)
                          n1194 = case shown="True" w1777 {
                            selector: w1777 -> [w1804 _]
                            tunnel: w1780 -> [_ w1815]
                            tunnel: w1779 -> [_ w1814]
                            tunnel: [w1804 TRUE] -> w1776
                            frame False {
                            }
                            frame True {
                              n1195 = for {
                                N: 3 -> [_]
                                tunnel: w1815 -> [w1820]
                                tunnel: [w1819] -> w1813 mode=indexing
                                tunnel: w1814 -> [w1818]
                                i -> [w1817]
                                n1196 = Index Array(array=w1820, index (row)=w1818, index (col)=w1817) -> (element=w1819:dbl)
                              }
                              n1197 = Wait (ms)(milliseconds to wait=u32 1250) -> ()  [unwired: 1 out]
                              n1198 = Index Array(array=w1813, index #1=0 ("index"), index #2=1 ("index"), index #3=2 ("index")) -> (element #1=→"Press Next":dbl, element #2=→"resLower":dbl, element #3=→"resUpper":dbl)
                            }
                          }
                          n1199 = case shown="True" w1776 {
                            tunnel: [_ w1784] -> w1775
                            tunnel: [_ w1783] -> w1774
                            tunnel: w1773 -> [w1782 _]
                            frame False {
                              n1200 = local write "QuickResistance"(w1782) -> ()
                            }
                            frame True {
                              n1201 = while {
                                shift-right: [w1793] -> _
                                shift-left: _ -> [w1803]
                                tunnel: [w1800] -> w1784
                                tunnel: [w1785] -> w1783
                                stop <- w1792 stop-if-true
                                n1202 = local read "currentMaxResistance"() -> (w1794:string)
                                n1203 = local read "EQF1259 com port"() -> (w1797:refnum<visa-resource-name>)
                                n1204 = local read "resUpper"() -> (w1788:dbl)
                                n1205 = local read "resLower"() -> (w1798:dbl)
                                n1206 = call "resistanceScan.vi"("Imax"=w1794, "VISA Refnum in"=w1797) -> ("RESISTANCE/CURRENT"=→"RESISTANCE/CURRENT":cluster{dbl, dbl}, "ADC value"=w1800:dbl, "overCurrent"=w1790:bool, "Istring#"=w1799:string)  [unwired: 5 in, 1 out]
                                "IRun" <- w1799
                                "overCurrent" <- w1790
                                n1207 = Subtract(x=w1798, y=40.0) -> (x-y=w1802:dbl)
                                n1208 = Add(x=w1788, y=110.0) -> (x+y=w1789:dbl)
                                n1209 = In Range and Coerce(upper limit=w1789, x=w1800, lower limit=w1802) -> (In Range?=w1786:bool)  [unwired: 1 out]
                                "QuickResistance" <- w1786
                                n1210 = call "currentPeak.vi"("Istring# change"=w1803, "Istring# scan"=w1799) -> ("error out"=w1785:errorcluster, "Ipeak"=→"IPeak":string, "Irun"=w1793:string)  [unwired: 7 in]
                                n1211 = Compound Arithmetic op=OR("stopR", w1790, w1786) -> (w1792:bool)
                              }
                            }
                          }
                        }
                        "resistanceArray" <- w1772
                        n1212 = Decrement(x=w1770) -> (x-1=w1771:i32)
                      }
                      frame #1 {
                        n1213 = local read "refnum out"() -> (w1822:refnum<file>)
                        n1214 = case shown="True" w1823 {
                          tunnel: w1822 -> [w1826 w1833]
                          tunnel: w1821 -> [w1825 w1829]
                          frame True {
                            n1215 = call "dataSampled.vi"("Error In"=w1825, "refnum in"=w1826) -> ("error out"=w1827:errorcluster, "refnum out"=w1828:refnum<file>)  [unwired: 8 in]
                            n1216 = call "dataSampled.vi"("Error In"=w1827, "refnum in"=w1828) -> ()  [unwired: 8 in, 2 out]
                          }
                          frame False {
                            n1217 = local read "IPeak"() -> (w1830:string)
                            n1218 = call "dataSampled.vi"("Error In"=w1829, "Data"=w1830, "refnum in"=w1833) -> ("error out"=w1832:errorcluster, "refnum out"=w1831:refnum<file>)  [unwired: 7 in]
                            n1219 = local read "QuickResistance"() -> (w1834:bool)
                            n1220 = call "Pass_Fail.vi"("error in (no error)"=w1832, "OK"=w1834, "Byte Stream File in"=w1831) -> ()  [unwired: 7 in, 2 out]
                          }
                        }
                      }
                      frame #2 {
                        n1221 = local read "EQF1259 com port"() -> (w1835:refnum<visa-resource-name>)
                        n1222 = case shown="True" w1838 {
                          tunnel: w1835 -> [w1842 w1866]
                          tunnel: [w1840 w1865] -> w1837
                          tunnel: w1839 -> [w1841 _]
                          frame False {
                            n1223 = while {
                              tunnel: w1842 -> [w1857]
                              tunnel: w1841 -> [w1856]
                              shift-right: [w1852] -> _
                              shift-left: _ -> [w1851]
                              tunnel: [w1847] -> w1840
                              stop <- w1848 stop-if-true
                              w1860 = 100.0 ("y")
                              n1224 = local read "resistanceArray"() -> (w1864:dbl[])
                              n1225 = local read "currentMaxResistance"() -> (w1854:string)
                              n1226 = Index Array(array=w1864, index=w1856) -> (element=w1861:dbl)
                              n1227 = Subtract(x=w1861, y=w1860) -> (x-y=w1859:dbl)
                              n1228 = call "resistanceScan.vi"("Imax"=w1854, "VISA Refnum in"=w1857) -> ("error out"=w1843:errorcluster, "RESISTANCE/CURRENT"=w1863:cluster{dbl, dbl}, "ADC value"=w1862:dbl, "Istring#"=w1855:string)  [unwired: 5 in, 1 out]
                              n1229 = local write "IRun"(w1855) -> ()
                              n1230 = local write "RESISTANCE/CURRENT"(w1863) -> ()
                              n1231 = Subtract(x=w1859, y=w1860) -> (x-y=w1858:dbl)
                              n1232 = call "currentPeak.vi"("error in (no error)"=w1843, "Istring# change"=w1851, "Istring# scan"=w1855) -> ("Ipeak"=w1853:string, "Irun"=w1852:string)  [unwired: 6 in, 1 out]
                              n1233 = local read "overCurrent"() -> (w1845:bool)
                              n1234 = local read "stopR"() -> (w1849:bool)
                              n1235 = local write "IPeak"(w1853) -> ()
                              n1236 = In Range and Coerce(upper limit=w1859, x=w1862, lower limit=w1858) -> (In Range?=w1846:bool)  [unwired: 1 out]
                              n1237 = Not(x=w1849) -> (.not. x?=w1850:bool)
                              n1238 = Not(x=w1845) -> (.not. x?=w1844:bool)
                              n1239 = Compound Arithmetic op=OR(w1846, w1845, w1849) -> (w1848:bool)
                              n1240 = Compound Arithmetic op=AND(w1846, w1850, w1844) -> (w1847:bool)
                            }
                            "Decrease" <- w1840
                          }
                          frame True {
                            n1241 = while {
                              tunnel: w1866 -> [w1880]
                              tunnel: [w1873] -> w1865
                              shift-right: [w1878] -> _
                              shift-left: _ -> [w1877]
                              stop <- w1879 stop-if-true
                              n1242 = local read "currentMaxResistance"() -> (w1876:string)
                              n1243 = call "resistanceScan.vi"("Imax"=w1876, "VISA Refnum in"=w1880) -> ("error out"=w1867:errorcluster, "RESISTANCE/CURRENT"=w1883:cluster{dbl, dbl}, "ADC value"=w1882:dbl, "Istring#"=w1875:string)  [unwired: 5 in, 1 out]
                              n1244 = local read "overCurrent"() -> (w1871:bool)
                              n1245 = local write "IRun"(w1875) -> ()
                              n1246 = local write "RESISTANCE/CURRENT"(w1883) -> ()
                              n1247 = local read "stopR"() -> (w1869:bool)
                              n1248 = call "currentPeak.vi"("error in (no error)"=w1867, "Istring# change"=w1877, "Istring# scan"=w1875) -> ("Ipeak"=w1874:string, "Irun"=w1878:string)  [unwired: 6 in, 1 out]
                              n1249 = Greater?(x=w1882, y=1500.0) -> (0:w1870:bool)
                              n1250 = local write "IPeak"(w1874) -> ()
                              n1251 = Compound Arithmetic op=OR(w1870, w1871, w1869) -> (w1879:bool)
                              n1252 = Not(x=w1871) -> (.not. x?=w1868:bool)
                              n1253 = Not(x=w1869) -> (.not. x?=w1872:bool)
                              n1254 = Compound Arithmetic op=AND(w1870, w1868, w1872) -> (w1873:bool)
                            }
                            n1255 = local write "Increase"(w1865) -> ()
                          }
                        }
                        n1256 = local read "refnum out"() -> (w1836:refnum<file>)
                        n1257 = call "Pass_Fail.vi"("OK"=w1837, "Byte Stream File in"=w1836) -> ()  [unwired: 8 in, 2 out]
                      }
                      frame #3 {
                        n1258 = local read "EQF1259 com port"() -> (w1885:refnum<visa-resource-name>)
                        n1259 = case shown="True" w1887 {
                          tunnel: w1888 -> [w1891 _]
                          tunnel: w1885 -> [w1890 w1913]
                          tunnel: [w1889 w1912] -> w1884
                          frame False {
                            n1260 = while {
                              tunnel: w1890 -> [w1907]
                              tunnel: [w1895] -> w1889
                              tunnel: w1891 -> [w1906]
                              shift-right: [w1901] -> _
                              shift-left: _ -> [w1900]
                              stop <- w1896 stop-if-true
                              n1261 = local read "resistanceArray"() -> (w1911:dbl[])
                              n1262 = local read "currentMaxResistance"() -> (w1903:string)
                              n1263 = Index Array(array=w1911, index=w1906) -> (element=w1908:dbl)
                              n1264 = call "resistanceScan.vi"("Imax"=w1903, "VISA Refnum in"=w1907) -> ("RESISTANCE/CURRENT"=w1910:cluster{dbl, dbl}, "ADC value"=w1909:dbl, "Istring#"=w1899:string)  [unwired: 5 in, 2 out]
                              n1265 = Subtract(x=w1908, y=100.0) -> (x-y=w1905:dbl)
                              n1266 = local read "overCurrent"() -> (w1894:bool)
                              n1267 = local write "IRun"(w1899) -> ()
                              n1268 = local read "stopR"() -> (w1897:bool)
                              n1269 = local write "RESISTANCE/CURRENT"(w1910) -> ()
                              n1270 = In Range and Coerce(upper limit=w1908, x=w1909, lower limit=w1905) -> (In Range?=w1893:bool)  [unwired: 1 out]
                              n1271 = call "currentPeak.vi"("Istring# change"=w1900, "Istring# scan"=w1899) -> ("Ipeak"=w1902:string, "Irun"=w1901:string)  [unwired: 7 in, 1 out]
                              n1272 = local write "IPeak"(w1902) -> ()
                              n1273 = Compound Arithmetic op=OR(w1894, w1893, w1897) -> (w1896:bool)
                              n1274 = Not(x=w1897) -> (.not. x?=w1898:bool)
                              n1275 = Not(x=w1894) -> (.not. x?=w1892:bool)
                              n1276 = Compound Arithmetic op=AND(w1893, w1898, w1892) -> (w1895:bool)
                            }
                            "Increase" <- w1889
                          }
                          frame True {
                            n1277 = while {
                              tunnel: w1913 -> [w1928]
                              tunnel: [w1919] -> w1912
                              shift-right: [w1925] -> _
                              shift-left: _ -> [w1924]
                              stop <- w1918 stop-if-true
                              n1278 = local read "currentMaxResistance"() -> (w1927:string)
                              n1279 = call "resistanceScan.vi"("Imax"=w1927, "VISA Refnum in"=w1928) -> ("RESISTANCE/CURRENT"=w1929:cluster{dbl, dbl}, "ADC value"=w1914:dbl, "Istring#"=w1926:string)  [unwired: 5 in, 2 out]
                              n1280 = local read "overCurrent"() -> (w1916:bool)
                              n1281 = local write "IRun"(w1926) -> ()
                              n1282 = local write "RESISTANCE/CURRENT"(w1929) -> ()
                              n1283 = local read "stopR"() -> (w1917:bool)
                              n1284 = call "currentPeak.vi"("Istring# change"=w1924, "Istring# scan"=w1926) -> ("Ipeak"=w1923:string, "Irun"=w1925:string)  [unwired: 7 in, 1 out]
                              n1285 = Less?(x=w1914, y=825.0 ("x")) -> (x < y?=w1920:bool)
                              n1286 = local write "IPeak"(w1923) -> ()
                              n1287 = Compound Arithmetic op=OR(w1916, w1920, w1917) -> (w1918:bool)
                              n1288 = Not(x=w1916) -> (.not. x?=w1922:bool)
                              n1289 = Not(x=w1917) -> (.not. x?=w1921:bool)
                              n1290 = Compound Arithmetic op=AND(w1920, w1922, w1921) -> (w1919:bool)
                            }
                            n1291 = local write "Decrease"(w1912) -> ()
                          }
                        }
                        n1292 = local read "refnum out"() -> (w1886:refnum<file>)
                        n1293 = call "Pass_Fail.vi"("OK"=w1884, "Byte Stream File in"=w1886) -> ()  [unwired: 8 in, 2 out]
                      }
                      frame #4 {
                        n1294 = local read "EQF1259 com port"() -> (w1931:refnum<visa-resource-name>)
                        n1295 = case shown="True" w1930 {
                          tunnel: [w1935 TRUE] -> w1932
                          tunnel: w1931 -> [w1934 _]
                          frame False {
                            n1296 = while {
                              tunnel: [w1944] -> w1935
                              tunnel: w1934 -> [w1950]
                              shift-right: [w1947] -> _
                              shift-left: _ -> [w1945]
                              stop <- w1943 stop-if-true
                              n1297 = local read "currentMaxResistance"() -> (w1949:string)
                              n1298 = call "resistanceScan.vi"("Imax"=w1949, "VISA Refnum in"=w1950) -> ("RESISTANCE/CURRENT"=w1952:cluster{dbl, dbl}, "ADC value"=w1951:dbl, "Istring#"=w1948:string)  [unwired: 5 in, 2 out]
                              n1299 = local write "IRun"(w1948) -> ()
                              n1300 = local write "RESISTANCE/CURRENT"(w1952) -> ()
                              n1301 = call "currentPeak.vi"("Istring# change"=w1945, "Istring# scan"=w1948) -> ("Ipeak"=w1946:string, "Irun"=w1947:string)  [unwired: 7 in, 1 out]
                              n1302 = local read "overCurrent"() -> (w1939:bool)
                              n1303 = In Range and Coerce(upper limit=600.0, x=w1951, lower limit=400.0) -> (In Range?=w1940:bool)  [unwired: 1 out]
                              n1304 = local read "stopR"() -> (w1941:bool)
                              n1305 = local write "IPeak"(w1946) -> ()
                              n1306 = Not(x=w1941) -> (.not. x?=w1942:bool)
                              n1307 = Not(x=w1939) -> (.not. x?=w1938:bool)
                              n1308 = Compound Arithmetic op=OR(w1940, w1939, w1941) -> (w1943:bool)
                              n1309 = Compound Arithmetic op=AND(w1940, w1942, w1938) -> (w1944:bool)
                            }
                            n1310 = local read "refnum out"() -> (w1933:refnum<file>)
                            n1311 = call "Pass_Fail.vi"("OK"=w1935, "Byte Stream File in"=w1933) -> ()  [unwired: 8 in, 2 out]
                          }
                          frame True {
                            n1312 = local read "refnum out"() -> (w1953:refnum<file>)
                            n1313 = call "dataSampled.vi"("refnum in"=w1953) -> ()  [unwired: 9 in, 2 out]
                          }
                        }
                        "Least" <- w1932
                      }
                      frame #5 {
                        n1314 = case shown="True" w1955 {
                          tunnel: [w1957 w1963] -> w1956
                          frame False {
                            n1315 = local read "QuickResistance"() -> (w1959:bool)
                            n1316 = local read "Decrease"() -> (w1960:bool)
                            n1317 = local read "Increase"() -> (w1961:bool)
                            n1318 = local read "Least"() -> (w1962:bool)
                            n1319 = Compound Arithmetic op=AND(TRUE, w1959, w1960, w1961, w1962) -> (w1957:bool)
                          }
                          frame True {
                            n1320 = local read "Decrease"() -> (w1965:bool)
                            n1321 = local read "Increase"() -> (w1966:bool)
                            n1322 = Compound Arithmetic op=AND(TRUE, w1965, w1966) -> (w1963:bool)
                          }
                        }
                        "RESISTANCE PASS" <- w1956
                      }
                    }
                  }
                  frame 3 {
                    n1323 = flat-sequence {
                      tunnel: w1980 -> [w1989]
                      tunnel: w1979 -> [w1988]
                      tunnel: [w1984] -> w1978
                      tunnel: [w1983] -> w1977
                      tunnel: [w1981] -> w1972
                      tunnel: w1978 -> [w2038]
                      tunnel: w1977 -> [w2037]
                      tunnel: [w2037] -> w1976
                      tunnel: [w2036] -> w1973
                      tunnel: w1972 -> [w2036]
                      tunnel: [w2033] -> w1968
                      tunnel: w1976 -> [w2050]
                      tunnel: [w2050] -> w1975
                      tunnel: w1973 -> [w2049]
                      tunnel: [w2049] -> w1971
                      tunnel: w1968 -> [w2048]
                      tunnel: [w2048] -> w1967
                      tunnel: w1975 -> [w2123]
                      tunnel: [w2123] -> w1974
                      tunnel: w1971 -> [w2122]
                      tunnel: w1967 -> [w2121]
                      tunnel: w1974 -> [w2190]
                      tunnel: [w2190] -> w1970
                      tunnel: w1970 -> [w2216]
                      tunnel: [w2215] -> w1969
                      frame #0 {
                        n1324 = call "gearCalculator.vi"("VISA Refnum in"=w1989, "error in (no error)"=w1988) -> ("steps/button Array"=w1986:dbl[][], "No Keys"=w1983:bool, "cycle"=w1987:dbl)  [unwired: 9 in, 2 out]
                        n1325 = To Long Integer(number=w1987) -> (32bit integer=w1982:i32)
                        n1326 = for {
                          N: w1982 -> [_]
                          tunnel: w1986 -> [w1993]
                          tunnel: [w1991] -> w1985 mode=indexing
                          tunnel: [w1990] -> w1984
                          i -> [w1994]
                          n1327 = Index Array(array=w1993, index (row)=w1994, index (col)=0 ("disabled index (col)")) -> (element=w1996:dbl)
                          n1328 = Not Equal To 0?(x=w1996) -> (x != 0?=w1995:bool)
                          n1329 = case shown="True" w1995 {
                            selector: w1995 -> [w2017 _]
                            tunnel: w1993 -> [_ w2026]
                            tunnel: w1994 -> [_ w2025]
                            tunnel: [w2017 TRUE] -> w1992
                            frame False {
                            }
                            frame True {
                              n1330 = for {
                                N: 2 -> [_]
                                tunnel: w2026 -> [w2031]
                                tunnel: w2025 -> [w2029]
                                tunnel: [w2028] -> w2024 mode=indexing
                                i -> [w2030]
                                n1331 = Index Array(array=w2031, index (row)=w2029, index (col)=w2030) -> (element=w2028:dbl)
                              }
                              n1332 = Wait (ms)(milliseconds to wait=u32 1250) -> ()  [unwired: 1 out]
                              n1333 = Index Array(array=w2024, index #1=0 ("index"), index #2=1 ("index")) -> (element #1=w2020:dbl, element #2=→"valueResistance":dbl)
                              n1334 = local write "Press Next"(w2020) -> ()
                            }
                          }
                          n1335 = case shown="True" w1992 {
                            tunnel: [_ w1999] -> w1991
                            tunnel: [_ w1998] -> w1990
                            frame False {
                            }
                            frame True {
                              n1336 = while {
                                shift-right: [w2009] -> _
                                shift-left: _ -> [w2008]
                                tunnel: [w2002] -> w1999
                                tunnel: [w2001] -> w1998
                                stop <- w2016 stop-if-true
                                w2013 = 10.0
                                n1337 = local read "currentMaxResistance"() -> (w2005:string)
                                n1338 = local read "EQF1259 com port"() -> (w2004:refnum<visa-resource-name>)
                                n1339 = local read "valueResistance"() -> (w2010:dbl)
                                n1340 = Add(x=w2010, y=w2013) -> (x+y=w2012:dbl)
                                n1341 = Subtract(x=w2010, y=w2013) -> (x-y=w2011:dbl)
                                n1342 = call "resistanceScan.vi"("Imax"=w2005, "VISA Refnum in"=w2004) -> ("error out"=w2001:errorcluster, "RESISTANCE/CURRENT"=w2007:cluster{dbl, dbl}, "ADC value"=w2002:dbl, "overCurrent"=w2006:bool, "Istring#"=w2003:string)  [unwired: 5 in]
                                n1343 = local read "stopR"() -> (w2015:bool)
                                n1344 = local write "IRun"(w2003) -> ()
                                n1345 = local write "RESISTANCE/CURRENT"(w2007) -> ()
                                n1346 = local write "overCurrent"(w2006) -> ()
                                n1347 = In Range and Coerce(upper limit=w2012, x=w2002, lower limit=w2011) -> (In Range?=w2014:bool)  [unwired: 1 out]
                                n1348 = call "currentPeak.vi"("Istring# change"=w2008, "Istring# scan"=w2003) -> ("Ipeak"=w2000:string, "Irun"=w2009:string)  [unwired: 7 in, 1 out]
                                n1349 = local write "QuickResistance"(w2014) -> ()
                                n1350 = local write "IPeak"(w2000) -> ()
                                n1351 = Compound Arithmetic op=OR(w2014, w2006, w2015) -> (w2016:bool)
                              }
                            }
                          }
                        }
                        n1352 = local write "resistanceArray"(w1985) -> ()
                        n1353 = Decrement(x=w1982) -> (x-1=w1981:i32)
                      }
                      frame #1 {
                        n1354 = local read "refnum out"() -> (w2041:refnum<file>)
                        n1355 = local read "IPeak"() -> (w2032:string)
                        n1356 = call "dataSampled.vi"("Error In"=w2038, "Data"=w2032, "refnum in"=w2041) -> ("error out"=w2039:errorcluster, "refnum out"=w2040:refnum<file>)  [unwired: 7 in]
                        n1357 = case shown="False" w2037 {
                          selector: w2037 -> [w2042 _]
                          tunnel: w2039 -> [w2044 w2047]
                          tunnel: w2040 -> [w2043 w2046]
                          frame True {
                            n1358 = call "dataSampled.vi"("Error In"=w2044, "refnum in"=w2043) -> ()  [unwired: 8 in, 2 out]
                            n1359 = local write "QuickResistance"(w2042) -> ()
                          }
                          frame False {
                            n1360 = local read "QuickResistance"() -> (w2045:bool)
                            n1361 = call "Pass_Fail.vi"("error in (no error)"=w2047, "OK"=w2045, "Byte Stream File in"=w2046) -> ()  [unwired: 7 in, 2 out]
                          }
                        }
                        n1362 = global read "Global_usbComm.vi" "PartNumber"() -> (w2035:string)
                        n1363 = Not Equal?(x=w2035, y="400659") -> (x != y?=w2033:bool)
                      }
                      frame #2 {
                        n1364 = case shown="False" w2048 {
                          tunnel: w2050 -> [_ w2073]
                          tunnel: w2049 -> [_ w2071]
                          frame False {
                            # "for EBNT71017V1 only"
                            n1365 = while {
                              shift-right: [w2064] -> _
                              shift-left: _ -> [w2065]
                              tunnel: [w2054] -> w2052
                              stop <- w2058 stop-if-true
                              n1366 = local read "currentMaxResistance"() -> (w2070:string)
                              n1367 = local read "EQF1259 com port"() -> (w2053:refnum<visa-resource-name>)
                              n1368 = call "resistanceScan.vi"("Imax"=w2070, "VISA Refnum in"=w2053) -> ("error out"=w2068:errorcluster, "RESISTANCE/CURRENT"=w2069:cluster{dbl, dbl}, "ADC value"=w2063:dbl, "Istring#"=w2066:string)  [unwired: 5 in, 1 out]
                              n1369 = local write "IRun"(w2066) -> ()
                              n1370 = local write "RESISTANCE/CURRENT"(w2069) -> ()
                              n1371 = call "currentPeak.vi"("error in (no error)"=w2068, "Istring# change"=w2065, "Istring# scan"=w2066) -> ("Ipeak"=w2067:string, "Irun"=w2064:string)  [unwired: 6 in, 1 out]
                              n1372 = local read "overCurrent"() -> (w2059:bool)
                              n1373 = local write "IPeak"(w2067) -> ()
                              n1374 = In Range and Coerce(upper limit=2070.0, x=w2063, lower limit=1734.0) -> (In Range?=w2055:bool)  [unwired: 1 out]
                              n1375 = local read "stopR"() -> (w2060:bool)
                              n1376 = Not(x=w2060) -> (.not. x?=w2057:bool)
                              n1377 = Not(x=w2059) -> (.not. x?=w2056:bool)
                              n1378 = Compound Arithmetic op=OR(w2055, w2059, w2060) -> (w2058:bool)
                              n1379 = Compound Arithmetic op=AND(w2055, w2057, w2056) -> (w2054:bool)
                            }
                            n1380 = local read "refnum out"() -> (w2051:refnum<file>)
                            n1381 = local write "Decrease"(w2052) -> ()
                            n1382 = call "Pass_Fail.vi"("OK"=w2052, "Byte Stream File in"=w2051) -> ()  [unwired: 8 in, 2 out]
                          }
                          frame True {
                            n1383 = local read "EQF1259 com port"() -> (w2072:refnum<visa-resource-name>)
                            n1384 = case shown="False" w2073 {
                              tunnel: [w2076 w2101] -> w2075
                              tunnel: w2072 -> [w2078 w2102]
                              tunnel: w2071 -> [w2077 w2103]
                              frame False {
                                n1385 = while {
                                tunnel: [w2095] -> w2076
                                shift-right: [w2085] -> _
                                shift-left: _ -> [w2084]
                                tunnel: w2078 -> [w2079]
                                tunnel: w2077 -> [w2080]
                                stop <- w2098 stop-if-true
                                w2089 = 100.0
                                n1386 = local read "resistanceArray"() -> (w2094:dbl[])
                                n1387 = local read "currentMaxResistance"() -> (w2082:string)
                                n1388 = Index Array(array=w2094, index=w2080) -> (element=w2093:dbl)
                                n1389 = Subtract(x=w2093, y=w2089) -> (x-y=w2090:dbl)
                                n1390 = call "resistanceScan.vi"("Imax"=w2082, "VISA Refnum in"=w2079) -> ("error out"=w2083:errorcluster, "RESISTANCE/CURRENT"=w2081:cluster{dbl, dbl}, "ADC value"=w2091:dbl, "Istring#"=w2086:string)  [unwired: 5 in, 1 out]
                                n1391 = local write "IRun"(w2086) -> ()
                                n1392 = local write "RESISTANCE/CURRENT"(w2081) -> ()
                                n1393 = Subtract(x=w2090, y=w2089) -> (x-y=w2092:dbl)
                                n1394 = call "currentPeak.vi"("error in (no error)"=w2083, "Istring# change"=w2084, "Istring# scan"=w2086) -> ("Ipeak"=w2087:string, "Irun"=w2085:string)  [unwired: 6 in, 1 out]
                                n1395 = local read "overCurrent"() -> (w2097:bool)
                                n1396 = local read "stopR"() -> (w2096:bool)
                                n1397 = local write "IPeak"(w2087) -> ()
                                n1398 = In Range and Coerce(upper limit=w2090, x=w2091, lower limit=w2092) -> (In Range?=w2088:bool)  [unwired: 1 out]
                                n1399 = Not(x=w2096) -> (.not. x?=w2099:bool)
                                n1400 = Not(x=w2097) -> (.not. x?=w2100:bool)
                                n1401 = Compound Arithmetic op=OR(w2088, w2097, w2096) -> (w2098:bool)
                                n1402 = Compound Arithmetic op=AND(w2088, w2099, w2100) -> (w2095:bool)
                                }
                                n1403 = local write "Decrease"(w2076) -> ()
                              }
                              frame True {
                                n1404 = while {
                                shift-right: [w2120] -> _
                                shift-left: _ -> [w2119]
                                tunnel: [w2114] -> w2101
                                tunnel: w2103 -> [_]
                                tunnel: w2102 -> [w2104]
                                stop <- w2109 stop-if-true
                                n1405 = local read "currentMaxResistance"() -> (w2105:string)
                                n1406 = call "resistanceScan.vi"("Imax"=w2105, "VISA Refnum in"=w2104) -> ("error out"=w2115:errorcluster, "RESISTANCE/CURRENT"=w2116:cluster{dbl, dbl}, "ADC value"=w2111:dbl, "Istring#"=w2118:string)  [unwired: 5 in, 1 out]
                                n1407 = local read "overCurrent"() -> (w2107:bool)
                                n1408 = local write "IRun"(w2118) -> ()
                                n1409 = local write "RESISTANCE/CURRENT"(w2116) -> ()
                                n1410 = local read "stopR"() -> (w2108:bool)
                                n1411 = call "currentPeak.vi"("error in (no error)"=w2115, "Istring# change"=w2119, "Istring# scan"=w2118) -> ("Ipeak"=w2117:string, "Irun"=w2120:string)  [unwired: 6 in, 1 out]
                                n1412 = Greater?(x=w2111, y=1000.0) -> (0:w2106:bool)
                                n1413 = local write "IPeak"(w2117) -> ()
                                n1414 = Compound Arithmetic op=OR(w2106, w2107, w2108) -> (w2109:bool)
                                n1415 = Not(x=w2107) -> (.not. x?=w2112:bool)
                                n1416 = Not(x=w2108) -> (.not. x?=w2113:bool)
                                n1417 = Compound Arithmetic op=AND(w2106, w2112, w2113) -> (w2114:bool)
                                }
                                n1418 = local write "Increase"(w2101) -> ()
                              }
                            }
                            n1419 = local read "refnum out"() -> (w2074:refnum<file>)
                            n1420 = call "Pass_Fail.vi"("OK"=w2075, "Byte Stream File in"=w2074) -> ()  [unwired: 8 in, 2 out]
                          }
                        }
                      }
                      frame #3 {
                        n1421 = case shown="False" w2121 {
                          tunnel: w2123 -> [_ w2146]
                          tunnel: w2122 -> [_ w2145]
                          frame False {
                            # "for EBNT71017V1 only"
                            n1422 = while {
                              shift-right: [w2137] -> _
                              shift-left: _ -> [w2138]
                              tunnel: [w2127] -> w2125
                              stop <- w2131 stop-if-true
                              n1423 = local read "currentMaxResistance"() -> (w2143:string)
                              n1424 = local read "EQF1259 com port"() -> (w2126:refnum<visa-resource-name>)
                              n1425 = call "resistanceScan.vi"("Imax"=w2143, "VISA Refnum in"=w2126) -> ("error out"=w2141:errorcluster, "RESISTANCE/CURRENT"=w2142:cluster{dbl, dbl}, "ADC value"=w2136:dbl, "Istring#"=w2139:string)  [unwired: 5 in, 1 out]
                              n1426 = local write "IRun"(w2139) -> ()
                              n1427 = local write "RESISTANCE/CURRENT"(w2142) -> ()
                              n1428 = call "currentPeak.vi"("error in (no error)"=w2141, "Istring# change"=w2138, "Istring# scan"=w2139) -> ("Ipeak"=w2140:string, "Irun"=w2137:string)  [unwired: 6 in, 1 out]
                              n1429 = local read "overCurrent"() -> (w2132:bool)
                              n1430 = local write "IPeak"(w2140) -> ()
                              n1431 = In Range and Coerce(upper limit=2458.0, x=w2136, lower limit=2251.0) -> (In Range?=w2128:bool)  [unwired: 1 out]
                              n1432 = local read "stopR"() -> (w2133:bool)
                              n1433 = Not(x=w2133) -> (.not. x?=w2130:bool)
                              n1434 = Not(x=w2132) -> (.not. x?=w2129:bool)
                              n1435 = Compound Arithmetic op=OR(w2128, w2132, w2133) -> (w2131:bool)
                              n1436 = Compound Arithmetic op=AND(w2128, w2130, w2129) -> (w2127:bool)
                            }
                            n1437 = local read "refnum out"() -> (w2124:refnum<file>)
                            n1438 = local write "Increase"(w2125) -> ()
                            n1439 = call "Pass_Fail.vi"("OK"=w2125, "Byte Stream File in"=w2124) -> ()  [unwired: 8 in, 2 out]
                          }
                          frame True {
                            n1440 = local read "EQF1259 com port"() -> (w2147:refnum<visa-resource-name>)
                            n1441 = case shown="True" w2146 {
                              tunnel: w2147 -> [w2151 w2173]
                              tunnel: [w2149 w2172] -> w2144
                              tunnel: w2145 -> [w2150 _]
                              frame False {
                                n1442 = while {
                                tunnel: w2151 -> [w2167]
                                tunnel: [w2156] -> w2149
                                shift-right: [w2162] -> _
                                shift-left: _ -> [w2161]
                                tunnel: w2150 -> [w2152]
                                stop <- w2157 stop-if-true
                                n1443 = local read "resistanceArray"() -> (w2171:dbl[])
                                n1444 = local read "currentMaxResistance"() -> (w2164:string)
                                n1445 = Index Array(array=w2171, index=w2152) -> (element=w2168:dbl)
                                n1446 = call "resistanceScan.vi"("Imax"=w2164, "VISA Refnum in"=w2167) -> ("RESISTANCE/CURRENT"=w2170:cluster{dbl, dbl}, "ADC value"=w2169:dbl, "Istring#"=w2160:string)  [unwired: 5 in, 2 out]
                                n1447 = Subtract(x=w2168, y=100.0) -> (x-y=w2166:dbl)
                                n1448 = local read "overCurrent"() -> (w2155:bool)
                                n1449 = local write "IRun"(w2160) -> ()
                                n1450 = local read "stopR"() -> (w2158:bool)
                                n1451 = local write "RESISTANCE/CURRENT"(w2170) -> ()
                                n1452 = In Range and Coerce(upper limit=w2168, x=w2169, lower limit=w2166) -> (In Range?=w2154:bool)  [unwired: 1 out]
                                n1453 = call "currentPeak.vi"("Istring# change"=w2161, "Istring# scan"=w2160) -> ("Ipeak"=w2163:string, "Irun"=w2162:string)  [unwired: 7 in, 1 out]
                                n1454 = local write "IPeak"(w2163) -> ()
                                n1455 = Compound Arithmetic op=OR(w2155, w2154, w2158) -> (w2157:bool)
                                n1456 = Not(x=w2158) -> (.not. x?=w2159:bool)
                                n1457 = Not(x=w2155) -> (.not. x?=w2153:bool)
                                n1458 = Compound Arithmetic op=AND(w2154, w2159, w2153) -> (w2156:bool)
                                }
                                n1459 = local write "Increase"(w2149) -> ()
                              }
                              frame True {
                                n1460 = while {
                                tunnel: w2173 -> [w2188]
                                tunnel: [w2179] -> w2172
                                shift-right: [w2185] -> _
                                shift-left: _ -> [w2184]
                                stop <- w2178 stop-if-true
                                n1461 = local read "currentMaxResistance"() -> (w2187:string)
                                n1462 = call "resistanceScan.vi"("Imax"=w2187, "VISA Refnum in"=w2188) -> ("RESISTANCE/CURRENT"=w2189:cluster{dbl, dbl}, "ADC value"=w2174:dbl, "Istring#"=w2186:string)  [unwired: 5 in, 2 out]
                                n1463 = local read "overCurrent"() -> (w2176:bool)
                                n1464 = local write "IRun"(w2186) -> ()
                                n1465 = local write "RESISTANCE/CURRENT"(w2189) -> ()
                                n1466 = local read "stopR"() -> (w2177:bool)
                                n1467 = call "currentPeak.vi"("Istring# change"=w2184, "Istring# scan"=w2186) -> ("Ipeak"=w2183:string, "Irun"=w2185:string)  [unwired: 7 in, 1 out]
                                n1468 = Less?(x=w2174, y=500.0 ("x")) -> (x < y?=w2180:bool)
                                n1469 = local write "IPeak"(w2183) -> ()
                                n1470 = Compound Arithmetic op=OR(w2176, w2180, w2177) -> (w2178:bool)
                                n1471 = Not(x=w2176) -> (.not. x?=w2182:bool)
                                n1472 = Not(x=w2177) -> (.not. x?=w2181:bool)
                                n1473 = Compound Arithmetic op=AND(w2180, w2182, w2181) -> (w2179:bool)
                                }
                                n1474 = local write "Decrease"(w2172) -> ()
                              }
                            }
                            n1475 = local read "refnum out"() -> (w2148:refnum<file>)
                            n1476 = call "Pass_Fail.vi"("OK"=w2144, "Byte Stream File in"=w2148) -> ()  [unwired: 8 in, 2 out]
                          }
                        }
                      }
                      frame #4 {
                        n1477 = local read "EQF1259 com port"() -> (w2191:refnum<visa-resource-name>)
                        n1478 = case shown="False" w2190 {
                          tunnel: [w2195 TRUE] -> w2192
                          tunnel: w2191 -> [w2194 _]
                          frame False {
                            n1479 = while {
                              tunnel: [w2204] -> w2195
                              tunnel: w2194 -> [w2210]
                              shift-right: [w2207] -> _
                              shift-left: _ -> [w2205]
                              stop <- w2203 stop-if-true
                              n1480 = local read "currentMaxResistance"() -> (w2209:string)
                              n1481 = call "resistanceScan.vi"("Imax"=w2209, "VISA Refnum in"=w2210) -> ("RESISTANCE/CURRENT"=w2212:cluster{dbl, dbl}, "ADC value"=w2211:dbl, "Istring#"=w2208:string)  [unwired: 5 in, 2 out]
                              n1482 = local write "IRun"(w2208) -> ()
                              n1483 = local write "RESISTANCE/CURRENT"(w2212) -> ()
                              n1484 = call "currentPeak.vi"("Istring# change"=w2205, "Istring# scan"=w2208) -> ("Ipeak"=w2206:string, "Irun"=w2207:string)  [unwired: 7 in, 1 out]
                              n1485 = local read "overCurrent"() -> (w2199:bool)
                              n1486 = In Range and Coerce(upper limit=310.0, x=w2211, lower limit=194.0) -> (In Range?=w2200:bool)  [unwired: 1 out]
                              n1487 = local read "stopR"() -> (w2201:bool)
                              n1488 = local write "IPeak"(w2206) -> ()
                              n1489 = Not(x=w2201) -> (.not. x?=w2202:bool)
                              n1490 = Not(x=w2199) -> (.not. x?=w2198:bool)
                              n1491 = Compound Arithmetic op=OR(w2200, w2199, w2201) -> (w2203:bool)
                              n1492 = Compound Arithmetic op=AND(w2200, w2202, w2198) -> (w2204:bool)
                            }
                            n1493 = local read "refnum out"() -> (w2193:refnum<file>)
                            n1494 = call "Pass_Fail.vi"("OK"=w2195, "Byte Stream File in"=w2193) -> ()  [unwired: 8 in, 2 out]
                          }
                          frame True {
                            n1495 = local read "refnum out"() -> (w2213:refnum<file>)
                            n1496 = call "dataSampled.vi"("refnum in"=w2213) -> ()  [unwired: 9 in, 2 out]
                          }
                        }
                        n1497 = local write "Least"(w2192) -> ()
                      }
                      frame #5 {
                        n1498 = case shown="False" w2216 {
                          tunnel: [w2217 w2223] -> w2215
                          frame False {
                            n1499 = local read "QuickResistance"() -> (w2219:bool)
                            n1500 = local read "Decrease"() -> (w2220:bool)
                            n1501 = local read "Increase"() -> (w2221:bool)
                            n1502 = local read "Least"() -> (w2222:bool)
                            n1503 = Compound Arithmetic op=AND(TRUE, w2219, w2220, w2221, w2222) -> (w2217:bool)
                          }
                          frame True {
                            n1504 = local read "Decrease"() -> (w2225:bool)
                            n1505 = local read "Increase"() -> (w2226:bool)
                            n1506 = Compound Arithmetic op=AND(TRUE, w2225, w2226) -> (w2223:bool)
                          }
                        }
                        n1507 = local write "RESISTANCE PASS"(w2215) -> ()
                      }
                    }
                  }
                }
              }
            }
          }
        }
        n1508 = Select(t=T3."Incline" ("Tab Control"), s=w1344, f=T3."Failed" ("Tab Control")) -> (s? t:f=w1347:T3)
      }
      frame "Pulse" {
        w2227 = FALSE
        n1509 = local write "BLE PULSE"(u32 0 ("Waveform Chart")) -> ()
        n1510 = local write "PUL0"(w2227) -> ()
        n1511 = local write "PUL1"(w2227) -> ()
        n1512 = property on="BLE PULSE" class="WFChart (strict)"("History Data"=u32[] []) -> ()  [unwired: 2 in, 2 out]
        n1513 = local write "Hand/Thumb Pass"(w2227) -> ()
        n1514 = local write "BLE_HRM Pass"(w2227) -> ()
        n1515 = local write "E-stopHRM"(w2227) -> ()
        n1516 = global read "Global_usbComm.vi" "pulseType"() -> (w2228:string)
        n1517 = Not Equal?(x=w2228, y="1") -> (x != y?=w2235:bool)
        n1518 = case shown="True" w2235 {
          tunnel: [TRUE w2241] -> w2234
          frame False {
            n1519 = local read "refnum out"() -> (w2240:refnum<file>)
            n1520 = call "dataSampled.vi"("refnum in"=w2240) -> ()  [unwired: 9 in, 2 out]
          }
          frame True {
            n1521 = local read "EQF1259 com port"() -> (w2248:refnum<visa-resource-name>)
            n1522 = call "usbCommand.vi"("write buffer"="'\u0001", "VISA resource name in"=w2248) -> ("error out"=w2251:errorcluster)  [unwired: 8 in, 1 out]
            n1523 = call "pulsePIP.vi"("error in (no error)"=w2251) -> ("error out"=w2247:errorcluster, "PULSE-17"=→"PULSE-17":string)  [unwired: 9 in]
            n1524 = while {
              shift-right: [w2260] -> _
              shift-left: T6."verifyHand_Thumb" -> [w2261]
              tunnel: w2248 -> [w2258]
              tunnel: w2247 -> [w2257]
              tunnel: [w2257] -> w2246
              tunnel: [w2256] -> w2245
              tunnel: [w2255] -> w2244
              stop <- w2259 stop-if-true
              n1525 = case shown="\"statusBLE_HRM\"" w2261 {
                tunnel: [w2269 T6."readBLE_HRM" T6."statusBLE_HRM" w2316] -> w2260
                tunnel: [w2268 FALSE FALSE w2313] -> w2259
                tunnel: w2258 -> [w2267 w2296 w2302 w2310]
                tunnel: [FALSE w2295 w2301 w2309] -> w2256
                tunnel: [w2265 w2295 w2301 w2308] -> w2255
                frame "verifyHand_Thumb", Default {
                  n1526 = global read "Global_usbComm.vi" "pulseType"() -> (w2262:string)
                  n1527 = Not Equal?(x=w2262, y="32") -> (x != y?=w2264:bool)
                  n1528 = case shown="False" w2264 {
                    tunnel: [T6."startBLE_HRM" w2281] -> w2269
                    tunnel: [FALSE w2280] -> w2268
                    tunnel: w2267 -> [w2275 w2279]
                    tunnel: [w2273 w2278] -> w2265
                    frame False {
                      w2273 = TRUE
                      n1529 = call "usbUart.vi"("VISA resource name"=w2275, "write buffer"="\u0002\u0001", "sdFeature"=FALSE) -> ("number[0]"=w2271:u32)  [unwired: 1 in, 15 out]
                      n1530 = local write "BLE Status"(w2271) -> ()
                      n1531 = local write "Hand/Thumb Pass"(w2273) -> ()
                      n1532 = local write "PUL1"(w2273) -> ()
                      n1533 = Wait (ms)(milliseconds to wait=u32 250) -> ()  [unwired: 1 out]
                    }
                    frame True {
                      n1534 = while {
                        tunnel: [w2292] -> w2281
                        tunnel: [w2283] -> w2280
                        tunnel: w2279 -> [w2287]
                        tunnel: [w2282] -> w2278
                        stop <- w2285 stop-if-true
                        w2291 = T6."startBLE_HRM"
                        n1535 = call "usbUart.vi"("VISA resource name"=w2287, "write buffer"="\u0002\u0001", "sdFeature"=FALSE) -> ("number[0]"=w2288:u32)  [unwired: 1 in, 15 out]
                        n1536 = local write "BLE Status"(w2288) -> ()
                        n1537 = Not(x="PUL0") -> (.not. x?=w2293:bool)
                        n1538 = Or(x="PUL0", y="PUL1") -> (x .or. y?=w2285:bool)
                        n1539 = Compound Arithmetic op=AND(TRUE ("value"), "PUL1", w2293) -> (w2282:bool)
                        "Hand/Thumb Pass" <- w2282
                        n1540 = Select(t=w2291, s=w2282, f=w2291) -> (s? t:f=w2292:T6)
                        n1541 = Not(x=w2282) -> (.not. x?=w2283:bool)
                      }
                    }
                  }
                }
                frame "startBLE_HRM" {
                  w2295 = FALSE ("Hand/Thumb Pass")
                  n1542 = call "usbCommand.vi"("write buffer"="\u000b\u0001", "VISA resource name in"=w2296) -> ()  [unwired: 8 in, 2 out]
                  n1543 = Wait (ms)(milliseconds to wait=u32 250) -> ()  [unwired: 1 out]
                }
                frame "readBLE_HRM" {
                  w2301 = FALSE ("Hand/Thumb Pass")
                  n1544 = call "usbUart.vi"("VISA resource name"=w2302, "write buffer"="F\u0001", "sdFeature"=FALSE) -> ("number[0]"=→"BLE_BPM" →"BLE PULSE":u32)  [unwired: 1 in, 15 out]
                }
                frame "statusBLE_HRM" {
                  n1545 = call "usbUart.vi"("VISA resource name"=w2310, "write buffer"="\u0002\u0001", "sdFeature"=FALSE) -> ("number[0]"=w2320:u32)  [unwired: 1 in, 15 out]
                  "BLE Status" <- w2320
                  n1546 = case shown="True" "E-stopHRM" {
                    selector: "E-stopHRM" -> [w2321 w2323]
                    tunnel: [w2321 w2323] -> w2311
                    tunnel: w2310 -> [_ w2322]
                    frame False {
                    }
                    frame True {
                      n1547 = call "usbCommand.vi"("write buffer"="\u000b\u0000", "VISA resource name in"=w2322) -> ()  [unwired: 8 in, 2 out]
                    }
                  }
                  n1548 = Equal?(x=u32 2, y=w2320) -> (x = y?=w2309:bool)
                  "BLE_HRM Pass" <- w2309
                  n1549 = Or(x=w2311, y=w2309) -> (x .or. y?=w2313:bool)
                  n1550 = Select(t=T6."statusBLE_HRM", s=w2309, f=T6."readBLE_HRM") -> (s? t:f=w2316:T6)
                  n1551 = local read "Hand/Thumb Pass"() -> (w2308:bool)
                }
              }
            }
            n1552 = Equal?(x=w2245, y=w2244) -> (x = y?=w2242:bool)
            n1553 = case shown="True" w2242 {
              selector: w2242 -> [w2325 w2331]
              tunnel: [w2326 w2332] -> w2250
              tunnel: w2246 -> [w2326 w2333]
              tunnel: [w2325 w2331] -> w2241
              frame False {
              }
              frame True {
                # "This is 1 second / per 10 samples"
                n1554 = while {
                  tunnel: [w2339] -> w2328 mode=indexing
                  i -> [w2337]
                  stop <- w2338 stop-if-true
                  n1555 = local read "EQF1259 com port"() -> (w2335:refnum<visa-resource-name>)
                  n1556 = Equal?(x=25, y=w2337) -> (x = y?=w2338:bool)
                  n1557 = call "currentScan.vi"("VISA resource name"=w2335) -> ("Ichart"=w2339:dbl)  [unwired: 7 in, 3 out]
                }
                n1558 = local read "refnum out"() -> (w2334:refnum<file>)
                n1559 = call-poly <vilib>:"Mean.vi"("X"=w2328) -> ("mean"=w2329:dbl)  [unwired: 1 out]
                n1560 = call "Pass_Fail.vi"("error in (no error)"=w2333, "OK"=w2331, "Byte Stream File in"=w2334) -> ("error out"=w2332:errorcluster)  [unwired: 7 in, 1 out]
                n1561 = Number To Fractional String(number=w2329, precision (6)=i16 2) -> (F-format string=w2330:string)  [unwired: 2 in]
                n1562 = global write "Global_usbComm.vi" "BaseCurrent"(w2330) -> ()
              }
            }
            n1563 = local read "EQF1259 com port"() -> (w2243:refnum<visa-resource-name>)
            n1564 = call "usbCommand.vi"("error in (no error)"=w2250, "write buffer"="'\u0000", "VISA resource name in"=w2243) -> ()  [unwired: 7 in, 2 out]
          }
        }
        n1565 = Select(t=T3."Fan" ("Tab Control"), s=w2234, f=T3."Failed" ("Tab Control")) -> (s? t:f=w2236:T3)
      }
      frame "Fan" {
        w2340 = "0.00" ("runCurrent")
        w2352 = FALSE
        n1566 = local write "FanCurrent"(0.0 ("CURRENT")) -> ()
        n1567 = local write "Ifan"(w2340) -> ()
        n1568 = property on="FanCurrent" class="WFChart (strict)"("History Data"=dbl[] []) -> ()  [unwired: 2 in, 2 out]
        n1569 = local write "FAN1"(w2352) -> ()
        n1570 = local write "FAN0"(w2352) -> ()
        n1571 = local write "fanIPeak"(w2340) -> ()
        n1572 = global write "Global_usbComm.vi" "runCurrent"(w2340) -> ()
        n1573 = local write "limitFan"(w2352) -> ()
        n1574 = flat-sequence {
          tunnel: [w2357] -> w2343
          tunnel: [w2364] -> w2345
          tunnel: [w2363] -> w2344
          tunnel: w2343 -> [w2363]
          tunnel: w2345 -> [w2374]
          tunnel: [w2374] -> w2347
          tunnel: [w2371] -> w2346
          tunnel: w2344 -> [w2369]
          tunnel: w2347 -> [w2377]
          tunnel: [w2378] -> w2349
          tunnel: [w2379] -> w2348
          tunnel: w2346 -> [w2379]
          frame #0 {
            n1575 = global read "Global_usbComm.vi" "FAN"() -> (w2359:string)
            "FAN" <- w2359
            n1576 = Not Equal?(x=w2359, y="0") -> (x != y?=w2357:bool)
          }
          frame #1 {
            # "% multiplier"
            n1577 = local read "EQF1259 com port"() -> (w2362:refnum<visa-resource-name>)
            n1578 = call "usbUart.vi"("VISA resource name"=w2362, "write buffer"="b\u0001", "sdFeature"=FALSE) -> ("byte[0]"=w2360:string, "error out"=w2364:errorcluster)  [unwired: 1 in, 14 out]
            n1579 = global write "Global_usbComm.vi" "fanType"(w2360) -> ()
            n1580 = case shown="\"01\", Default" w2360 {
              frame "01", Default {
                # "2-pin"
                n1581 = global write "Global_usbComm.vi" "tempNumeric"(0.25) -> ()
              }
              frame "02" {
                # "3-pin"
                n1582 = global write "Global_usbComm.vi" "tempNumeric"(0.6) -> ()
              }
              frame "04" {
                # "2 and 3-pin"
                n1583 = global write "Global_usbComm.vi" "tempNumeric"(0.7) -> ()
              }
            }
          }
          frame #2 {
            # "Verifies that config is correct"
            n1584 = global read "Global_usbComm.vi" "fanType"() -> (w2373:string)
            "fanType" <- w2373
            n1585 = Not Equal?(x=w2373, y="0") -> (x != y?=w2370:bool)
            n1586 = And(x=w2370, y=w2369) -> (x .and. y?=w2371:bool)
          }
          frame #3 {
            n1587 = global read "Global_usbComm.vi" "maxCurrent"() -> (w2376:string)
            "currentMaxFan" <- w2376
            n1588 = Fract/Exp String To Number(string=w2376) -> (number=w2375:dbl)  [unwired: 3 in, 1 out]
            n1589 = property on="FanCurrent" class="WFChart (strict)"(error in=w2377, "YScale.Maximum"=w2375) -> (error out=w2378:errorcluster)  [unwired: 1 in, 1 out]
          }
        }
        n1590 = case shown="True" w2348 {
          tunnel: [TRUE w2390] -> w2356
          tunnel: w2349 -> [w2380 w2388]
          frame False {
            n1591 = local read "refnum out"() -> (w2382:refnum<file>)
            n1592 = call "dataSampled.vi"("Error In"=w2380, "refnum in"=w2382) -> ()  [unwired: 8 in, 2 out]
          }
          frame True {
            n1593 = call "fanPIP.vi"() -> ("FAN-18"=→"FAN-18":string)  [unwired: 10 in, 1 out]
            n1594 = while {
              tunnel: [w2396] -> w2390
              tunnel: w2388 -> [w2395]
              tunnel: [w2394] -> w2387
              shift-right: [w2392] -> _
              shift-left: enum16{"High", "Low"}."High" -> [w2393]
              stop <- w2391 stop-if-true
              n1595 = case shown="\"High\", Default" w2393 {
                tunnel: [w2399 w2430] -> w2396
                tunnel: w2395 -> [_ w2429]
                tunnel: [w2398 w2426] -> w2394
                tunnel: [enum16{"High", "Low"}."Low" enum16{"High", "Low"}."Low"] -> w2392
                tunnel: [FALSE TRUE] -> w2391
                frame "High", Default {
                  n1596 = while {
                    tunnel: [w2413] -> w2399
                    shift-right: [w2403] -> _
                    shift-left: _ -> [w2410]
                    tunnel: [w2401] -> w2398
                    stop <- w2414 stop-if-true
                    n1597 = local read "EQF1259 com port"() -> (w2407:refnum<visa-resource-name>)
                    n1598 = local read "currentMaxFan"() -> (w2406:string)
                    n1599 = global read "Global_usbComm.vi" "PowerMode"() -> (w2409:string)
                    n1600 = local read "FAN0"() -> (w2405:bool)
                    n1601 = call "currentScan.vi"("Imax"=w2406, "VISA resource name"=w2407) -> ("max"=w2402:bool, "Istring"=w2403:string, "Ichart"=w2404:dbl)  [unwired: 6 in, 1 out]
                    n1602 = local write "FanCurrent"(w2404) -> ()
                    n1603 = local write "Ifan"(w2403) -> ()
                    n1604 = local write "limitFan"(w2402) -> ()
                    n1605 = case shown="\"On\"" w2409 {
                      tunnel: [FALSE w2423 w2425] -> w2408
                      tunnel: w2403 -> [_ w2422 _]
                      frame "Off", Default {
                        # "Why would I be Off"
                      }
                      frame "On" {
                        w2421 = 1.0 ("default (0 DBL)")
                        # "Lower limit control"
                        n1606 = global read "Global_usbComm.vi" "BaseCurrent"() -> (w2420:string)
                        n1607 = Fract/Exp String To Number(string=w2422, default (0 dbl)=w2421) -> (number=w2424:dbl)  [unwired: 2 in, 1 out]
                        n1608 = global read "Global_usbComm.vi" "tempNumeric"() -> (w2416:dbl)
                        n1609 = Fract/Exp String To Number(string=w2420, default (0 dbl)=w2421) -> (number=w2418:dbl)  [unwired: 2 in, 1 out]
                        n1610 = Multiply(x=w2418, y=w2416) -> (x*y=w2419:dbl)
                        n1611 = Add(x=w2418, y=w2419) -> (x+y=w2417:dbl)
                        n1612 = Greater Or Equal?(x=w2424, y=w2417) -> (x >= y?=w2423:bool)
                      }
                      frame "Battery" {
                        n1613 = local read "FAN1"() -> (w2425:bool)
                      }
                    }
                    n1614 = call "currentPeak.vi"("Istring# change"=w2410, "Istring# scan"=w2403) -> ("Ipeak"=w2401:string)  [unwired: 7 in, 2 out]
                    n1615 = Not(x=w2405) -> (.not. x?=w2412:bool)
                    n1616 = Not(x=w2402) -> (.not. x?=w2411:bool)
                    n1617 = local write "fanIPeak"(w2401) -> ()
                    n1618 = Compound Arithmetic op=OR(w2408, w2405, w2402) -> (w2414:bool)
                    n1619 = Compound Arithmetic op=AND(w2408, w2412, w2411) -> (w2413:bool)
                  }
                }
                frame "Low" {
                  n1620 = while {
                    tunnel: [w2439] -> w2430
                    tunnel: w2429 -> [_]
                    shift-right: [w2433] -> _
                    shift-left: _ -> [w2436]
                    tunnel: [w2431] -> w2426
                    stop <- w2444 stop-if-true
                    n1621 = local read "EQF1259 com port"() -> (w2442:refnum<visa-resource-name>)
                    n1622 = local read "currentMaxFan"() -> (w2441:string)
                    n1623 = global read "Global_usbComm.vi" "PowerMode"() -> (w2434:string)
                    n1624 = call "currentScan.vi"("Imax"=w2441, "VISA resource name"=w2442) -> ("max"=w2440:bool, "Istring"=w2433:string, "Ichart"=→"FanCurrent":dbl)  [unwired: 6 in, 1 out]
                    "Ifan" <- w2433
                    "limitFan" <- w2440
                    n1625 = case shown="\"On\"" w2434 {
                      tunnel: [FALSE w2453 "FAN1"] -> w2432
                      tunnel: w2433 -> [_ w2452 _]
                      frame "Off", Default {
                        # "Why would I be Off"
                      }
                      frame "On" {
                        w2451 = 1.0 ("default (0 DBL)")
                        # "Lower limit control"
                        n1626 = global read "Global_usbComm.vi" "BaseCurrent"() -> (w2450:string)
                        n1627 = Fract/Exp String To Number(string=w2450, default (0 dbl)=w2451) -> (number=w2447:dbl)  [unwired: 2 in, 1 out]
                        n1628 = Multiply(x=w2447, y=0.05) -> (x*y=w2448:dbl)
                        n1629 = Add(x=w2447, y=w2448) -> (x+y=w2446:dbl)
                        n1630 = Fract/Exp String To Number(string=w2452, default (0 dbl)=w2451) -> (number=w2454:dbl)  [unwired: 2 in, 1 out]
                        n1631 = Less Or Equal?(x=w2454, y=w2446) -> (x <= y?=w2453:bool)
                      }
                      frame "Battery" {
                      }
                    }
                    n1632 = Not(x=w2440) -> (.not. x?=w2437:bool)
                    n1633 = Not(x="FAN0") -> (.not. x?=w2438:bool)
                    n1634 = call "currentPeak.vi"("Istring# change"=w2436, "Istring# scan"=w2433) -> ("Ipeak"=w2431:string)  [unwired: 7 in, 2 out]
                    "fanIPeak" <- w2431
                    n1635 = Compound Arithmetic op=OR(w2432, "FAN0", w2440) -> (w2444:bool)
                    n1636 = Compound Arithmetic op=AND(w2432, w2438, w2437) -> (w2439:bool)
                    n1637 = local write "FAN1"(w2432) -> ()
                  }
                }
              }
            }
            n1638 = local read "refnum out"() -> (w2389:refnum<file>)
            n1639 = call "dataSampled.vi"("Data"=w2387, "refnum in"=w2389) -> ("error out"=w2384:errorcluster)  [unwired: 8 in, 1 out]
            n1640 = call "Wait.vi"("error in (no error)"=w2384, "milliseconds to wait"=u32 1500) -> ()  [unwired: 8 in, 2 out]
          }
        }
        n1641 = Select(t=T3."Audio" ("Tab Control"), s=w2356, f=T3."Failed" ("Tab Control")) -> (s? t:f=w2355:T3)
      }
      frame "Audio" {
        w2460 = "0.00" ("Ipeak")
        w2456 = FALSE
        # "All testing done with  tone \ngenerator set to:\n*80hz\n*full amplitude (dbm)\n*device at full volume\n\ntest tolerances...\nupper: .25\nlower: .075\n21\" tablet\n\nupper: .65\nlower: .075"
        n1642 = local write "limitAudio"(w2456) -> ()
        n1643 = local write "AUD1 2"(w2456) -> ()
        n1644 = local write "AUD0 2"(w2456) -> ()
        n1645 = local write "Iaudio"(w2460) -> ()
        n1646 = property on="AudioCurrent" class="WFChart (strict)"("History Data"=dbl[] []) -> ()  [unwired: 2 in, 2 out]
        n1647 = local write "AUD0"(w2456) -> ()
        n1648 = local write "audioIPeak"(w2460) -> ()
        n1649 = global write "Global_usbComm.vi" "runCurrent"(w2460) -> ()
        n1650 = local write "AUD1"(w2456) -> ()
        n1651 = flat-sequence {
          tunnel: [w2476] -> w2458
          tunnel: w2458 -> [w2478]
          tunnel: [w2478] -> w2457
          tunnel: [w2489] -> w2466
          tunnel: w2457 -> [w2489]
          frame #0 {
            n1652 = local read "EQF1259 com port"() -> (w2471:refnum<visa-resource-name>)
            n1653 = global read "Global_usbComm.vi" "maxCurrent"() -> (w2475:string)
            "currentMaxAudio" <- w2475
            n1654 = Fract/Exp String To Number(string=w2475) -> (number=w2468:dbl)  [unwired: 3 in, 1 out]
            n1655 = property on="AudioCurrent" class="WFChart (strict)"("YScale.Maximum"=w2468) -> ()  [unwired: 2 in, 2 out]
            n1656 = call "usbUart.vi"("VISA resource name"=w2471, "write buffer"="`\u0002", "sdFeature"=FALSE) -> ("number[0]"=w2473:u32)  [unwired: 1 in, 15 out]
            n1657 = Number To Decimal String(number=w2473) -> (decimal integer string=w2469:string)  [unwired: 1 in]
            n1658 = global write "Global_usbComm.vi" "audioType"(w2469) -> ()
            n1659 = Not Equal?(x=w2469, y="1") -> (x != y?=w2476:bool)
          }
          frame #1 {
            # "Wait for current to \nreturn to run state"
            n1660 = call "audio_tvPIP.vi"() -> ("AUDIO-19"=→"AUDIO-19":string)  [unwired: 9 in, 2 out]
            n1661 = while {
              shift-right: [w2487] -> _
              shift-left: _ -> [w2485]
              stop <- w2484 stop-if-true
              n1662 = Fract/Exp String To Number(string=w2485) -> (number=w2483:dbl)  [unwired: 3 in, 1 out]
              n1663 = global read "Global_usbComm.vi" "BaseCurrent"() -> (w2486:string)
              n1664 = Fract/Exp String To Number(string=w2486) -> (number=w2482:dbl)  [unwired: 3 in, 1 out]
              n1665 = global read "Global_usbComm.vi" "maxCurrent"() -> (w2479:string)
              n1666 = local read "EQF1259 com port"() -> (w2488:refnum<visa-resource-name>)
              n1667 = Multiply(x=1.01, y=w2482) -> (x*y=w2481:dbl)
              n1668 = In Range and Coerce(upper limit=w2481, x=w2483, lower limit=w2482) -> (In Range?=w2484:bool)  [unwired: 1 out]
              n1669 = call "currentScan.vi"("Imax"=w2479, "VISA resource name"=w2488) -> ("Istring"=w2487:string)  [unwired: 6 in, 3 out]
            }
          }
          frame #2 {
            # "BLE Audio connect"
            n1670 = flat-sequence {
              tunnel: [w2491] -> w2490
              tunnel: w2490 -> [w2501]
              tunnel: w2489 -> [w2500]
              frame #0 {
                n1671 = while {
                  tunnel: [w2495] -> w2491
                  i -> [w2493]
                  stop <- w2496 stop-if-true
                  n1672 = global read "Global_usbComm.vi" "audioType"() -> (w2497:string)
                  n1673 = Index Array(array=string[] ["68", "100", "228"], index=w2493) -> (element=w2498:string)
                  n1674 = Equal?(x=w2498, y=w2497) -> (x = y?=w2495:bool)
                  n1675 = Equal?(x=3, y=w2493) -> (x = y?=w2494:bool)
                  n1676 = Or(x=w2495, y=w2494) -> (x .or. y?=w2496:bool)
                }
              }
              frame #1 {
                n1677 = And(x=w2501, y=w2500) -> (x .and. y?=w2502:bool)
                n1678 = case shown="True" w2502 {
                  frame False {
                    # "No BLE Audio feature"
                    n1679 = local write "AUD1 2"(TRUE ("AUD1 2")) -> ()
                  }
                  frame True {
                    n1680 = while {
                      tunnel: [w2505] -> w2504
                      stop <- w2508 stop-if-true
                      n1681 = Not(x="AUD0 2") -> (.not. x?=w2509:bool)
                      n1682 = Or(x="AUD1 2", y="AUD0 2") -> (x .or. y?=w2508:bool)
                      n1683 = Compound Arithmetic op=AND(TRUE ("value"), "AUD1 2", w2509) -> (w2507:bool)
                      n1684 = Not(x=w2507) -> (.not. x?=w2505:bool)
                    }
                    n1685 = local write "AUD0"(w2504) -> ()
                  }
                }
              }
            }
          }
        }
        n1686 = case shown="True" w2466 {
          tunnel: [TRUE w2519] -> w2459
          frame False {
            n1687 = local read "refnum out"() -> (w2512:refnum<file>)
            n1688 = call "dataSampled.vi"("refnum in"=w2512) -> ()  [unwired: 9 in, 2 out]
          }
          frame True {
            # "if (!Battery)\n{\n   current();\n}\nelse\n{\n   manual();\n}"
            n1689 = global read "Global_usbComm.vi" "PowerMode"() -> (w2515:string)
            n1690 = Not Equal?(x=w2515, y="Battery") -> (x != y?=w2516:bool)
            n1691 = case shown="True" w2516 {
              tunnel: ["Battery" ("Ipeak") w2531] -> w2520
              tunnel: [w2522 w2530] -> w2519
              frame False {
                n1692 = while {
                  tunnel: [w2524] -> w2522
                  stop <- w2529 stop-if-true
                  n1693 = local read "AUD1"() -> (w2526:bool)
                  n1694 = local read "AUD0"() -> (w2528:bool)
                  n1695 = Not(x=w2528) -> (.not. x?=w2527:bool)
                  n1696 = Or(x=w2526, y=w2528) -> (x .or. y?=w2529:bool)
                  n1697 = Compound Arithmetic op=AND(TRUE ("value"), w2526, w2527) -> (w2524:bool)
                }
              }
              frame True {
                n1698 = while {
                  tunnel: [w2537] -> w2530
                  tunnel: [w2536] -> w2531
                  shift-right: [w2534] -> _
                  shift-left: enum16{"High", "Low"}."High" -> [w2535]
                  stop <- w2533 stop-if-true
                  n1699 = case shown="\"High\", Default" w2535 {
                    tunnel: [w2540 w2572] -> w2537
                    tunnel: [w2539 w2569] -> w2536
                    tunnel: [enum16{"High", "Low"}."Low" enum16{"High", "Low"}."Low"] -> w2534
                    tunnel: [FALSE TRUE] -> w2533
                    frame "High", Default {
                      n1700 = while {
                        tunnel: [w2556] -> w2540
                        shift-right: [w2548] -> _
                        shift-left: _ -> [w2553]
                        tunnel: [w2546] -> w2539
                        stop <- w2557 stop-if-true
                        n1701 = local read "EQF1259 com port"() -> (w2544:refnum<visa-resource-name>)
                        n1702 = local read "currentMaxAudio"() -> (w2545:string)
                        n1703 = global read "Global_usbComm.vi" "PowerMode"() -> (w2552:string)
                        n1704 = local read "AUD0"() -> (w2550:bool)
                        n1705 = call "currentScan.vi"("Imax"=w2545, "VISA resource name"=w2544) -> ("error out"=w2542:errorcluster, "max"=w2547:bool, "Istring"=w2548:string, "Ichart"=w2549:dbl)  [unwired: 6 in]
                        n1706 = local write "AudioCurrent"(w2549) -> ()
                        n1707 = local write "Ifan"(w2548) -> ()
                        n1708 = case shown="\"On\"" w2552 {
                          tunnel: [FALSE w2566 w2568] -> w2551
                          tunnel: w2548 -> [_ w2565 _]
                          frame "Off", Default {
                            # "Why would I be Off"
                          }
                          frame "On" {
                            w2564 = 1.0 ("default (0 DBL)")
                            # "Lower limit control"
                            n1709 = global read "Global_usbComm.vi" "BaseCurrent"() -> (w2563:string)
                            n1710 = Fract/Exp String To Number(string=w2563, default (0 dbl)=w2564) -> (number=w2560:dbl)  [unwired: 2 in, 1 out]
                            n1711 = Multiply(x=w2560, y=0.1) -> (x*y=w2561:dbl)
                            n1712 = Add(x=w2560, y=w2561) -> (x+y=w2559:dbl)
                            n1713 = Fract/Exp String To Number(string=w2565, default (0 dbl)=w2564) -> (number=w2567:dbl)  [unwired: 2 in, 1 out]
                            n1714 = Greater Or Equal?(x=w2567, y=w2559) -> (x >= y?=w2566:bool)
                          }
                          frame "Battery" {
                            n1715 = local read "AUD1"() -> (w2568:bool)
                          }
                        }
                        n1716 = local write "limitAudio"(w2547) -> ()
                        n1717 = Not(x=w2550) -> (.not. x?=w2555:bool)
                        n1718 = Not(x=w2547) -> (.not. x?=w2554:bool)
                        n1719 = call "currentPeak.vi"("error in (no error)"=w2542, "Istring# change"=w2553, "Istring# scan"=w2548) -> ("Ipeak"=w2546:string, "Irun"=w2543:string)  [unwired: 6 in, 1 out]
                        n1720 = local write "Iaudio"(w2543) -> ()
                        n1721 = local write "audioIPeak"(w2546) -> ()
                        n1722 = Compound Arithmetic op=OR(w2551, w2550, w2547) -> (w2557:bool)
                        n1723 = Compound Arithmetic op=AND(w2551, w2555, w2554) -> (w2556:bool)
                      }
                    }
                    frame "Low" {
                      n1724 = while {
                        tunnel: [w2585] -> w2572
                        shift-right: [w2580] -> _
                        shift-left: _ -> [w2582]
                        tunnel: [w2573] -> w2569
                        stop <- w2587 stop-if-true
                        n1725 = local read "EQF1259 com port"() -> (w2578:refnum<visa-resource-name>)
                        n1726 = local read "currentMaxAudio"() -> (w2577:string)
                        n1727 = global read "Global_usbComm.vi" "PowerMode"() -> (w2581:string)
                        n1728 = call "currentScan.vi"("Imax"=w2577, "VISA resource name"=w2578) -> ("max"=w2586:bool, "Istring"=w2580:string, "Ichart"=→"AudioCurrent":dbl)  [unwired: 6 in, 1 out]
                        "limitAudio" <- w2586
                        n1729 = case shown="\"On\"" w2581 {
                          tunnel: [FALSE w2596 "AUD1"] -> w2574
                          tunnel: w2580 -> [_ w2595 _]
                          frame "Off", Default {
                            # "Why would I be Off"
                          }
                          frame "On" {
                            w2594 = 1.0 ("default (0 DBL)")
                            # "Lower limit control"
                            n1730 = global read "Global_usbComm.vi" "BaseCurrent"() -> (w2593:string)
                            n1731 = Fract/Exp String To Number(string=w2593, default (0 dbl)=w2594) -> (number=w2590:dbl)  [unwired: 2 in, 1 out]
                            n1732 = Multiply(x=w2590, y=0.075) -> (x*y=w2591:dbl)
                            n1733 = Add(x=w2590, y=w2591) -> (x+y=w2589:dbl)
                            n1734 = Fract/Exp String To Number(string=w2595, default (0 dbl)=w2594) -> (number=w2597:dbl)  [unwired: 2 in, 1 out]
                            n1735 = Less Or Equal?(x=w2597, y=w2589) -> (x <= y?=w2596:bool)
                          }
                          frame "Battery" {
                          }
                        }
                        n1736 = Not(x=w2586) -> (.not. x?=w2583:bool)
                        n1737 = Not(x="AUD0") -> (.not. x?=w2584:bool)
                        n1738 = call "currentPeak.vi"("Istring# change"=w2582, "Istring# scan"=w2580) -> ("Ipeak"=w2573:string, "Irun"=→"Iaudio":string)  [unwired: 7 in, 1 out]
                        "audioIPeak" <- w2573
                        n1739 = Compound Arithmetic op=OR(w2574, "AUD0", w2586) -> (w2587:bool)
                        n1740 = Compound Arithmetic op=AND(w2574, w2584, w2583) -> (w2585:bool)
                        n1741 = local write "AUD1"(w2574) -> ()
                      }
                    }
                  }
                }
              }
            }
            n1742 = local read "refnum out"() -> (w2521:refnum<file>)
            n1743 = call "dataSampled.vi"("Data"=w2520, "refnum in"=w2521) -> ("error out"=w2518:errorcluster)  [unwired: 8 in, 1 out]
            n1744 = call "Wait.vi"("error in (no error)"=w2518, "milliseconds to wait"=u32 1500) -> ()  [unwired: 8 in, 2 out]
          }
        }
        n1745 = Select(t=T3."TV" ("Tab Control"), s=w2459, f=T3."Failed" ("Tab Control")) -> (s? t:f=w2467:T3)
      }
      frame "TV" {
        w2599 = "0.00" ("USB")
        w2607 = FALSE
        n1746 = local write "Itv"(w2599) -> ()
        n1747 = local write "TV1"(w2607) -> ()
        n1748 = local write "TV0"(w2607) -> ()
        n1749 = property on="TVCurrent" class="WFChart (strict)"("History Data"=dbl[] []) -> ()  [unwired: 2 in, 2 out]
        n1750 = local write "tvIPeak"(w2599) -> ()
        n1751 = global write "Global_usbComm.vi" "runCurrent"(w2599) -> ()
        n1752 = local write "limitTV"(w2607) -> ()
        n1753 = while {
          shift-right: [w2612] -> _
          shift-left: 0 -> [w2613]
          tunnel: [w2611] -> w2602
          stop <- w2610 stop-if-true
          n1754 = case shown="0, Default" w2613 {
            tunnel: [1 _] -> w2612
            tunnel: [FALSE w2623] -> w2611
            tunnel: [FALSE TRUE] -> w2610
            frame 0, Default {
              n1755 = global read "Global_usbComm.vi" "maxCurrent"() -> (w2615:string)
              "currentMaxTV" <- w2615
              n1756 = Fract/Exp String To Number(string=w2615) -> (number=w2614:dbl)  [unwired: 3 in, 1 out]
              n1757 = property on="TVCurrent" class="WFChart (strict)"("YScale.Maximum"=w2614) -> ()  [unwired: 2 in, 2 out]
            }
            frame 1 {
              w2626 = 128
              n1758 = global read "Global_usbComm.vi" "audioType"() -> (w2629:string)
              n1759 = global read "Global_usbComm.vi" "TV"() -> (w2619:string)
              n1760 = Decimal String To Number(string=w2629) -> (number=w2627:i32)  [unwired: 2 in, 1 out]
              n1761 = Decimal String To Number(string=w2619) -> (number=w2628:i32)  [unwired: 2 in, 1 out]
              n1762 = global read "Global_usbComm.vi" "tabletType"() -> (w2620:string)
              n1763 = Greater Or Equal?(x=w2628, y=w2626) -> (x >= y?=w2631:bool)
              n1764 = Greater Or Equal?(x=w2627, y=w2626) -> (x >= y?=w2630:bool)
              n1765 = Compound Arithmetic op=OR(w2631, w2630) -> (w2625:bool)
              n1766 = Equal?(x="1", y=w2620) -> (x = y?=w2621:bool)
              n1767 = Or(x=w2621, y=w2625) -> (x .or. y?=w2623:bool)
            }
          }
        }
        n1768 = case shown="True" w2602 {
          tunnel: [TRUE w2636] -> w2609
          frame False {
            n1769 = local read "refnum out"() -> (w2632:refnum<file>)
            n1770 = call "dataSampled.vi"("refnum in"=w2632) -> ()  [unwired: 9 in, 2 out]
          }
          frame True {
            n1771 = while {
              tunnel: [w2654] -> w2636
              shift-right: [w2642] -> _
              shift-left: _ -> [w2640]
              tunnel: [w2641] -> w2634
              stop <- w2655 stop-if-true
              n1772 = global read "Global_usbComm.vi" "tabletType"() -> (w2639:string)
              n1773 = Equal?(x=w2639, y="1") -> (x = y?=w2645:bool)
              n1774 = case shown="True" w2645 {
                tunnel: [w2657 w2659] -> w2647
                tunnel: [w2656 _] -> w2644
                frame False {
                  n1775 = call "audio_tvPIP.vi"() -> ("error out"=w2656:errorcluster, "TV-20"=w2657:string)  [unwired: 9 in, 1 out]
                }
                frame True {
                  n1776 = global read "Global_usbComm.vi" "PIP_Instruction"() -> (w2658:string[][])
                  n1777 = Index Array(array=w2658, index (row)=1 ("disabled index (row)"), index (col)=20 ("disabled index (col)")) -> (element=w2659:string)
                }
              }
              "TV-20" <- w2647
              n1778 = local read "EQF1259 com port"() -> (w2651:refnum<visa-resource-name>)
              n1779 = local read "currentMaxTV"() -> (w2650:string)
              n1780 = call "currentScan.vi"("error in (no error)"=w2644, "Imax"=w2650, "VISA resource name"=w2651) -> ("max"=w2648:bool, "Istring"=w2642:string, "Ichart"=→"TVCurrent":dbl)  [unwired: 5 in, 1 out]
              "limitTV" <- w2648
              n1781 = Compound Arithmetic op=OR("TV0", "TV1", w2648) -> (w2655:bool)
              n1782 = Not(x="TV0") -> (.not. x?=w2643:bool)
              n1783 = Not(x=w2648) -> (.not. x?=w2649:bool)
              n1784 = call "currentPeak.vi"("Istring# change"=w2640, "Istring# scan"=w2642) -> ("Ipeak"=w2641:string, "Irun"=→"Itv":string)  [unwired: 7 in, 1 out]
              "tvIPeak" <- w2641
              n1785 = Compound Arithmetic op=AND(w2643, "TV1", w2649) -> (w2654:bool)
            }
            n1786 = local read "refnum out"() -> (w2635:refnum<file>)
            n1787 = call "dataSampled.vi"("Data"=w2634, "refnum in"=w2635) -> ()  [unwired: 8 in, 2 out]
          }
        }
        n1788 = Select(t=T3."USB" ("Tab Control"), s=w2609, f=T3."Failed" ("Tab Control")) -> (s? t:f=w2608:T3)
      }
      frame "USB" {
        w2662 = "0.00" ("USB")
        w2668 = FALSE
        n1789 = local write "FanCurrent"(0.0 ("CURRENT")) -> ()
        n1790 = local write "Iusb"(w2662) -> ()
        n1791 = property on="USBCurrent" class="WFChart (strict)"("History Data"=dbl[] []) -> ()  [unwired: 2 in, 2 out]
        n1792 = local write "USB0"(w2668) -> ()
        n1793 = local write "USB1"(w2668) -> ()
        n1794 = local write "usbIPeak"(w2662) -> ()
        n1795 = global write "Global_usbComm.vi" "runCurrent"(w2662) -> ()
        n1796 = local write "limitUSB"(w2668) -> ()
        n1797 = flat-sequence {
          tunnel: [w2680] -> w2667
          frame #0 {
            n1798 = global read "Global_usbComm.vi" "maxCurrent"() -> (w2673:string)
            "currentMaxUSB" <- w2673
            n1799 = local read "EQF1259 com port"() -> (w2674:refnum<visa-resource-name>)
            n1800 = Fract/Exp String To Number(string=w2673) -> (number=w2672:dbl)  [unwired: 3 in, 1 out]
            n1801 = property on="USBCurrent" class="WFChart (strict)"("YScale.Maximum"=w2672) -> ()  [unwired: 2 in, 2 out]
            n1802 = call "usbUart.vi"("VISA resource name"=w2674, "write buffer"="c\u0001") -> ("number[0]"=w2676:u32)  [unwired: 2 in, 15 out]
            n1803 = Number To Decimal String(number=w2676) -> (decimal integer string=w2677:string)  [unwired: 1 in]
            n1804 = global write "Global_usbComm.vi" "usbType"(w2677) -> ()
          }
          frame #1 {
            n1805 = call "usbPIP.vi"() -> ("Boolean"=w2679:bool, "USB-16"=→"USB-16":string)  [unwired: 9 in, 1 out]
            n1806 = case shown="True" w2679 {
              tunnel: [TRUE w2685] -> w2680
              frame False {
                n1807 = local read "refnum out"() -> (w2681:refnum<file>)
                n1808 = call "dataSampled.vi"("refnum in"=w2681) -> ()  [unwired: 9 in, 2 out]
              }
              frame True {
                n1809 = while {
                  tunnel: [w2695] -> w2685
                  shift-right: [w2688] -> _
                  shift-left: _ -> [w2687]
                  tunnel: [w2686] -> w2683
                  stop <- w2698 stop-if-true
                  n1810 = local read "EQF1259 com port"() -> (w2693:refnum<visa-resource-name>)
                  n1811 = local read "currentMaxUSB"() -> (w2692:string)
                  n1812 = call "currentScan.vi"("Imax"=w2692, "VISA resource name"=w2693) -> ("max"=w2689:bool, "Istring"=w2688:string, "Ichart"=→"USBCurrent":dbl)  [unwired: 6 in, 1 out]
                  "limitUSB" <- w2689
                  n1813 = Compound Arithmetic op=OR("USB0", "USB1", w2689) -> (w2698:bool)
                  n1814 = Not(x="USB1") -> (.not. x?=w2699:bool)
                  n1815 = Not(x=w2689) -> (.not. x?=w2694:bool)
                  n1816 = call "currentPeak.vi"("Istring# change"=w2687, "Istring# scan"=w2688) -> ("Ipeak"=w2686:string, "Irun"=→"Iusb":string)  [unwired: 7 in, 1 out]
                  "usbIPeak" <- w2686
                  n1817 = Compound Arithmetic op=AND("USB0", w2699, w2694) -> (w2695:bool)
                }
                n1818 = local read "refnum out"() -> (w2684:refnum<file>)
                n1819 = call "dataSampled.vi"("Data"=w2683, "refnum in"=w2684) -> ()  [unwired: 8 in, 2 out]
              }
            }
          }
        }
        n1820 = Select(t=T3."Resistance" ("Tab Control"), s=w2667, f=T3."Failed" ("Tab Control")) -> (s? t:f=w2670:T3)
      }
      frame "CSafe" {
        w2707 = "0.00" ("runCurrent")
        w2713 = FALSE
        n1821 = local write "FanCurrent"(0.0 ("CURRENT")) -> ()
        n1822 = property on="CSafeCurrent" class="WFChart (strict)"("History Data"=dbl[] []) -> ()  [unwired: 2 in, 2 out]
        n1823 = local write "Icsafe"(w2707) -> ()
        n1824 = local write "CSA0"(w2713) -> ()
        n1825 = local write "CSA1"(w2713) -> ()
        n1826 = local read "EQF1259 com port"() -> (w2708:refnum<visa-resource-name>)
        n1827 = local write "csafeIPeak"(w2707) -> ()
        n1828 = global write "Global_usbComm.vi" "runCurrent"(w2707) -> ()
        n1829 = local write "limitCSafe"(w2713) -> ()
        n1830 = call "currentMax.vi"("VISA Refnum in"=w2708) -> ("stringCurrentMax"=→"currentMaxCSafe":string, "numberCurrentMax"=w2710:dbl)  [unwired: 8 in, 1 out]
        n1831 = property on="CSafeCurrent" class="WFChart (strict)"("YScale.Maximum"=w2710) -> ()  [unwired: 2 in, 2 out]
        n1832 = global read "Global_usbComm.vi" "CSAFE"() -> (w2712:string)
        n1833 = Not Equal?(x=w2712, y="0") -> (x != y?=w2716:bool)
        n1834 = case shown="False" w2716 {
          tunnel: [TRUE w2726] -> w2719
          frame False {
            n1835 = local read "refnum out"() -> (w2721:refnum<file>)
            n1836 = Write to Text File(file (use dialog)=w2721, text="NULL" ("Data")) -> ()  [unwired: 2 in, 3 out]
          }
          frame True {
            n1837 = call "csafePIP.vi"() -> ("CSAFE-21"=→"CSAFE-21":string)  [unwired: 10 in, 1 out]
            n1838 = while {
              tunnel: [w2737] -> w2726
              shift-right: [w2732] -> _
              shift-left: _ -> [w2730]
              tunnel: [w2729] -> w2723
              stop <- w2740 stop-if-true
              n1839 = local read "EQF1259 com port"() -> (w2735:refnum<visa-resource-name>)
              n1840 = local read "currentMaxCSafe"() -> (w2734:string)
              n1841 = call "currentScan.vi"("Imax"=w2734, "VISA resource name"=w2735) -> ("error out"=w2733:errorcluster, "max"=w2731:bool, "Istring"=w2728:string, "Ichart"=→"CSafeCurrent":dbl)  [unwired: 6 in]
              "limitCSafe" <- w2731
              "Icsafe" <- w2728
              n1842 = Not(x="CSA1") -> (.not. x?=w2741:bool)
              n1843 = Not(x=w2731) -> (.not. x?=w2727:bool)
              n1844 = call "currentPeak.vi"("error in (no error)"=w2733, "Istring# change"=w2730, "Istring# scan"=w2728) -> ("Ipeak"=w2729:string, "Irun"=w2732:string)  [unwired: 6 in, 1 out]
              "csafeIPeak" <- w2729
              n1845 = Compound Arithmetic op=OR("CSA0", "CSA1", w2731) -> (w2740:bool)
              n1846 = Compound Arithmetic op=AND("CSA0", w2741, w2727) -> (w2737:bool)
            }
            n1847 = local read "refnum out"() -> (w2725:refnum<file>)
            n1848 = Write to Text File(file (use dialog)=w2725, text=w2723) -> ()  [unwired: 2 in, 3 out]
          }
        }
        n1849 = Greater?(x=w2704, y=1) -> (0:w2705:bool)
        n1850 = Select(t=T1."Another" ("Tab Control"), s=w2705, f=T1."Finish" ("Tab Control")) -> (s? t:f=w2701:T1)
        n1851 = Select(t=w2701, s=w2719, f=T1."Failed" ("Tab Control")) -> (s? t:f=w2715:T1)
      }
      frame "Wahoo" {
        w2744 = "0.00" ("runCurrent")
        w2752 = FALSE
        # "This is tested as a BLE connection and HRM test"
        n1852 = local write "FanCurrent"(0.0 ("CURRENT")) -> ()
        n1853 = global write "Global_usbComm.vi" "runCurrent"(w2744) -> ()
        n1854 = local write "Iwahoo"(w2744) -> ()
        n1855 = local write "wahooIPeak"(w2744) -> ()
        n1856 = property on="WahooCurrent" class="WFChart (strict)"("History Data"=dbl[] []) -> ()  [unwired: 2 in, 2 out]
        n1857 = local write "WAH0"(w2752) -> ()
        n1858 = local write "WAH1"(w2752) -> ()
        n1859 = local read "EQF1259 com port"() -> (w2747:refnum<visa-resource-name>)
        n1860 = local write "limitWahoo"(w2752) -> ()
        n1861 = call "currentMax.vi"("VISA Refnum in"=w2747) -> ("stringCurrentMax"=→"currentMaxWahoo":string, "numberCurrentMax"=w2746:dbl)  [unwired: 8 in, 1 out]
        n1862 = property on="WahooCurrent" class="WFChart (strict)"("YScale.Maximum"=w2746) -> ()  [unwired: 2 in, 2 out]
        n1863 = global read "Global_usbComm.vi" "WAHOO"() -> (w2751:string)
        n1864 = Not Equal?(x=w2751, y="0" ("WAHOO")) -> (x != y?=w2754:bool)
        n1865 = case shown="True" w2754 {
          tunnel: [TRUE w2763] -> w2750
          frame False {
            n1866 = local read "refnum out"() -> (w2758:refnum<file>)
            n1867 = call "dataSampled.vi"("refnum in"=w2758) -> ()  [unwired: 9 in, 2 out]
          }
          frame True {
            n1868 = call "wahooPIP.vi"() -> ("WAHOO-22"=→"WAHOO-22":string)  [unwired: 10 in, 1 out]
            n1869 = while {
              tunnel: [w2774] -> w2763
              tunnel: [w2768] -> w2760
              shift-right: [w2767] -> _
              shift-left: _ -> [w2766]
              stop <- w2777 stop-if-true
              n1870 = local read "currentMaxWahoo"() -> (w2772:string)
              n1871 = local read "EQF1259 com port"() -> (w2771:refnum<visa-resource-name>)
              n1872 = call "currentScan.vi"("Imax"=w2772, "VISA resource name"=w2771) -> ("error out"=w2773:errorcluster, "max"=w2769:bool, "Istring"=w2765:string, "Ichart"=→"WahooCurrent":dbl)  [unwired: 6 in]
              "Iwahoo" <- w2765
              "limitWahoo" <- w2769
              n1873 = Not(x="WAH1") -> (.not. x?=w2778:bool)
              n1874 = Not(x=w2769) -> (.not. x?=w2764:bool)
              n1875 = Compound Arithmetic op=OR("WAH0", "WAH1", w2769) -> (w2777:bool)
              n1876 = call "currentPeak.vi"("error in (no error)"=w2773, "Istring# change"=w2766, "Istring# scan"=w2765) -> ("Ipeak"=w2768:string, "Irun"=w2767:string)  [unwired: 6 in, 1 out]
              "wahooIPeak" <- w2768
              n1877 = Compound Arithmetic op=AND("WAH0", w2778, w2764) -> (w2774:bool)
            }
            n1878 = local read "refnum out"() -> (w2762:refnum<file>)
            n1879 = call "dataSampled.vi"("Data"=w2760, "refnum in"=w2762) -> ()  [unwired: 8 in, 2 out]
          }
        }
        n1880 = Select(t=T1."Finish" ("Tab Control"), s=w2750, f=T1."Failed" ("Tab Control")) -> (s? t:f=w2756:T1)
      }
      frame "Another" {
        w2792 = FALSE
        n1881 = Subtract(x=w2784, y=w2783) -> (x-y=→"# of Passed Samples":i32)
        n1882 = local write "ANO0"(w2792) -> ()
        n1883 = local write "ANO1"(w2792) -> ()
        n1884 = global read "Global_usbComm.vi" "PIC_ARRAY"() -> (w2787:picture[])
        n1885 = local read "refnum out"() -> (w2791:refnum<file>)
        n1886 = Index Array(array=w2787, index=3) -> (element=→"Another":picture)
        n1887 = Write to Text File(file (use dialog)=w2791, text="\r") -> ()  [unwired: 2 in, 3 out]
        n1888 = local read "EQF1259 com port"() -> (w2780:refnum<visa-resource-name>)
        n1889 = call "usbCommand.vi"("write buffer"="\u0005\u0004", "VISA resource name in"=w2780) -> ("error out"=w2779:errorcluster)  [unwired: 8 in, 1 out]
        n1890 = while {
          tunnel: [w2795] -> w2794
          tunnel: w2779 -> [_]
          stop <- w2798 stop-if-true
          n1891 = Not(x="ANO0") -> (.not. x?=w2799:bool)
          n1892 = Compound Arithmetic op=OR("ANO1", "ANO0") -> (w2798:bool)
          n1893 = Compound Arithmetic op=AND("ANO1", w2799) -> (w2795:bool)
        }
        n1894 = Select(t=T3."Scan DUT" ("Tab Control"), s=w2794, f=T3."end" ("Tab Control")) -> (s? t:f=w2793:T3)
      }
      frame "Failed" {
        n1895 = call "Display Message to User6"() -> ()  [unwired: 10 in, 2 out]
        n1896 = Increment(x=w2807) -> (x+1=w2806:i32)
        "# of Failed Samples" <- w2806
        n1897 = global read "Global_usbComm.vi" "PIC_ARRAY"() -> (w2802:picture[])
        n1898 = local read "refnum out"() -> (w2811:refnum<file>)
        n1899 = local read "EQF1259 com port"() -> (w2808:refnum<visa-resource-name>)
        n1900 = Index Array(array=w2802, index=4) -> (element=→"Failed":picture)
        n1901 = call "dataSampled.vi"("Data"="FAILED" ("string"), "refnum in"=w2811) -> ()  [unwired: 8 in, 2 out]
        n1902 = call "usbUart.vi"("VISA resource name"=w2808, "write buffer"="(\u0001", "sdFeature"=FALSE) -> ()  [unwired: 1 in, 16 out]
      }
      frame "end" {
        n1903 = while {
          shift-right: [w2817] -> _
          shift-left: 0 -> [w2819]
          stop <- w2818 stop-if-true
          n1904 = case shown="2" w2819 {
            tunnel: [FALSE _ _ TRUE] -> w2818
            tunnel: [1 2 3 _] -> w2817
            frame 0, Default {
              n1905 = global read "Global_usbComm.vi" "PIC_ARRAY"() -> (w2825:picture[])
              n1906 = Index Array(array=w2825, index=0) -> (element=→"Goodbye!":picture)
              n1907 = local write "Test Log"("") -> ()
            }
            frame 1 {
              n1908 = local read "refnum out"() -> (w2830:refnum<file>)
              n1909 = call "Close Data File and open.vi"("File Refnum In"=w2830) -> ("path"=w2829:path)  [unwired: 9 in, 1 out]
              n1910 = Path To String(path=w2829) -> (string=→"Test Log":string)
              n1911 = Wait (ms)(milliseconds to wait=u32 250) -> ()  [unwired: 1 out]
            }
            frame 2 {
              w2834 = "\""
              n1912 = Wait (ms)(milliseconds to wait=u32 250) -> ()  [unwired: 1 out]
              n1913 = local read "Test Log"() -> (w2833:string)
              n1914 = call <vilib>:"Space Constant.vi"() -> ("String"=w2839:string)
              n1915 = Concatenate Strings("cmd /c C:\\specsheetsConsole\\build\\exe.win-amd64-3.6\\labviewdbupload.exe ", w2839, w2834, w2833, w2834) -> (w2832:string)
              n1916 = call "exeCLI.vi"("Tab Control"=T2."Built-in command line utilities", "command line (built-in)"=w2832) -> ("standard error"=→"standard notepad":string)  [unwired: 11 in, 2 out]
            }
            frame 3 {
              w2841 = "\""
              n1917 = local read "Test Log"() -> (w2842:string)
              n1918 = call <vilib>:"Space Constant.vi"() -> ("String"=w2846:string)
              n1919 = Concatenate Strings("C:\\Windows\\System32\\notepad.exe" ("Command"), w2846, w2841, w2842, w2841) -> (w2847:string)
              n1920 = call "exeCLI.vi"("Tab Control"=T2."Interactive applications", "command line (interactive)"=w2847) -> ("standard error"=→"standard labviewdbupload":string)  [unwired: 11 in, 2 out]
            }
          }
        }
      }
      frame "Finish" {
        n1921 = local write "FIN0"(FALSE ("FIN0")) -> ()
        n1922 = local read "EQF1259 com port"() -> (w2851:refnum<visa-resource-name>)
        n1923 = call "usbUart.vi"("VISA resource name"=w2851, "write buffer"="Y\u0001", "sdFeature"=FALSE) -> ("number[0]"=w2852:u32)  [unwired: 1 in, 15 out]
        n1924 = case shown="4" w2852 {
          tunnel: [_ w2860 w2861 w2865 w2869] -> w2849
          frame 0, Default {
          }
          frame 1 {
            n1925 = global read "Global_usbComm.vi" "PIP_Instruction"() -> (w2859:string[][])
            n1926 = Index Array(array=w2859, index (row)=1, index (col)=25 ("disabled index (col)")) -> (element=w2860:string)
            n1927 = global write "Global_usbComm.vi" "FINISH-25"(w2860) -> ()
          }
          frame 2 {
            n1928 = global read "Global_usbComm.vi" "PIP_Instruction"() -> (w2864:string[][])
            n1929 = Index Array(array=w2864, index (row)=4, index (col)=25 ("disabled index (col)")) -> (element=w2861:string)
            n1930 = global write "Global_usbComm.vi" "FINISH-25"(w2861) -> ()
          }
          frame 3 {
            n1931 = global read "Global_usbComm.vi" "PIP_Instruction"() -> (w2868:string[][])
            n1932 = Index Array(array=w2868, index (row)=3, index (col)=25 ("disabled index (col)")) -> (element=w2865:string)
            n1933 = global write "Global_usbComm.vi" "FINISH-25"(w2865) -> ()
          }
          frame 4 {
            n1934 = global read "Global_usbComm.vi" "PIP_Instruction"() -> (w2872:string[][])
            n1935 = Index Array(array=w2872, index (row)=1, index (col)=25 ("disabled index (col)")) -> (element=w2869:string)
            n1936 = global write "Global_usbComm.vi" "FINISH-25"(w2869) -> ()
          }
        }
        "FINISH-25" <- w2849
        n1937 = while {
          tunnel: [T1."Another" ("Tab Control")] -> w2854
          stop <- "FIN0" stop-if-true
        }
      }
    }
  }
